vi "Results_file_Plotter.vi"() -> ()   [LabVIEW 2010]
uses:
  Anemometry/Anemometry Sub Vis/Data_plotting_vis/Plot_Slice.ctl
  Anemometry/Anemometry Sub Vis/Data_plotting_vis/Plotter_Mode.ctl
  Anemometry/Anemometry Sub Vis/Data_plotting_vis/Data_File_Type.ctl
  Anemometry/Anemometry Sub Vis/File/Setup_Filetype.ctl
  Anemometry/Anemometry Sub Vis/Controls/Global_mode.ctl
  Anemometry/Anemometry Sub Vis/Data_plotting_vis/Results_plotter_Global.vi
  Anemometry/Anemometry Sub Vis/Globals/Trav_pos_global.vi
  Anemometry/Anemometry Sub Vis/Globals/Constants_global.vi
  Instance           1 28Saved   Results_file_Plotter .vi
panel:
  in  "Single Series":i32[](listbox)=[0]
  out "Uadvec":dbl
  in  "Bkgnd Value":dbl
  in  "Update":bool
  in  "Full_Res_Results_Folder":path
  out "Last used Template":path
  out "Cursor index":i32
  in  "Plot Resolution":bool
  out "Choosen Path":path
  out "XY Plot":cluster{dbl[], dbl[]}[](graph)
  in  "VI Refnum Calculation":refnum<vi>
  in  "Save Plot as jpg":bool
  out "Edit Raw Data Header Info":bool
  out "Raw DF in Orig Pos?":bool
  out "Edit Raw DF?":bool
  out "Filetype":string[](array[string])
  out "Mode":T1
  out "Plotted rows only?":bool
  in  "type specifier VI Refnum (for type only) 2":refnum<vi>
  out "Warning!":string
  in  "Edit Template File":bool
  in  "type specifier VI Refnum (for type only)":refnum<vi>
  in  "color and symbol":bool
  out "No Of Rows":i32
  in  "Filter Bins 2":i32[](listbox)=[0]
  in  "Filter 6":u16(ring)
  in  "Filter 5":u16(ring)
  in  "Filter 4":u16(ring) items=["Show All (1216)", "10 (200)", "11 (4)", "13 (4)", "16 (4)", "17 (4)", "20 (12)", "23 (4)", "25 (4)", "28 (4)", "29 (4)", "30 (4)", "31 (4)", "35 (4)", "37 (4)", "38 (4)", "40 (8)", "44 (4)", "45 (8)", "47 (4)", "49 (4)", "50 (192)", "51 (4)", "53 (8)", "54 (4)", "56 (4)", "60 (12)", "63 (4)", "65 (4)", "67 (4)", "71 (8)", "72 (4)", "75 (4)", "78 (4)", "79 (4)", "81 (4)", "82 (4)", "85 (4)", "87 (4)", "90 (12)", "94 (4)", "97 (12)", "99 (4)", "100 (188)", "101 (8)", "103 (4)", "104 (4)", "106 (8)", "110 (4)", "111 (4)", "112 (4)", "115 (4)", "116 (4)", "119 (4)", "121 (8)", "125 (4)", "126 (4)", "128 (8)", "134 (12)", "137 (4)", "139 (4)", "141 (4)", "143 (4)", "144 (4)", "146 (8)", "148 (8)", "149 (4)", "150 (188)", "151 (4)", "153 (8)", "155 (4)", "156 (8)", "160 (4)", "162 (4)", "163 (4)", "164 (4)", "165 (4)", "171 (8)", "172 (4)", "173 (4)", "178 (8)", "181 (4)", "182 (4)", "185 (8)", "191 (8)", "193 (8)", "200 (16)"]
  in  "Filter 3":u16(ring) items=["Show All (1216)", "92 (1216)", "NOT 92 (0)"]
  in  "Filter Array":u16[](array[ring])=[0, 0, 0, 0, 0, 0] items=["Don't Filter", "Filename", "Case", "Roof Height", "Tank Height", "Release Angle", "X", "Y", "Z", "Y (FFID2)", "Z (FFID2)", "Mean Concentration (C)", "Variance in Concentration (C)", "Mean Concentration (C0)", "Variance in Concentration (C0)", "Standard Error in Mean C", "Background Mean Concentration", "Variance in Background Concentration", "CU/Q", "CU/Q err", "x/H", "y/H", "z/H", "Qtrace", "Uref", "Flow Measurement Time", "Seconds since 1st Jan", "Atmos Pressure Used for Corrections", "Current File Number", "Correlation coefficient", "Calib File", "Correlation", "Emission Rate", "Raw Data Filename"]
  in  "Filter Bins 1":i32[](listbox)=[0]
  in  "Tab Control":T2(tab)=enum."Save "
  in  "Reload Files":bool
  in  "Template":path
  in  "Empty":bool
  in  "Result files to read":path[](array[path])
  in  "Add results file":bool
  in  "File Tyoes to Read":T3
  in  "Vector Plot?":bool
  in  "Ordinate Name":string
  out "2nd Add label":string
  out "First Add label":string
  in  "Additional X Values":dbl[](array[numeric]) format="%.2f"
  in  "Additional Y Values":dbl[](array[numeric]) format="%.2f"
  in  "Show Results Space Analysis":bool
  in  "Show Plot Space Analysis":bool
  in  "Multi Ordinate":i32[](listbox)
  in  "Multi Ordinate?":bool
  in  "Ordinate":u16(ring) items=["Filename", "Case", "Roof Height", "Tank Height", "Release Angle", "X", "Y", "Z", "Y (FFID2)", "Z (FFID2)", "Mean Concentration (C)", "Variance in Concentration (C)", "Mean Concentration (C0)", "Variance in Concentration (C0)", "Standard Error in Mean C", "Background Mean Concentration", "Variance in Background Concentration", "CU/Q", "CU/Q err", "x/H", "y/H", "z/H", "Qtrace", "Uref", "Flow Measurement Time", "Seconds since 1st Jan", "Atmos Pressure Used for Corrections", "Current File Number", "Correlation coefficient", "Calib File", "Correlation", "Emission Rate", "Raw Data Filename"]
  in  "Intensity Plot?":bool
  in  "Absisca":u16(ring) items=["Filename", "Case", "Roof Height", "Tank Height", "Release Angle", "X", "Y", "Z", "Y (FFID2)", "Z (FFID2)", "Mean Concentration (C)", "Variance in Concentration (C)", "Mean Concentration (C0)", "Variance in Concentration (C0)", "Standard Error in Mean C", "Background Mean Concentration", "Variance in Background Concentration", "CU/Q", "CU/Q err", "x/H", "y/H", "z/H", "Qtrace", "Uref", "Flow Measurement Time", "Seconds since 1st Jan", "Atmos Pressure Used for Corrections", "Current File Number", "Correlation coefficient", "Calib File", "Correlation", "Emission Rate", "Raw Data Filename"]
  in  "Job Directory":path
  in  "Save Averaged rows":bool
  in  "Create picture Vi Name":string="Intensity plot jpg.vi"
  in  "Save Surface Fit":bool
  in  "Output Filename":path
  in  "Save Data in Rows":bool
  in  "Save Plot data":bool
  in  "Process Point":bool
  in  "Kill Point":bool
  out "Table":string[][](table)
  in  "Post Process Plotted Data":bool
  in  "Calculate Routine":string="Intensity plot jpg.vi"
  in  "Calculate new metadata":bool
  in  "Add /Edit metadata":bool
  in  "Delete Plotted data from file":bool
  in  "Save Setup":bool
  in  "Load Setup":bool
  in  "Point Size":i32(slide) scale=0.0..10.0
  in  "No of Contours":i32=20
  out "Accept Array":bool[][](array[boolean])
  out "Previous slice mode":T4
  out "Slice mode Change?":bool
  in  "Slice mode":T4
  in  "Z Ch Name":u16(ring) items=["Filename", "Case", "Roof Height", "Tank Height", "Release Angle", "X", "Y", "Z", "Y (FFID2)", "Z (FFID2)", "Mean Concentration (C)", "Variance in Concentration (C)", "Mean Concentration (C0)", "Variance in Concentration (C0)", "Standard Error in Mean C", "Background Mean Concentration", "Variance in Background Concentration", "CU/Q", "CU/Q err", "x/H", "y/H", "z/H", "Qtrace", "Uref", "Flow Measurement Time", "Seconds since 1st Jan", "Atmos Pressure Used for Corrections", "Current File Number", "Correlation coefficient", "Calib File", "Correlation", "Emission Rate", "Raw Data Filename"]
  in  "Y Ch Name":u16(ring) items=["Filename", "Case", "Roof Height", "Tank Height", "Release Angle", "X", "Y", "Z", "Y (FFID2)", "Z (FFID2)", "Mean Concentration (C)", "Variance in Concentration (C)", "Mean Concentration (C0)", "Variance in Concentration (C0)", "Standard Error in Mean C", "Background Mean Concentration", "Variance in Background Concentration", "CU/Q", "CU/Q err", "x/H", "y/H", "z/H", "Qtrace", "Uref", "Flow Measurement Time", "Seconds since 1st Jan", "Atmos Pressure Used for Corrections", "Current File Number", "Correlation coefficient", "Calib File", "Correlation", "Emission Rate", "Raw Data Filename"]
  in  "X Ch Name":u16(ring) items=["Filename", "Case", "Roof Height", "Tank Height", "Release Angle", "X", "Y", "Z", "Y (FFID2)", "Z (FFID2)", "Mean Concentration (C)", "Variance in Concentration (C)", "Mean Concentration (C0)", "Variance in Concentration (C0)", "Standard Error in Mean C", "Background Mean Concentration", "Variance in Background Concentration", "CU/Q", "CU/Q err", "x/H", "y/H", "z/H", "Qtrace", "Uref", "Flow Measurement Time", "Seconds since 1st Jan", "Atmos Pressure Used for Corrections", "Current File Number", "Correlation coefficient", "Calib File", "Correlation", "Emission Rate", "Raw Data Filename"]
  out "Filter 2 Strings":string[](array[string])
  out "Filter 1 Strings":string[](array[string])
  out "Ordinate Strings":string[](array[string])
  out "Non-Blank Rows":bool[](array[boolean])
  out "File Index":i32
  in  "Resolution":dbl=1.0 min=0.0 format="%.4f"
  out "Intensity Graph":dbl[][](graph)
  out "Tolerances":dbl[](array[numeric]) format="%.2f"
  in  "Results files choosen":path[](array[path])
  in  "Header":string
  out "Current":string="Graph Scales"
  in  "Transpose":bool
  out "Plotted Series":bool[][](array[boolean])
  in  "Results file":path
  in  "stop":bool
  out "Surface Area":dbl format="%.2f"
  out "Surface Integral":dbl format="%.4f"
  out "Surface Average":dbl format="%#.5f"
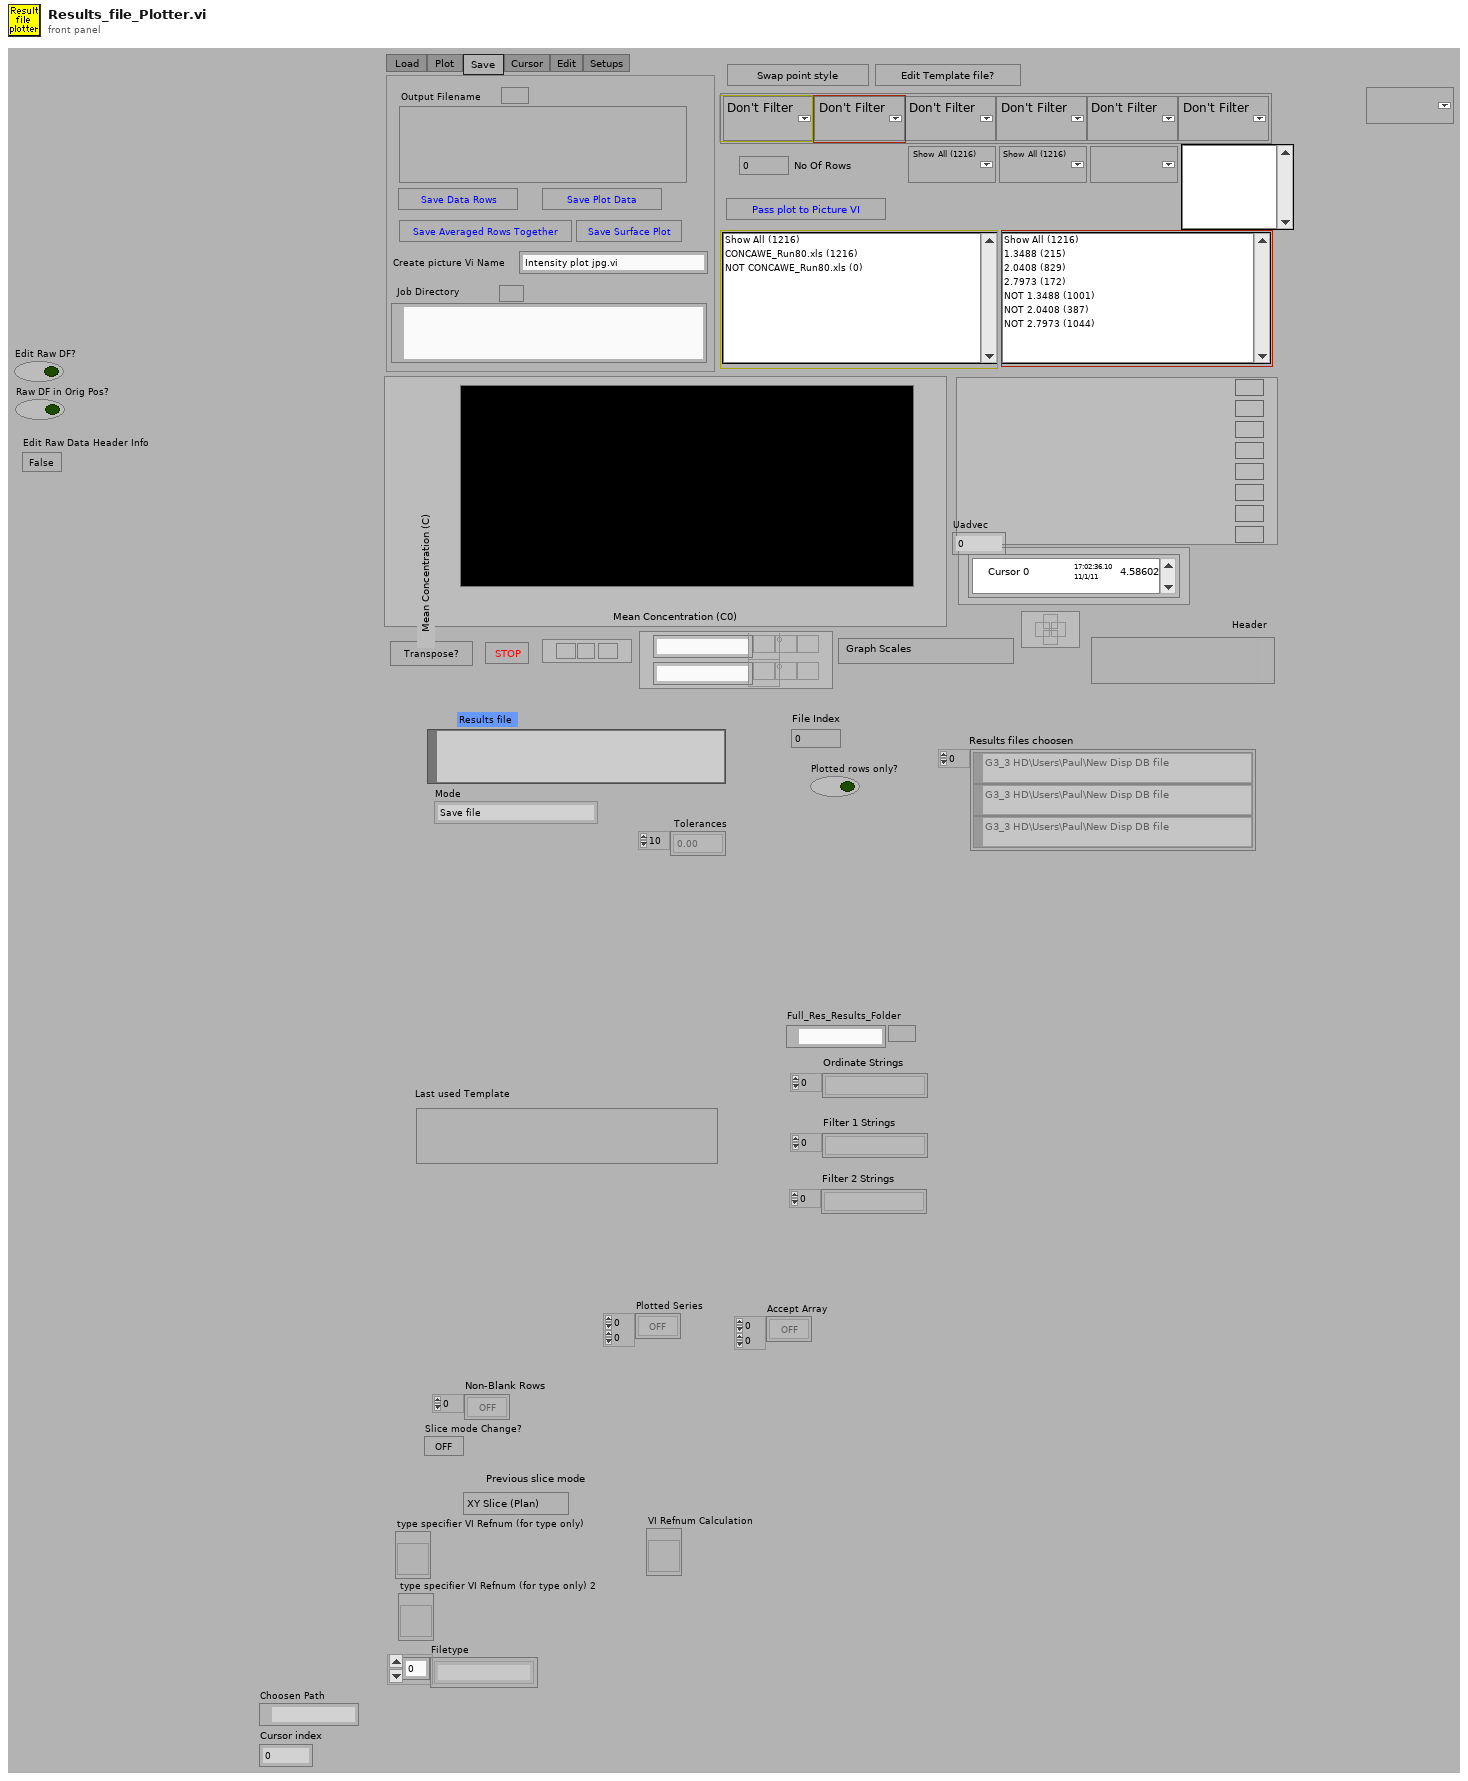
[diagram p1: front panel]
types:
  T1 = typedef "Plotter_Mode.ctl" = enum16{"Save file", "Delete unwanted rows", "Edit Values with constants", "Edit values per row", "Edit Raw Data file header", "Post Process Plotted Rows"}
  T2 = enum32{"Load ", "Plot ", "Save ", "Cursor", "Edit", "Setups"}
  T3 = typedef "Data_File_Type.ctl" = enum16{"Read All File Types", "Results Files Only", "Raw Data Files Only", "Calibration Files Only", "Gas Desk Files Only", "Old Results Files Only", "Tabulated Data Files Only"}
  T4 = typedef "Plot_Slice.ctl" = enum16{"XY Slice (Plan)", "YX Slice (Plan)", "YZ Slice (Cross)", "ZY Slice (Cross)", "XZ Slice (Side)", "ZX Slice (Side)"}
  T5 = typedef "Setup_Filetype.ctl" = enum16{"Measurement Setups", "Calibration Setups", "General", "Results File Plotter Setups", "Speed Calib Tweaks"}
  T6 = enum16{"Zero or one", "One", "Zero or more", "One or more"}
  T7 = typedef "Global_mode.ctl" = enum16{"Read Global", "Load Global From File", "Write Global to File"}
  T8 = enum16{"Edit Existing Template File", "Create New Template File"}
  T9 = enum16{"Show only data summary", "Show data summary", "No data summary"}
  T10 = typedef "All_Setup.ctl" = cluster{"Result files to read":path[], "Template":path, "Transpose":bool, "Additional X Values":dbl[], "Additional Y Values":dbl[], "Ordinate":u16, "Absisca":u16, "Filter Array":u16[], "color and symbol":bool, "Output Filename":path, "Jpg Vi Name":string, "Intensity Plot?":bool, "Multi Ordinate?":bool, "Filter Bins 1":i32[], "Filter Bins 2":i32[], "Multi Ordinate":i32[]}
  T11 = enum16{"Left Button", "Center Button", "Right Button", "Window Close"}
  T12 = enum32{"existing file", "new file", "new or existing file", "existing dir", "new dir", "new or existing dir", "existing file (use LLBs)", "new file (use LLBs)", "new or existing file (use LLBs)", "new or existing file or directory (use LLBs)"}
  T13 = cluster{"Plot Color":u32, "Plot Interpolation":u8, "Point Style":u8, "Line Style":u8, "Fill/Pt. Color":u32, "Line Width":u8, "Bar Plot Style":u8, "Fill To":i16}[]
  T14 = typedef "Group_Binning.ctl" = cluster{"Index":i32, "Tolerance":dbl, "Precision":string}
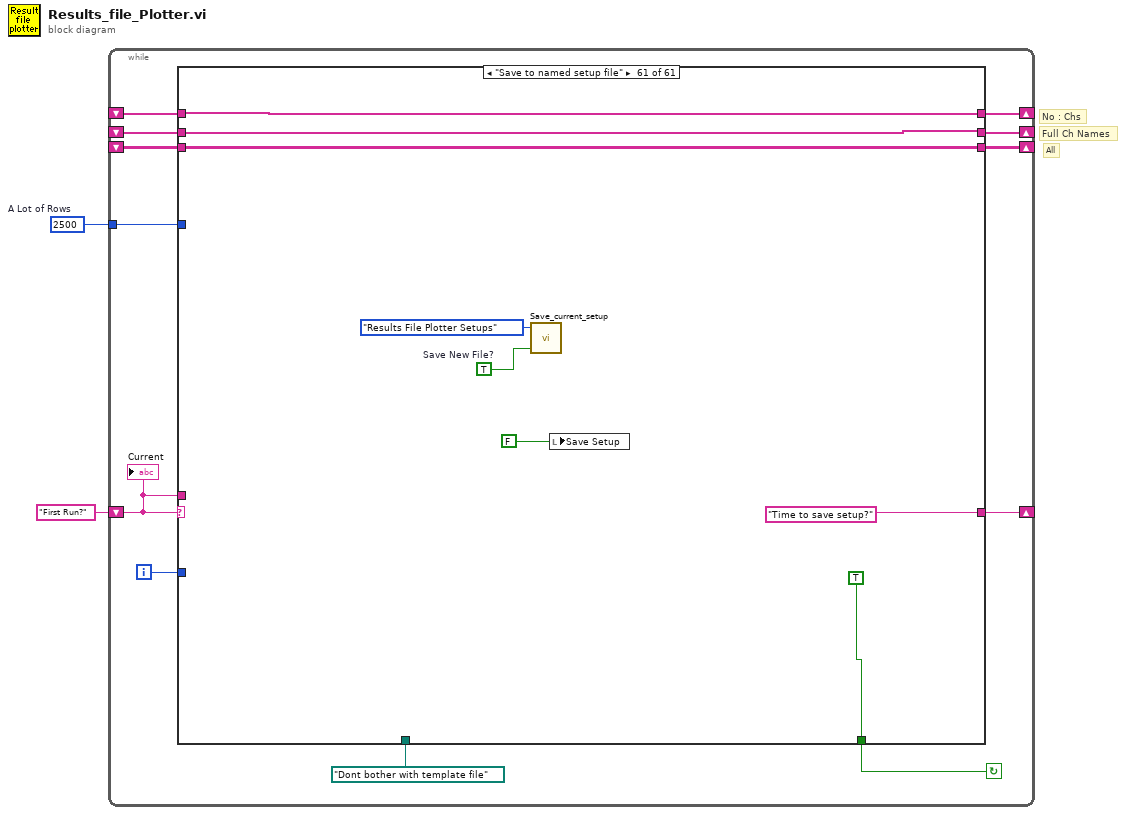
[diagram p0: block diagram]
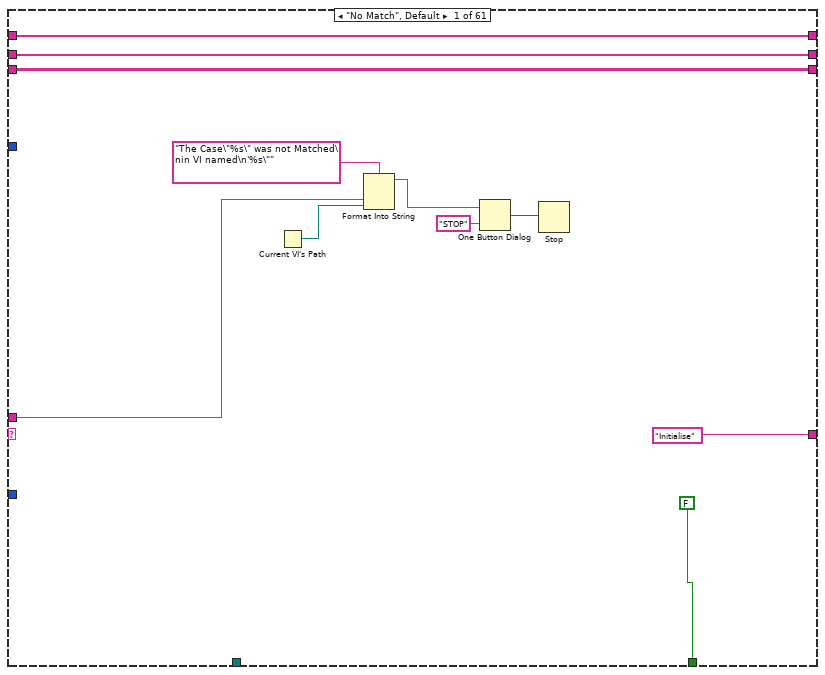
[diagram p2: hidden frame]
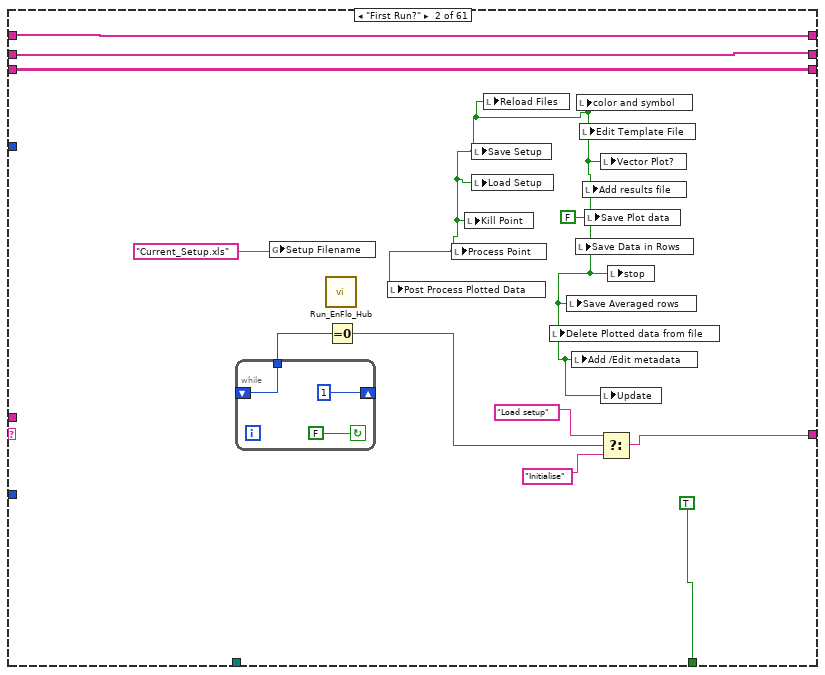
[diagram p3: hidden frame]
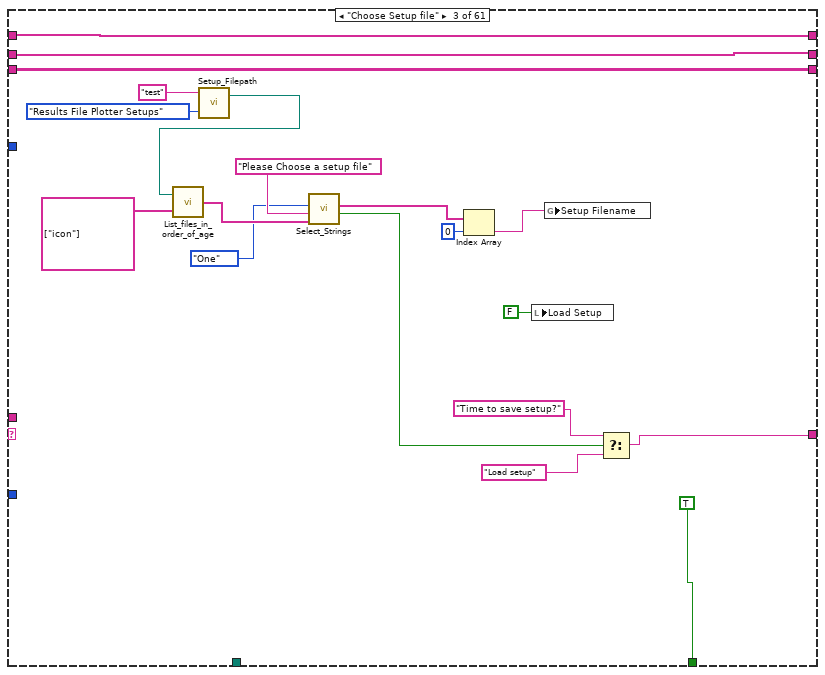
[diagram p4: hidden frame]
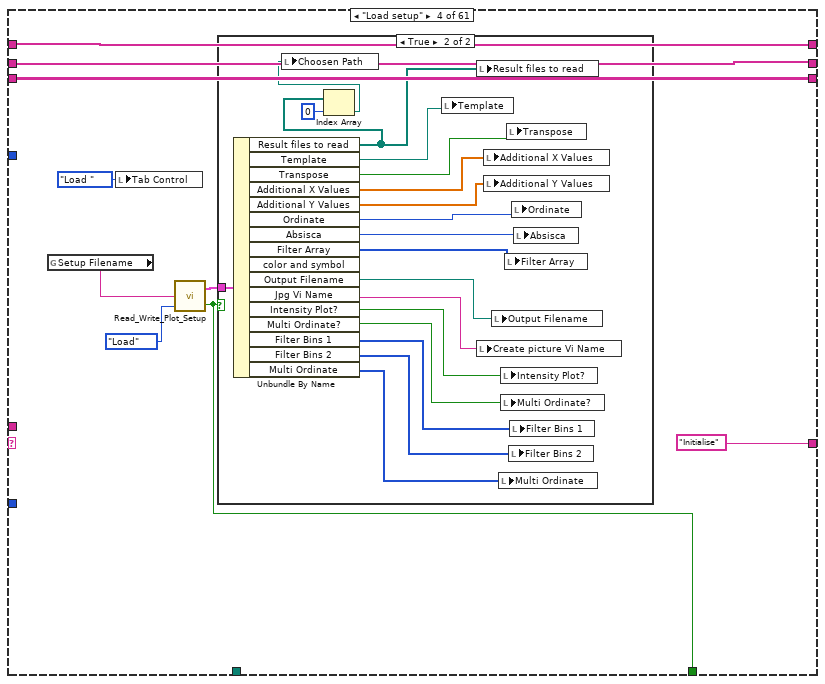
[diagram p5: hidden frame]
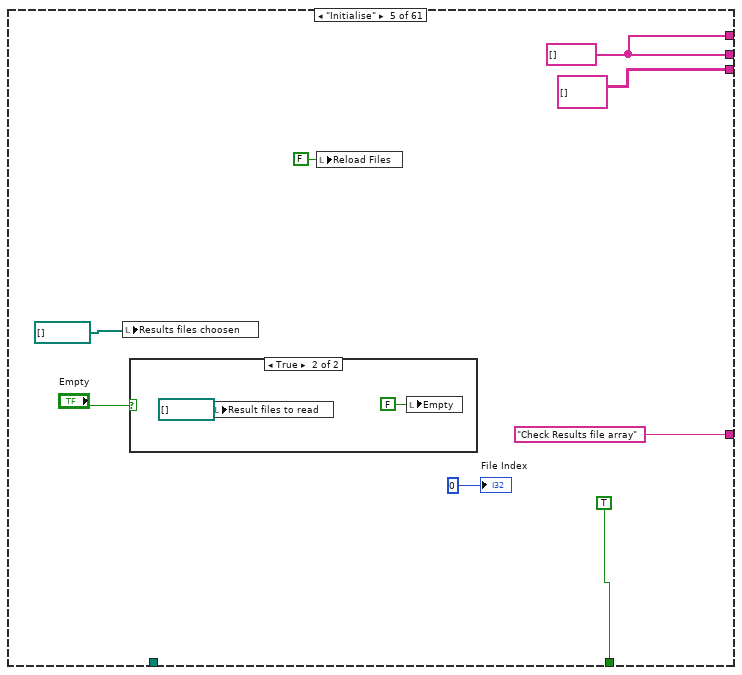
[diagram p7: hidden frame]
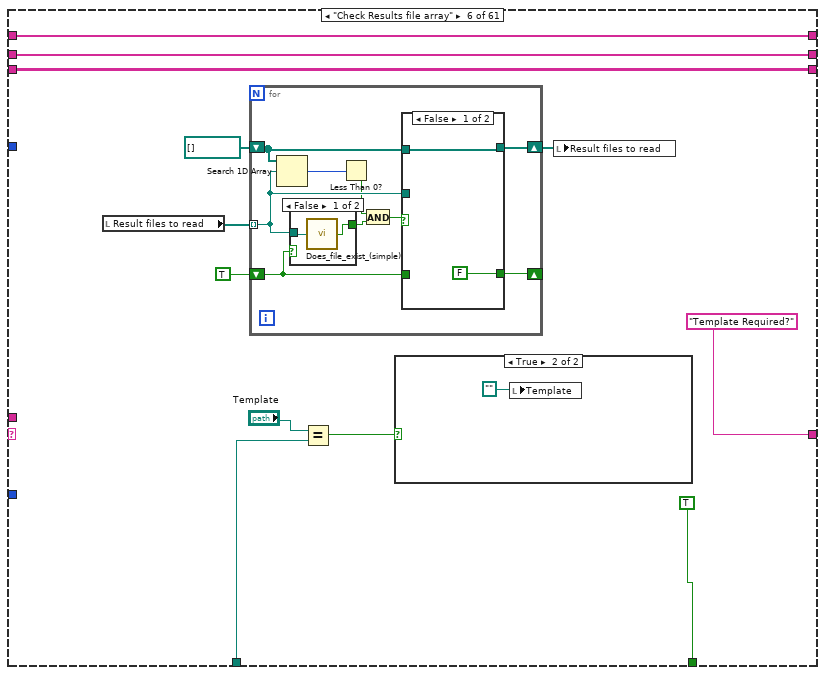
[diagram p9: hidden frame]
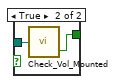
[diagram p11: hidden frame]
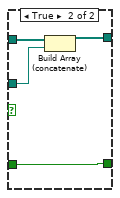
[diagram p12: hidden frame]
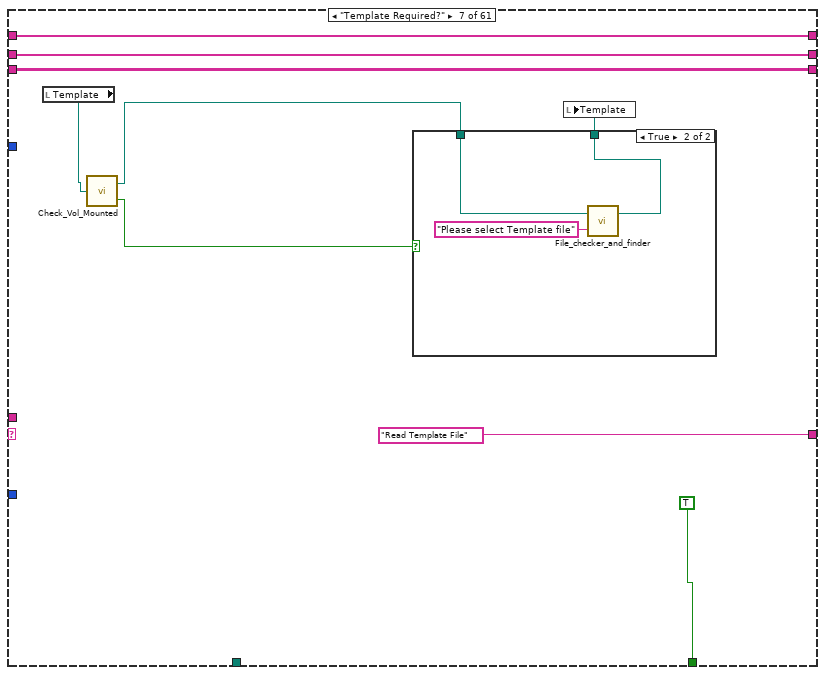
[diagram p13: hidden frame]
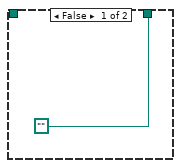
[diagram p14: hidden frame]
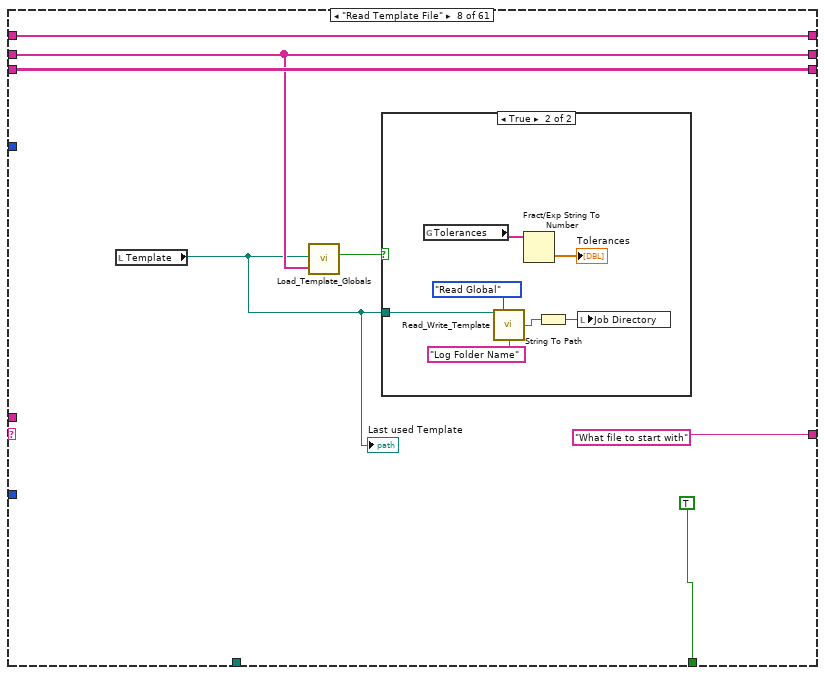
[diagram p15: hidden frame]
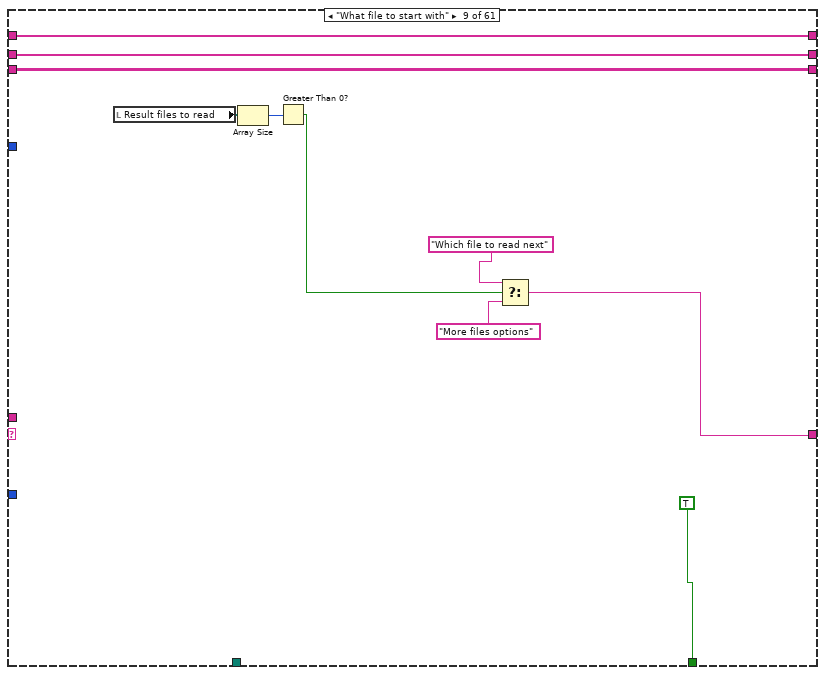
[diagram p17: hidden frame]
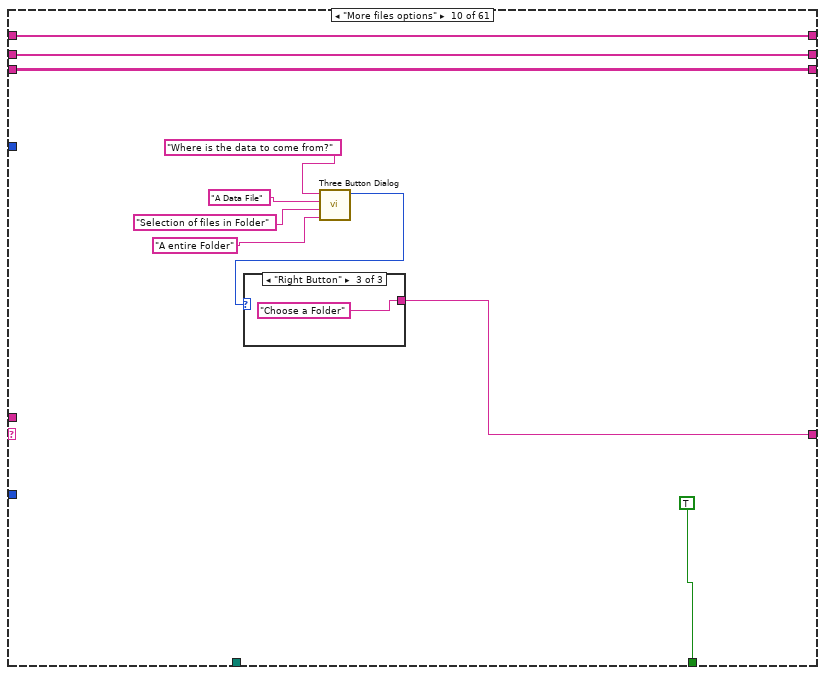
[diagram p18: hidden frame]
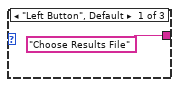
[diagram p19: hidden frame]
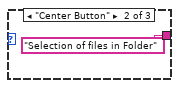
[diagram p20: hidden frame]
diagram:
  w1 = 2500  # A Lot of Rows
  # "No : Chs"
  # "Full Ch Names"
  # "All"
  n1 = while {
    shift-left: _ -> [w7]
    shift-right: [w8] -> _
    shift-left: "First Run?" -> [w11]
    shift-right: [w4] -> _
    shift-left: _ -> [w9]
    shift-right: [w14] -> _
    shift-left: _ -> [w12]
    shift-right: [w5] -> _
    tunnel: w1 -> [w3]
    i -> [w6]
    stop <- w13 continue-if-true
    n2 = case shown="\"Save to named setup file\"" w11 {
      tunnel: w9 -> [w25 w35 w57 w65 _ w106 w134 w143 w164 w174 w186 w200 w231 w258 w281 w403 w425 w451 w476 w502 w556 w570 w607 w909 w978 w1033 w1058 w1077 w1163 w1211 w1241 w1530 w1546 w1567 w1596 w1660 w1693 w1765 w1788 w1803 w1867 w1919 w1945 w2154 w2166 w2192 w2318 w2462 w2496 w2511 w2536 w2563 w2606 w2624 w2667 w2770 w2803 w3167 w3182 w3218 w3226]
      tunnel: [w25 w35 w57 w65 w91 w106 w134 w143 w164 w174 w186 w200 w231 w258 w279 w403 w425 w451 w476 w502 w556 w570 w607 w909 w978 w1033 w1058 w1077 w1163 w1211 w1239 w1530 w1546 w1567 w1596 w1660 w1693 w1765 w1788 w1803 w1867 w1919 w1943 w2154 w2166 w2190 w2311 w2462 w2496 w2511 w2536 w2563 w2606 w2624 w2667 w2770 w2803 w3167 w3182 w3218 w3226] -> w14
      tunnel: ["Initialise" w28 w52 "Initialise" ("t") "Check Results file array" ("t") "Template Required?" "Read Template File" "What file to start with" w155 w170 "Which file to read next" "Which file to read next" "Which file to read next" w254 w276 w394 "What is present?" "Ordinate Selector Type" w473 "Which rows are Non-Blank?" w549 "Create Selectors" w596 "Re Plot Data?" w973 "Prepare Filter2 strings" "Plot Data" w1074 "Add Axis names" "Analyse Plot Space" w1242 "What to do next?" "What to do next?" ("t") w1553 w1589 w1638 w1691 w1759 w1784 w1802 w1866 "Initialise" w1946 w2145 "Create Selectors" w2193 w2319 w2460 w2494 w2501 w2520 "Save XY plot as jpg" "Create Selectors" w2621 w2670 w2754 w2809 "Save Setup" ("t") "Initialise" ("t") w3187 "Time to save setup?"] -> w4
      tunnel: [FALSE TRUE TRUE w61 TRUE TRUE TRUE TRUE TRUE TRUE TRUE TRUE TRUE w249 w283 TRUE TRUE TRUE TRUE TRUE TRUE TRUE TRUE TRUE TRUE TRUE TRUE w1075 TRUE TRUE w1243 TRUE TRUE ("OK?") TRUE TRUE ("OK?") TRUE ("OK?") w1689 TRUE TRUE w1801 w1865 TRUE w1947 TRUE ("OK?") TRUE ("OK?") w2194 w2320 TRUE TRUE TRUE TRUE TRUE TRUE TRUE TRUE TRUE TRUE TRUE TRUE w3196 TRUE ("OK?")] -> w13
      tunnel: w12 -> [w24 w34 w56 w64 _ w105 w133 w145 w163 w173 w185 w199 w230 w257 w282 w399 w424 w452 w477 w503 w555 w568 w602 w911 w967 w1035 w1060 w1076 w1165 w1213 w1240 w1529 w1545 w1566 w1607 w1659 w1692 w1764 w1787 w1800 w1864 w1918 w1944 w2153 w2163 w2191 w2317 w2463 w2495 w2510 w2540 w2566 w2605 w2623 w2666 w2769 w2802 w3166 w3181 w3217 w3225]
      tunnel: w11 -> [w16 _ _ _ _ _ _ _ _ _ _ _ _ _ _ _ _ _ _ _ _ _ _ _ _ _ _ _ _ _ _ _ _ _ _ _ _ _ _ _ _ _ _ _ _ _ _ _ _ _ _ _ _ _ _ _ _ _ _ _ _]
      tunnel: path "Dont bother with template file" ("Template File") -> [_ _ _ _ _ w99 _ _ _ _ _ _ _ _ _ _ _ _ _ _ _ _ _ _ _ _ _ _ _ _ _ _ _ _ _ _ _ _ _ _ _ _ _ _ _ _ _ _ _ _ _ _ _ _ _ _ _ w3164 w3176 _ _]
      tunnel: [w15 w33 w55 w66 w91 w104 w132 w144 w161 w171 w183 w197 w228 w256 w278 w387 w423 w453 w475 w501 w547 w569 w600 w908 w969 w1025 w1053 w1073 w1157 w1206 w1235 w1526 w1547 w1565 w1597 w1661 w1694 w1763 w1786 w1799 w1863 w1917 w1937 w2155 w2171 w2181 w2314 w2472 w2497 w2512 w2537 w2564 w2607 w2625 w2671 w2771 w2810 w3168 w3183 w3219 w3227] -> w8
      tunnel: w7 -> [w15 w33 w55 w66 _ w104 w132 w144 w161 w171 w183 w197 w228 w256 w277 w387 w423 w453 w475 w501 w547 w569 w600 w908 w969 w1025 w1053 w1073 w1157 w1206 w1234 w1526 w1547 w1565 w1597 w1661 w1694 w1763 w1786 w1799 w1863 w1917 w1936 w2155 w2171 w2185 w2313 w2472 w2497 w2512 w2537 w2564 w2607 w2625 w2671 w2771 w2810 w3168 w3183 w3219 w3227]
      tunnel: w6 -> [_ _ _ _ _ _ _ _ _ _ _ _ _ _ _ _ _ _ _ _ _ _ _ _ _ _ _ _ _ _ _ _ _ _ _ _ w1690 _ _ _ _ _ _ _ _ _ _ _ _ _ _ _ _ _ _ _ _ _ _ _ _]
      tunnel: [w24 w34 w56 w64 string[][] [] w105 w133 w145 w163 w173 w185 w199 w230 w257 w280 w399 w424 w452 w477 w503 w555 w568 w602 w911 w967 w1035 w1060 w1076 w1165 w1213 w1238 w1529 w1545 w1566 w1607 w1659 w1692 w1764 w1787 w1800 w1864 w1918 w1942 w2153 w2163 w2189 w2310 w2463 w2495 w2510 w2540 w2566 w2605 w2623 w2666 w2769 w2802 w3166 w3181 w3217 w3225] -> w5
      tunnel: w3 -> [_ _ _ _ _ _ _ _ _ _ _ _ _ _ _ _ _ _ _ _ _ _ _ _ _ _ _ _ _ _ _ _ _ _ _ _ _ _ w1782 _ w1862 _ _ _ _ _ _ _ _ _ _ _ _ w2620 w2664 _ w2800 _ _ _ _]
      frame "No Match", Default {
        n3 = Current VI's Path() -> (path=w17:path)
        n4 = Format Into String(format string="The Case\"%s\" was not Matched\nin VI named\n'%s\"" ("Format String"), w16, w17) -> (resulting string=w20:string)  [unwired: 2 in, 1 out]
        n5 = One Button Dialog(message=w20, button name ("OK")="STOP") -> (true=w18:bool)
        n6 = Stop(stop? (T)=w18) -> ()
      }
      frame "First Run?" {
        w26 = FALSE ("Save Plot data")
        n7 = while {
          shift-right: [1] -> _
          shift-left: _ -> [w38]
          tunnel: [w38] -> w30
          stop <- FALSE continue-if-true
        }
        n8 = global write "Results_plotter_Global.vi" "Setup Filename"("Current_Setup.xls" ("Setup filename")) -> ()
        n9 = call "Run_EnFlo_Hub.vi"() -> ()  [unwired: 8 out]
        n10 = Equal To 0?(x=w30) -> (x = 0?=w29:bool)
        n11 = local write "Post Process Plotted Data"(w26) -> ()
        n12 = local write "Process Point"(w26) -> ()
        n13 = local write "Kill Point"(w26) -> ()
        n14 = local write "Save Setup"(w26) -> ()
        n15 = local write "Load Setup"(w26) -> ()
        n16 = local write "Reload Files"(w26) -> ()
        n17 = local write "Delete Plotted data from file"(w26) -> ()
        n18 = local write "Save Averaged rows"(w26) -> ()
        n19 = local write "Add /Edit metadata"(w26) -> ()
        n20 = local write "Save Data in Rows"(w26) -> ()
        n21 = local write "color and symbol"(w26) -> ()
        n22 = local write "Edit Template File"(w26) -> ()
        n23 = local write "Add results file"(w26) -> ()
        n24 = local write "Save Plot data"(w26) -> ()
        n25 = local write "Vector Plot?"(w26) -> ()
        n26 = local write "Update"(w26) -> ()
        n27 = Select(t="Load setup", s=w29, f="Initialise") -> (s? t:f=w28:string)
        n28 = local write "stop"(w26) -> ()
      }
      frame "Choose Setup file" {
        n29 = call "Setup_Filepath.vi"("Setup File Type"=Setup_Filetype."Results File Plotter Setups", "Filename in"="test") -> ("Directory"=w40:path)  [unwired: 1 out]
        n30 = call "List_files_in_order_of_age.vi"("Files to Hide"=string[] ["icon"], "Folder"=w40) -> ("file names"=w51:string[])
        n31 = call "Select_Strings.vi"("Available Ch names"=w51, "Message"="Please Choose a setup file", "Selector mode"=T6."One") -> ("Cancel"=w45:bool, "Selected Channel Names"=w48:string[])  [unwired: 1 in, 3 out]
        n32 = Index Array(array=w48, index=0) -> (element=w46:string)
        n33 = local write "Load Setup"(FALSE ("Save Setup")) -> ()
        n34 = global write "Results_plotter_Global.vi" "Setup Filename"(w46) -> ()
        n35 = Select(t="Time to save setup?", s=w45, f="Load setup") -> (s? t:f=w52:string)
      }
      frame "Load setup" {
        n36 = global read "Results_plotter_Global.vi" "Setup Filename"() -> (w60:string)
        n37 = local write "Tab Control"(T2."Load " ("Tab Control")) -> ()
        n38 = call "Read_Write_Plot_Setup.vi"("Mode"=enum16{"Load", "Save"}."Load", "Setup filename"=w60) -> ("OK?"=w61:bool, "Cluster 2"=w62:T10)  [unwired: 1 in]
        n39 = case shown="True" w61 {
          tunnel: w62 -> [_ w85]
          frame False {
          }
          frame True {
            n40 = Unbundle By Name(w85) -> ("Result files to read"=w70:path[], "Template"=w68:path, "Transpose"=w75:bool, "Additional X Values"=w76:dbl[], "Additional Y Values"=w77:dbl[], "Ordinate"=w78:u16, "Absisca"=w79:u16, "Filter Array"=w80:u16[], "Output Filename"=w81:path, "Jpg Vi Name"=w82:string, "Intensity Plot?"=w83:bool, "Multi Ordinate?"=w84:bool, "Filter Bins 1"=w74:i32[], "Filter Bins 2"=w73:i32[], "Multi Ordinate"=w72:i32[])  [unwired: 1 out]
            n41 = Index Array(array=w70, index=0) -> (element=w69:path)
            n42 = local write "Choosen Path"(w69) -> ()
            n43 = local write "Template"(w68) -> ()
            n44 = local write "Result files to read"(w70) -> ()
            n45 = local write "Create picture Vi Name"(w82) -> ()
            n46 = local write "Additional X Values"(w76) -> ()
            n47 = local write "Additional Y Values"(w77) -> ()
            n48 = local write "Output Filename"(w81) -> ()
            n49 = local write "Multi Ordinate"(w72) -> ()
            n50 = local write "Intensity Plot?"(w83) -> ()
            n51 = local write "Multi Ordinate?"(w84) -> ()
            n52 = local write "Filter Array"(w80) -> ()
            n53 = local write "Transpose"(w75) -> ()
            n54 = local write "Filter Bins 2"(w73) -> ()
            n55 = local write "Filter Bins 1"(w74) -> ()
            n56 = local write "Ordinate"(w78) -> ()
            n57 = local write "Absisca"(w79) -> ()
          }
        }
      }
      frame "Initialise" {
        w91 = string[] [] ("Channel names")
        n58 = local write "Results files choosen"(path[] [] ("Results file choosen")) -> ()
        n59 = case shown="True" "Empty" {
          frame False {
          }
          frame True {
            n60 = local write "Result files to read"(path[] [] ("Result files to read")) -> ()
            n61 = local write "Empty"(FALSE ("Empty")) -> ()
          }
        }
        n62 = local write "Reload Files"(FALSE ("Reload Files")) -> ()
        "File Index" <- 0
      }
      frame "Check Results file array" {
        n63 = local read "Result files to read"() -> (w103:path[])
        n64 = for {
          shift-right: [w117] -> w101
          shift-left: path[] [] -> [w116]
          tunnel: w103 -> [w115] mode=indexing
          shift-right: [w110] -> _
          shift-left: TRUE -> [w109]
          n65 = Search 1D Array(1D array=w116, element=w115) -> (index of element=w114:i32)  [unwired: 1 out]
          n66 = case shown="False" w109 {
            tunnel: w115 -> [w119 w121]
            tunnel: [w118 w120] -> w112
            frame False {
              n67 = call "Does_file_exist_(simple).vi"("Pathname"=w119) -> ("exists?"=w118:bool)
            }
            frame True {
              n68 = call "Check_Vol_Mounted.vi"("Filename"=w121) -> ("exists?"=w120:bool)  [unwired: 1 out]
            }
          }
          n69 = Less Than 0?(x=w114) -> (x < 0?=w111:bool)
          n70 = And(x=w111, y=w112) -> (x .and. y?=w113:bool)
          n71 = case shown="False" w113 {
            tunnel: w116 -> [w123 w127]
            tunnel: w115 -> [_ w126]
            tunnel: [w123 w125] -> w117
            tunnel: [FALSE w124] -> w110
            tunnel: w109 -> [_ w124]
            frame False {
            }
            frame True {
              n72 = Build Array (concatenate)(w127, w126) -> (w125:path[])
            }
          }
        }
        n73 = Equal?(x="Template", y=w99) -> (x = y?=w98:bool)
        n74 = case shown="True" w98 {
          frame False {
          }
          frame True {
            n75 = local write "Template"(path "") -> ()
          }
        }
        n76 = local write "Result files to read"(w101) -> ()
      }
      frame "Template Required?" {
        n77 = local read "Template"() -> (w131:path)
        n78 = call "Check_Vol_Mounted.vi"("Filename"=w131) -> ("Filename Out"=w130:path, "exists?"=w129:bool)
        n79 = case shown="True" w129 {
          tunnel: w130 -> [_ w139]
          tunnel: [path "" w138] -> w128
          frame False {
          }
          frame True {
            n80 = call "File_checker_and_finder.vi"("Promp if not found"="Please select Template file", "Filename In"=w139) -> ("Filename Out"=w138:path)  [unwired: 1 out]
          }
        }
        n81 = local write "Template"(w128) -> ()
      }
      frame "Read Template File" {
        n82 = local read "Template"() -> (w141:path)
        "Last used Template" <- w141
        n83 = call "Load_Template_Globals.vi"("Channel Names"=w143, "Template-read"=w141) -> ("Valid Template File?"=w142:bool)
        n84 = case shown="True" w142 {
          tunnel: w141 -> [_ w149]
          frame False {
          }
          frame True {
            n85 = global read "Results_plotter_Global.vi" "Tolerances"() -> (w153:string[])
            n86 = call "Read_Write_Template.vi"("Template File"=w149, "Mode"=Global_mode."Read Global", "Data type"="Log Folder Name" ("Variable name")) -> ("Single Value Out"=w151:string)  [unwired: 5 in, 7 out]
            n87 = Fract/Exp String To Number(string=w153) -> (number=→"Tolerances":dbl[])  [unwired: 4 out]
            n88 = String To Path(string=w151) -> (path=w148:path)
            n89 = local write "Job Directory"(w148) -> ()
          }
        }
      }
      frame "What file to start with" {
        n90 = local read "Result files to read"() -> (w160:path[])
        n91 = Array Size(array=w160) -> (size(s)=w159:i32)
        n92 = Greater Than 0?(x=w159) -> (x > 0?=w156:bool)
        n93 = Select(t="Which file to read next", s=w156, f="More files options") -> (s? t:f=w155:string)
      }
      frame "More files options" {
        n94 = call <vilib>:"Three Button Dialog.vi"("Right Button Text (\"Cancel\")"="A entire Folder" ("F button name (\"Cancel\")"), "Center Button Text (\"No\")"="Selection of files in Folder" ("T button name (\"OK\")"), "Left Button Text (\"Yes\")"="A Data File" ("T button name (\"OK\")"), "message"="Where is the data to come from?") -> ("Which Button?"=w169:T11)  [unwired: 1 in, 6 out]
        n95 = case shown="\"Right Button\"" w169 {
          tunnel: ["Choose Results File" "Selection of files in Folder" "Choose a Folder"] -> w170
          frame "Left Button", Default {
          }
          frame "Center Button" {
          }
          frame "Right Button" {
          }
        }
      }
      frame "Choose Results File" {
        (unwired) T12."existing file" ("select mode (2)")
        n96 = local read "Choosen Path"() -> (w178:path)
        n97 = File Dialog(7:"Please Choose a Results File" ("Promp if not found"), 11:w178) -> (1:w180:bool, 3:w179:path)  [unwired: 1 in, 6 out]
        "Choosen Path" <- w179
        n98 = case shown="False" w180 {
          tunnel: w179 -> [w187 _]
          frame False {
            n99 = local read "Result files to read"() -> (w188:path[])
            n100 = Build Array (concatenate)(w188, w187) -> (w189:path[])
            n101 = local write "Result files to read"(w189) -> ()
          }
          frame True {
          }
        }
      }
      frame "Choose a Folder" {
        n102 = local read "Choosen Path"() -> (w191:path)
        n103 = File Dialog(7:"Please Choose the folder that contains the Results files to be plotted" ("prompt"), 11:w191) -> (3:w190:path)  [unwired: 1 in, 7 out]
        n104 = local write "Choosen Path"(w190) -> ()
        n105 = call "Get_folder_and_filenames.vi"("file path (dialog if empty)"=w190) -> ("Files"=w192:path[])  [unwired: 1 out]
        n106 = for {
          shift-right: [w211] -> w193
          shift-left: "Result files to read" -> [w210]
          tunnel: w192 -> [w208] mode=indexing
          n107 = Search 1D Array(1D array=w210, element=w208) -> (index of element=w209:i32)  [unwired: 1 out]
          n108 = Strip Path(path=w208) -> (name=w207:string)  [unwired: 1 out]
          n109 = Less Than 0?(x=w209) -> (x < 0?=w206:bool)
          n110 = call "Add_filename_suffix.vi"("Filename"=w207) -> ("Original Suffix"=w204:string)  [unwired: 1 in, 3 out]
          n111 = call "Match_Pat_Case_In.vi"("String to match"=".jpg" ("x"), "String"=w204) -> ("offset past match"=w202:i32)  [unwired: 1 in, 3 out]
          n112 = Less Than 0?(x=w202) -> (x < 0?=w201:bool)
          n113 = And(x=w206, y=w201) -> (x .and. y?=w205:bool)
          n114 = case shown="True" w205 {
            tunnel: w210 -> [w212 w215]
            tunnel: w208 -> [_ w214]
            tunnel: [w212 w213] -> w211
            frame False {
            }
            frame True {
              n115 = Build Array (concatenate)(w215, w214) -> (w213:path[])
            }
          }
        }
        n116 = local write "Result files to read"(w193) -> ()
      }
      frame "Selection of files in Folder" {
        n117 = local read "Choosen Path"() -> (w217:path)
        n118 = local read "Result files to read"() -> (w220:path[])
        n119 = File Dialog(7:"Please Choose the folder that contains the Results files to be plotted" ("prompt"), 11:w217) -> (3:w216:path)  [unwired: 1 in, 7 out]
        n120 = local write "Choosen Path"(w216) -> ()
        n121 = call "Get_folder_and_filenames.vi"("file path (dialog if empty)"=w216) -> ("Files"=w222:path[])  [unwired: 1 out]
        n122 = for {
          tunnel: w222 -> [w245] mode=indexing
          tunnel: [w244] -> w225 mode=indexing
          n123 = Strip Path(path=w245) -> (name=w244:string)  [unwired: 1 out]
        }
        n124 = call "Select_Strings.vi"("Available Ch names"=w225, "Message"="Please select the desired data files", "Selector mode"=T6."Zero or more") -> ("Ch Indicies Choosen"=w223:i32[])  [unwired: 1 in, 4 out]
        n125 = for {
          tunnel: w223 -> [w243] mode=indexing
          tunnel: w222 -> [w242]
          tunnel: [w241] -> w218 mode=indexing
          n126 = Index Array(array=w242, index=w243) -> (element=w241:path)
        }
        n127 = for {
          shift-right: [w236] -> w219
          shift-left: w220 -> [w235]
          tunnel: w218 -> [w234] mode=indexing
          n128 = Search 1D Array(1D array=w235, element=w234) -> (index of element=w233:i32)  [unwired: 1 out]
          n129 = Less Than 0?(x=w233) -> (x < 0?=w232:bool)
          n130 = case shown="True" w232 {
            tunnel: w235 -> [w237 w240]
            tunnel: w234 -> [_ w239]
            tunnel: [w237 w238] -> w236
            frame False {
            }
            frame True {
              n131 = Build Array (concatenate)(w240, w239) -> (w238:path[])
            }
          }
        }
        n132 = local write "Result files to read"(w219) -> ()
      }
      frame "Which file to read next" {
        n133 = local read "Result files to read"() -> (w255:path[])
        n134 = local read "File Index"() -> (w252:i32)
        n135 = Array Size(array=w255) -> (size(s)=w253:i32)
        n136 = Equal?(x=w253, y=w252) -> (x = y?=w251:bool)
        n137 = case shown="True" w251 {
          tunnel: w255 -> [w261 _]
          tunnel: [w262 "Load Selectors"] -> w254
          tunnel: w252 -> [w260 w274]
          tunnel: [w259 w274] -> w247
          frame False {
            n138 = Index Array(array=w261, index=w260) -> (element=w263:path)
            n139 = Search 1D Array(1D array="Results files choosen", element=w263) -> (index of element=w265:i32)  [unwired: 1 out]
            n140 = local write "Results file"(w263) -> ()
            n141 = call "Add_filename_suffix.vi"() -> ()  [unwired: 2 in, 4 out]
            n142 = case shown="-1" w265 {
              tunnel: "Results files choosen" -> [_ w273]
              tunnel: w263 -> [w269 w272]
              tunnel: ["Which file to read next" "Load Data"] -> w262
              frame 0, Default {
                n143 = Format Into String(format string="The filename\n \"%s\"\n has already been choosen" ("Format String"), w269) -> (resulting string=w267:string)  [unwired: 2 in, 1 out]
                n144 = One Button Dialog(message=w267) -> ()  [unwired: 2 out]
              }
              frame -1 {
                n145 = Build Array (concatenate)(w273, w272) -> (w271:path[])
                n146 = local write "Results files choosen"(w271) -> ()
              }
            }
            n147 = Increment(x=w260) -> (x+1=w259:i32)
          }
          frame True {
          }
        }
        n148 = Decrement(x=w247) -> (x-1=w246:i32)
        n149 = Build Array(w246) -> (w248:i32[])
        n150 = local read "stop"() -> (w250:bool)
        n151 = local write "File Index"(w247) -> ()
        n152 = property on="Result files to read" class="Arr (strict)"("Index Values"=w248) -> ()  [unwired: 2 in, 2 out]
        n153 = Not(x=w250) -> (.not. x?=w249:bool)
      }
      frame "Load Data" {
        n154 = stacked-sequence {
          seq-local: [w288 _] -> [_ w348]
          seq-local: [w287 _] -> [_ w353]
          seq-local: [w286 _] -> [_ w352]
          seq-local: [w284 _] -> [_ w351]
          tunnel: [TRUE _] -> w283
          tunnel: w282 -> [w302 w354]
          tunnel: w281 -> [w301 _]
          tunnel: [w300 _] -> w280
          tunnel: [w299 _] -> w279
          tunnel: [w298 _] -> w278
          tunnel: w277 -> [w297 _]
          tunnel: ["Which file to read next" _] -> w276
          frame #0 {
            w291 = TRUE  # Add Extra Channels?
            n155 = local read "Template"() -> (w295:path)
            n156 = call "Read_Data_file.vi"("Results file"="Results file", "Add Extra Channels?"=w291, "Template File"=w295, "Desired File Types"="File Tyoes to Read") -> ("Row numbers"=w286:i32[], "Template File Out"=w292:path, "Filetype"=w287:string, "Results file Out"=w288:path, "Ch names Out"=w293:string[], "Channel Values Out"=w289:string[][])  [unwired: 1 in, 9 out]
            n157 = local write "Template"(w292) -> ()
            n158 = Array Size(array=w293) -> (size(s)=w294:i32)
            n159 = Greater Than 0?(x=w294) -> (x > 0?=w284:bool)
            n160 = case shown="True" w284 {
              tunnel: w302 -> [w305 w318]
              tunnel: w301 -> [w306 w310]
              tunnel: w289 -> [_ w308]
              tunnel: [w305 w311] -> w300
              tunnel: [w306 w316] -> w299
              tunnel: [w304 w315] -> w298
              tunnel: w297 -> [w304 _]
              tunnel: w293 -> [_ w309]
              frame False {
              }
              frame True {
                n161 = for {
                  tunnel: w308 -> [w320] mode=indexing
                  tunnel: [w319] -> w307 mode=indexing
                  n162 = for {
                    tunnel: w320 -> [w322] mode=indexing
                    tunnel: [w321] -> w319 mode=indexing
                    n163 = call "Fast_string_Replace.vi"("Replace match with:"="[", "Input String"=w322, "regular expression"="(") -> ("Output String"=w323:string)  [unwired: 2 out]
                    n164 = call "Fast_string_Replace.vi"("Replace match with:"="]", "Input String"=w323, "regular expression"=")") -> ("Output String"=w321:string)  [unwired: 2 out]
                  }
                }
                n165 = call "Merge_channel_names.vi"("Preferred Channel array"=w310, "Channel array"=w309) -> ("Merged Channels"=w316:string[], "Preferred Channels Changed?"=w313:bool, "Channel Array Changed?"=w314:bool)
                n166 = for {
                  tunnel: w316 -> [w345] mode=indexing
                  tunnel: [w342] -> w315 mode=indexing
                  n167 = call "Fast_string_Replace.vi"("Replace match with:"=" ", "Input String"=w345, "regular expression"=":") -> ("Output String"=w341:string)  [unwired: 2 out]
                  n168 = call "Fast_string_Replace.vi"("Replace match with:"=" ", "Input String"=w341, "regular expression"="  ") -> ("Output String"=w340:string)  [unwired: 2 out]
                  n169 = call <vilib>:"Trim Whitespace.vi"("string"=w340) -> ("trimmed string"=w342:string)  [unwired: 1 in]
                }
                n170 = case shown="True" w313 {
                  tunnel: w318 -> [w333 w335]
                  tunnel: w310 -> [_ w337]
                  tunnel: [w333 w334] -> w312
                  tunnel: w316 -> [_ w336]
                  frame False {
                  }
                  frame True {
                    n171 = call "Merge_2D_values.vi"("Values In"=w335, "Present Channels"=w337, "Desired Channels"=w336) -> ("Values Out"=w334:string[][])
                  }
                }
                n172 = case shown="True" w314 {
                  tunnel: [w328 w332] -> w317
                  tunnel: w309 -> [_ w331]
                  tunnel: w307 -> [w328 w330]
                  tunnel: w316 -> [_ w329]
                  frame False {
                  }
                  frame True {
                    n173 = call "Merge_2D_values.vi"("Values In"=w330, "Present Channels"=w331, "Desired Channels"=w329) -> ("Values Out"=w332:string[][])
                  }
                }
                n174 = Build Array (concatenate)(w312, w317) -> (w311:string[][])
              }
            }
          }
          frame #1 {
            n175 = local read "Result files to read"() -> (w347:path[])
            n176 = local read "File Index"() -> (w350:i32)
            n177 = Decrement(x=w350) -> (x-1=w349:i32)
            n178 = case shown="True" w351 {
              tunnel: w354 -> [_ w367]
              tunnel: w353 -> [_ w365]
              tunnel: w352 -> [_ w363]
              tunnel: w349 -> [w355 w361]
              tunnel: w348 -> [_ w360]
              tunnel: w347 -> [w357 w362]
              tunnel: [w356 w359] -> w346
              frame False {
                n179 = Delete From Array(array=w357, length=1, index=w355) -> (array with subset deleted=w356:path[])  [unwired: 1 out]
                n180 = local write "File Index"(w355) -> ()
              }
              frame True {
                n181 = Array Size(array=w367) -> (size(s)=w369:i32[])
                n182 = Index Array(array=w369, index=0 ("Index")) -> (element=w366:i32)
                n183 = for {
                  tunnel: w361 -> [w386]
                  tunnel: [w385] -> w371 mode=indexing
                  tunnel: w366 -> [w382]
                  tunnel: w363 -> [w381] mode=indexing
                  i -> [w383]
                  n184 = Add(x=w383, y=w382) -> (x+y=w384:i32)
                  n185 = Build Array(w386, w381, w384) -> (w385:i32[])
                }
                n186 = case shown="0" w361 {
                  tunnel: w371 -> [w374 w379]
                  tunnel: [w374 w378] -> w370
                  tunnel: w365 -> [w373 w377]
                  tunnel: [w372 w375] -> w364
                  frame 0 {
                    n187 = Build Array(w373) -> (w372:string[])
                  }
                  frame 1, Default {
                    n188 = global read "Results_plotter_Global.vi" "Row Reference"() -> (w380:i32[][])
                    n189 = local read "Filetype"() -> (w376:string[])
                    n190 = Build Array (concatenate)(w376, w377) -> (w375:string[])
                    n191 = Build Array (concatenate)(w380, w379) -> (w378:i32[][])
                  }
                }
                "Filetype" <- w364
                n192 = Replace Array Subset(array=w362, new element=w360, index=w361) -> (w359:path[])
                n193 = global write "Results_plotter_Global.vi" "Row Reference"(w370) -> ()
              }
            }
            n194 = local write "Result files to read"(w346) -> ()
          }
        }
      }
      frame "Load Selectors" {
        n195 = while {
          shift-right: [w407] -> w392
          shift-left: _ -> [w409]
          tunnel: [w409] -> w391
          tunnel: w387 -> [w407]
          stop <- FALSE continue-if-true
        }
        n196 = Array Size(array=w399) -> (size(s)=w398:i32[])
        n197 = local read "Tolerances"() -> (w395:dbl[])
        n198 = Index Array(array=w398, index=0 ("Index")) -> (element=→"No Of Rows":i32)
        n199 = property on="X Ch Name" class="Ring (strict)"("Strings []"=w387) -> ()  [unwired: 2 in, 2 out]
        n200 = property on="Ordinate" class="Ring (strict)"("Strings []"=w387) -> ()  [unwired: 2 in, 2 out]
        n201 = property on="X Axis" class="Ring (strict)"("Strings []"=w387) -> ()  [unwired: 2 in, 2 out]
        n202 = property on="Y Ch Name" class="Ring (strict)"("Strings []"=w387) -> ()  [unwired: 2 in, 2 out]
        n203 = Equal?(x=w392, y=w391) -> (x = y?=w390:bool)
        n204 = Array Size(array=w387) -> (size(s)=w401:i32)
        n205 = Array Size(array=w395) -> (size(s)=w400:i32)
        n206 = property on="Multi Ordinate" class="LstBox (strict)"("Item Names"=w387) -> ()  [unwired: 2 in, 2 out]
        n207 = property on="Z Ch Name" class="Ring (strict)"("Strings []"=w387) -> ()  [unwired: 2 in, 2 out]
        n208 = Not Equal?(x=w401, y=w400) -> (x != y?=w402:bool)
        n209 = case shown="True" w402 {
          tunnel: w401 -> [_ w416]
          tunnel: w400 -> [_ w415]
          tunnel: w395 -> [_ w412]
          frame False {
          }
          frame True {
            n210 = Subtract(x=w416, y=w415) -> (x-y=w414:i32)
            n211 = Initialize Array(1.0 ("Element Data"), w414) -> (w411:dbl[])
            n212 = Build Array (concatenate)(w412, w411) -> (w410:dbl[])
            n213 = local write "Tolerances"(w410) -> ()
          }
        }
        n214 = Build Array (concatenate)("Don't Filter" ("Input Element"), w387) -> (w404:string[])
        n215 = global write "Results_plotter_Global.vi" "First Loop"(TRUE) -> ()
        n216 = property on="Filter on column 1:" class="Ring (strict)"("Strings []"=w404) -> ()  [unwired: 2 in, 2 out]
        n217 = Select(t="What is present?", s=w390, f="Set Axis Channels") -> (s? t:f=w394:string)
      }
      frame "Set Axis Channels" {
        n218 = Array Size(array=w423) -> (size(s)=w422:i32)
        n219 = Build Array("X" ("regular expression"), "Y" ("regular expression"), "Z" ("regular expression")) -> (w417:string[])
        n220 = Decrement(x=w422) -> (x-1=w421:i32)
        n221 = for {
          tunnel: w423 -> [w435]
          tunnel: w421 -> [w434]
          tunnel: w417 -> [w433] mode=indexing
          i -> [w429]
          n222 = while {
            tunnel: w435 -> [w449] mode=indexing
            tunnel: w434 -> [w448]
            tunnel: w433 -> [w446]
            tunnel: [w439] -> w432
            tunnel: [w444] -> w431
            i -> [w444]
            stop <- w447 continue-if-true
            n223 = call "Match_Pat_Case_In.vi"("String to match"=w446, "String"=w449) -> ("offset past match"=w443:i32)  [unwired: 1 in, 3 out]
            n224 = Less?(x=w444, y=w448) -> (x < y?=w445:bool)
            n225 = In Range and Coerce(upper limit=4, x=w443, lower limit=0) -> (In Range?=w440:bool)  [unwired: 1 out]
            n226 = Not(x=w440) -> (.not. x?=w439:bool)
            n227 = And(x=w439, y=w445) -> (x .and. y?=w447:bool)
          }
          n228 = Select(t=0, s=w432, f=w431) -> (s? t:f=w428:i32)
          n229 = case shown="1" w429 {
            tunnel: w428 -> [w436 w437 w438]
            frame 0, Default {
              n230 = local write "X Ch Name"(w436) -> ()
            }
            frame 1 {
              n231 = local write "Y Ch Name"(w437) -> ()
            }
            frame 2 {
              n232 = local write "Z Ch Name"(w438) -> ()
            }
          }
        }
      }
      frame "What is present?" {
        n233 = case shown="True" "Show Results Space Analysis" {
          tunnel: w453 -> [_ w457]
          tunnel: w452 -> [_ w456]
          frame False {
          }
          frame True {
            n234 = stacked-sequence {
              tunnel: w457 -> [w461]
              tunnel: w456 -> [w460]
              frame #0 {
                w458 = FALSE  # Summarise All
                n235 = call "Summarise.vi"("Channel Names"=w461, "Data"=w460, "Summarise All"=w458) -> ("Summary"=w459:string[][])  [unwired: 2 in]
                n236 = call "Results_Space_Analysis.vi"("Table"=w459) -> ()
              }
            }
          }
        }
      }
      frame "Ordinate Selector Type" {
        n237 = while {
          tunnel: [w480] -> w471
          shift-left: _ -> [w480]
          shift-right: ["Slice mode"] -> w472
          stop <- FALSE continue-if-true
          "Previous slice mode" <- w480
        }
        n238 = property on="Multi Ordinate" class="LstBox (strict)"("Visible"="Multi Ordinate?") -> ()  [unwired: 2 in, 2 out]
        n239 = global read "Results_plotter_Global.vi" "First Loop"() -> (w467:bool)
        n240 = Not(x="Multi Ordinate?") -> (.not. x?=w466:bool)
        n241 = local read "Intensity Plot?"() -> (w470:bool)
        n242 = property on="Ordinate Name" class="Str"("Visible"="Multi Ordinate?") -> ()  [unwired: 2 in, 2 out]
        n243 = property on="Ordinate" class="Ring (strict)"("Visible"=w466) -> ()  [unwired: 2 in, 2 out]
        n244 = Not Equal?(x=w472, y=w471) -> (x != y?=w463:bool)
        n245 = Or(x=w463, y="Update") -> (x .or. y?=w464:bool)
        n246 = case shown="False" "Multi Ordinate?" {
          frame False {
            n247 = Build Array("Ordinate") -> (w482:u16[])
            n248 = local write "Multi Ordinate"(w482) -> ()
          }
          frame True {
          }
        }
        n249 = Compound Arithmetic op=AND(invert w467, w464, w470) -> (w469:bool)
        "Slice mode Change?" <- w469
        n250 = property on="First Add label" class="Str"("Visible"=w466) -> ()  [unwired: 2 in, 2 out]
        n251 = property on="Additional Y Values" class="Arr (strict)"("Visible"=w466) -> ()  [unwired: 2 in, 2 out]
        n252 = property on="2nd Add label" class="Str"("Visible"=w466) -> ()  [unwired: 2 in, 2 out]
        n253 = Select(t="Change Slice mode", s=w469, f="Which rows are Non-Blank?") -> (s? t:f=w473:string)
        n254 = property on="Additional X Values" class="Arr (strict)"("Visible"=w466) -> ()  [unwired: 2 in, 2 out]
      }
      frame "Change Slice mode" {
        n255 = local read "Previous slice mode"() -> (w486:T4)
        n256 = local read "Slice mode"() -> (w500:T4)
        n257 = case shown="\"XY Slice (Plan)\"" w500 {
          tunnel: [w512 w517 w524 w529 w536 w542] -> w499
          tunnel: "Y Ch Name" -> [w510 w517 w524 w530 w535 w540]
          tunnel: "X Ch Name" -> [w512 w516 w523 w528 w536 w541]
          tunnel: [w511 w518 w523 w528 w535 w540] -> w490
          tunnel: "Z Ch Name" -> [w511 w518 w522 w529 w534 w542]
          tunnel: [w510 w516 w522 w530 w534 w541] -> w488
          tunnel: w486 -> [w509 w514 w520 w526 w533 w538]
          tunnel: [w507 w513 w519 w525 w532 w537] -> w485
          frame "XY Slice (Plan)" {
            n258 = Equal?(x=Plot_Slice."YX Slice (Plan)" ("Previous slice mode"), y=w509) -> (x = y?=w507:bool)
          }
          frame "YX Slice (Plan)" {
            n259 = Equal?(x=Plot_Slice."XY Slice (Plan)" ("Previous slice mode"), y=w514) -> (x = y?=w513:bool)
          }
          frame "YZ Slice (Cross)" {
            n260 = Equal?(x=Plot_Slice."ZY Slice (Cross)" ("Previous slice mode"), y=w520) -> (x = y?=w519:bool)
          }
          frame "ZY Slice (Cross)" {
            n261 = Equal?(x=Plot_Slice."YZ Slice (Cross)" ("Previous slice mode"), y=w526) -> (x = y?=w525:bool)
          }
          frame "XZ Slice (Side)" {
            n262 = Equal?(x=Plot_Slice."ZX Slice (Side)" ("Previous slice mode"), y=w533) -> (x = y?=w532:bool)
          }
          frame "ZX Slice (Side)" {
            n263 = Equal?(x=Plot_Slice."XZ Slice (Side)" ("Previous slice mode"), y=w538) -> (x = y?=w537:bool)
          }
        }
        n264 = case shown="True" w485 {
          frame False {
          }
          frame True {
            n265 = local read "Transpose"() -> (w506:bool)
            n266 = Not(x=w506) -> (.not. x?=w505:bool)
            n267 = local write "Transpose"(w505) -> ()
          }
        }
        n268 = local write "Update"(FALSE ("Update")) -> ()
        n269 = Increment(x=w490) -> (x+1=w493:u16)
        n270 = Increment(x=w488) -> (x+1=w492:u16)
        n271 = local read "Filter Array"() -> (w497:u16[])
        n272 = Array Subset(array=w497, index=2 ("Array Index")) -> (w495:u16[])  [unwired: 1 in]
        n273 = Build Array (concatenate)(w493, w492, w495) -> (w494:u16[])
        n274 = local write "Filter Array"(w494) -> ()
        n275 = local write "Absisca"(w499) -> ()
      }
      frame "Which rows are Non-Blank?" {
        n276 = while {
          tunnel: [w559] -> w553
          tunnel: [w560] -> w554
          shift-left: _ -> [w561]
          shift-right: [w562] -> w546
          shift-left: _ -> [w564]
          shift-right: [w563] -> _
          stop <- FALSE continue-if-true
          n277 = local read "Multi Ordinate"() -> (w562:i32[])
          n278 = local read "Absisca"() -> (w563:u16)
          n279 = Equal?(x=w563, y=w564) -> (x = y?=w560:bool)
          n280 = Equal?(x=w562, y=w561) -> (x = y?=w559:bool)
        }
        n281 = global read "Results_plotter_Global.vi" "First Loop"() -> (w548:bool)
        n282 = Compound Arithmetic op=AND(invert w548, w554, w553) -> (w552:bool)
        n283 = Array Size(array=w546) -> (size(s)=w545:i32)
        n284 = Greater?(x=w545, y=1) -> (0:w543:bool)
        n285 = global write "Results_plotter_Global.vi" "Multi Ordinate?"(w543) -> ()
        n286 = Select(t="Create Selectors", s=w552, f="Evaluate Blank Rows") -> (s? t:f=w549:string)
      }
      frame "Evaluate Blank Rows" {
        n287 = local read "Multi Ordinate"() -> (w566:i32[])
        n288 = local read "Absisca"() -> (w567:u16)
        n289 = for {
          tunnel: w568 -> [w574] mode=indexing
          tunnel: w567 -> [w577]
          tunnel: w566 -> [w576]
          tunnel: [w573] -> w565 mode=indexing
          n290 = Index Array(array=w574, index=w577) -> (element=w578:string)
          n291 = call "Convert_to_number.vi"("string"=w578) -> ("Number"=w579:dbl)  [unwired: 1 out]
          n292 = Not A Number/Path/Refnum?(number/path/refnum=w579) -> (NaN/Path/Refnum?=w575:bool)
          n293 = case shown="False" w575 {
            tunnel: w576 -> [w583 _]
            tunnel: w574 -> [w582 _]
            tunnel: [w580 FALSE] -> w573
            frame False {
              n294 = for {
                tunnel: w583 -> [w589] mode=indexing
                tunnel: w582 -> [w587]
                tunnel: [w584] -> w581 mode=indexing
                n295 = Index Array(array=w587, index=w589) -> (element=w588:string)
                n296 = call "Convert_to_number.vi"("string"=w588) -> ("Number"=w586:dbl)  [unwired: 1 out]
                n297 = Not A Number/Path/Refnum?(number/path/refnum=w586) -> (NaN/Path/Refnum?=w585:bool)
                n298 = Not(x=w585) -> (.not. x?=w584:bool)
              }
              n299 = Or Array Elements(Boolean array=w581) -> (logical OR=w580:bool)
            }
            frame True {
            }
          }
        }
        "Non-Blank Rows" <- w565
      }
      frame "Create Selectors" {
        n300 = local read "Non-Blank Rows"() -> (w594:bool[])
        n301 = local read "Tolerances"() -> (w592:dbl[])
        n302 = global read "Results_plotter_Global.vi" "Precision"() -> (w591:string[])
        n303 = Array Size(array=w602) -> (size(s)=w601:i32[])
        n304 = Index Array(array=w601, index=0 ("Index")) -> (element=w604:i32)
        n305 = for {
          tunnel: w602 -> [w620]
          tunnel: "Filter Array" -> [w612] mode=indexing
          shift-right: [w619] -> w593
          shift-left: _ -> [w617]
          tunnel: w604 -> [w618]
          tunnel: [w615] -> w599 mode=indexing
          tunnel: w594 -> [w614]
          tunnel: w592 -> [w613]
          tunnel: w591 -> [w610]
          i -> [w616]
          n306 = Decrement(x=w612) -> (x-1=w609:u16)
          n307 = Index Array(array=w610, index=w609) -> (element=w608:string)
          n308 = Index Array(array=w613, index=w609) -> (element=w611:dbl)
          n309 = case shown="5" w616 {
            tunnel: w620 -> [w633 w669 w710 w751 w792 w835 w876]
            tunnel: w612 -> [w632 w668 w709 w750 w791 w834 w875]
            tunnel: w611 -> [w631 w667 w708 w749 w790 w833 w874]
            tunnel: [w630 w666 w707 w748 w789 w832 w873] -> w619
            tunnel: w618 -> [w628 w665 w706 w747 w788 w831 w872]
            tunnel: w617 -> [_ w664 w705 w746 w787 w830 w871]
            tunnel: w616 -> [w627 w663 w702 w743 w784 w829 w868]
            tunnel: [w623 w658 w701 w742 w783 w824 w867] -> w615
            tunnel: w614 -> [w622 w657 w700 w741 w782 w823 w866]
            tunnel: w608 -> [w621 w656 w699 w740 w781 w822 w865]
            frame 0, Default {
              n310 = case shown="1, Default" w632 {
                tunnel: w633 -> [w639 w649]
                tunnel: w632 -> [w640 w648]
                tunnel: w631 -> [_ w655]
                tunnel: [w635 w652] -> w630
                tunnel: "Filter Bins 1" -> [_ w653]
                tunnel: [string[] [] ("Write Attribute") w654] -> w629
                tunnel: w628 -> [w637 _]
                tunnel: w627 -> [w643 w651]
                tunnel: [i32[] [0] ("Filter Bins Out") w650] -> w625
                tunnel: [TRUE ("Unchanged?") w647] -> w623
                tunnel: w622 -> [_ w646]
                tunnel: w621 -> [_ w645]
                frame 0 {
                  n311 = call "Create_filter_points.vi"("Channel to Filter On"=w640, "Index"=w643, "Ch Values In"=w639) -> ()  [unwired: 4 in, 4 out]
                  n312 = Initialize Array(TRUE, w637) -> (w636:bool[])
                  n313 = Build Array(w636) -> (w635:bool[][])
                }
                frame 1, Default {
                  n314 = call "Create_filter_points.vi"("Non-Blank Rows"=w646, "Precision"=w645, "Channel to Filter On"=w648, "Tolerance"=w655, "Index"=w651, "Filter Bins 1"=w653, "Ch Values In"=w649) -> ("Unchanged?"=w647:bool, "Accept array"=w652:bool[][], "Filter Bins Out"=w650:i32[], "Bin Names"=w654:string[])
                }
              }
              n315 = Equal?(x="Filter Bins 1", y=w625) -> (x = y?=w624:bool)
              n316 = case shown="False" w624 {
                tunnel: w625 -> [w634 _]
                frame False {
                  n317 = local write "Filter Bins 1"(w634) -> ()
                }
                frame True {
                }
              }
              n318 = property on="Filter bins 1" class="LstBox (strict)"("Item Names"=w629) -> ()  [unwired: 2 in, 2 out]
            }
            frame 1 {
              n319 = case shown="1, Default" w668 {
                tunnel: w669 -> [_ w681]
                tunnel: w668 -> [w672 w680]
                tunnel: w667 -> [_ w688]
                tunnel: [w676 w684] -> w666
                tunnel: "Filter Bins 2" -> [_ w686]
                tunnel: [string[] [] ("Write Attribute") w690] -> w662
                tunnel: w665 -> [_ _]
                tunnel: w664 -> [w676 w689]
                tunnel: w663 -> [w675 w687]
                tunnel: [i32[] [0] ("Filter Bins Out") w682] -> w661
                tunnel: [TRUE ("Unchanged?") w679] -> w658
                tunnel: w657 -> [_ w678]
                tunnel: w656 -> [_ w677]
                frame 0 {
                  n320 = call "Create_filter_points.vi"("Channel to Filter On"=w672, "Index"=w675) -> ()  [unwired: 5 in, 4 out]
                }
                frame 1, Default {
                  n321 = call "Create_filter_points.vi"("Non-Blank Rows"=w678, "Precision"=w677, "Channel to Filter On"=w680, "Tolerance"=w688, "Index"=w687, "Filter Bins 1"=w686, "Ch Values In"=w681) -> ("Unchanged?"=w679:bool, "Accept array"=w685:bool[][], "Filter Bins Out"=w682:i32[], "Bin Names"=w690:string[])
                  n322 = for {
                    tunnel: w689 -> [w695]
                    tunnel: w685 -> [w694] mode=indexing
                    shift-right: [w691] -> w684
                    shift-left: bool[][] [] -> [w693]
                    n323 = for {
                      tunnel: w694 -> [w698]
                      tunnel: w695 -> [w697] mode=indexing
                      tunnel: [w696] -> _ mode=indexing
                      tunnel: [w696] -> w692 mode=indexing
                      n324 = And(x=w698, y=w697) -> (x .and. y?=w696:bool[])
                    }
                    n325 = Build Array (concatenate)(w693, w692) -> (w691:bool[][])
                  }
                }
              }
              n326 = Equal?(x="Filter Bins 2", y=w661) -> (x = y?=w659:bool)
              n327 = case shown="False" w659 {
                tunnel: w661 -> [w670 _]
                frame False {
                  n328 = local write "Filter Bins 2"(w670) -> ()
                }
                frame True {
                }
              }
              n329 = property on="Filter Bins 2" class="LstBox (strict)"("Item Names"=w662) -> ()  [unwired: 2 in, 2 out]
            }
            frame 2 {
              n330 = case shown="0" w709 {
                tunnel: w710 -> [_ w720]
                tunnel: w709 -> [w713 w721]
                tunnel: w708 -> [_ w732]
                tunnel: [w716 w733] -> w707
                tunnel: "Filter 3" -> [_ w724]
                tunnel: [string[] [] ("Write Attribute") w735] -> w703
                tunnel: w706 -> [_ _]
                tunnel: w705 -> [w716 w734]
                tunnel: w702 -> [w715 w727]
                tunnel: [TRUE ("Unchanged?") w719] -> w701
                tunnel: w700 -> [_ w718]
                tunnel: w699 -> [_ w717]
                frame 0 {
                  n331 = call "Create_filter_points.vi"("Channel to Filter On"=w713, "Index"=w715) -> ()  [unwired: 5 in, 4 out]
                  n332 = local write "Filter 3"(0) -> ()
                }
                frame 1, Default {
                  n333 = Build Array(w724) -> (w731:u16[])
                  n334 = call "Create_filter_points.vi"("Non-Blank Rows"=w718, "Precision"=w717, "Channel to Filter On"=w721, "Tolerance"=w732, "Index"=w727, "Filter Bins 1"=w731, "Ch Values In"=w720) -> ("Unchanged?"=w719:bool, "Accept array"=w729:bool[][], "Filter Bins Out"=w725:i32[], "Bin Names"=w735:string[])
                  n335 = Index Array(array=w725, index=0 ("Index")) -> (element=w722:i32)
                  n336 = Index Array(array=w729, index (row)=0 ("Index")) -> (element=w728:bool[])  [unwired: 1 in]
                  n337 = Equal?(x=w724, y=w722) -> (x = y?=w723:bool)
                  n338 = case shown="True" w723 {
                    tunnel: w722 -> [w736 _]
                    frame False {
                      n339 = local write "Filter 3"(w736) -> ()
                    }
                    frame True {
                    }
                  }
                  n340 = for {
                    tunnel: w728 -> [w739]
                    tunnel: w734 -> [w738] mode=indexing
                    tunnel: [w737] -> w733 mode=indexing
                    n341 = And(x=w739, y=w738) -> (x .and. y?=w737:bool[])
                  }
                }
              }
              n342 = property on="Filter 3" class="Ring (strict)"("Strings []"=w703) -> ()  [unwired: 2 in, 2 out]
            }
            frame 3 {
              n343 = case shown="1, Default" w750 {
                tunnel: w751 -> [_ w762]
                tunnel: w750 -> [w754 w761]
                tunnel: w749 -> [_ w773]
                tunnel: [w757 w774] -> w748
                tunnel: "Filter 4" -> [_ w765]
                tunnel: [string[] [] ("Write Attribute") w776] -> w744
                tunnel: w747 -> [_ _]
                tunnel: w746 -> [w757 w775]
                tunnel: w743 -> [w756 w768]
                tunnel: [TRUE ("Unchanged?") w760] -> w742
                tunnel: w741 -> [_ w759]
                tunnel: w740 -> [_ w758]
                frame 0 {
                  n344 = call "Create_filter_points.vi"("Channel to Filter On"=w754, "Index"=w756) -> ()  [unwired: 5 in, 4 out]
                  n345 = local write "Filter 4"(0) -> ()
                }
                frame 1, Default {
                  n346 = Build Array(w765) -> (w772:u16[])
                  n347 = call "Create_filter_points.vi"("Non-Blank Rows"=w759, "Precision"=w758, "Channel to Filter On"=w761, "Tolerance"=w773, "Index"=w768, "Filter Bins 1"=w772, "Ch Values In"=w762) -> ("Unchanged?"=w760:bool, "Accept array"=w770:bool[][], "Filter Bins Out"=w766:i32[], "Bin Names"=w776:string[])
                  n348 = Index Array(array=w766, index=0 ("Index")) -> (element=w764:i32)
                  n349 = Equal?(x=w765, y=w764) -> (x = y?=w763:bool)
                  n350 = Index Array(array=w770, index (row)=0 ("Index")) -> (element=w769:bool[])  [unwired: 1 in]
                  n351 = case shown="False" w763 {
                    tunnel: w764 -> [w777 _]
                    frame False {
                      n352 = local write "Filter 4"(w777) -> ()
                    }
                    frame True {
                    }
                  }
                  n353 = for {
                    tunnel: w769 -> [w780]
                    tunnel: w775 -> [w779] mode=indexing
                    tunnel: [w778] -> w774 mode=indexing
                    n354 = And(x=w780, y=w779) -> (x .and. y?=w778:bool[])
                  }
                }
              }
              n355 = property on="Filter 4" class="Ring (strict)"("Strings []"=w744) -> ()  [unwired: 2 in, 2 out]
            }
            frame 4 {
              n356 = case shown="1, Default" w791 {
                tunnel: w792 -> [_ w803]
                tunnel: w791 -> [w795 w802]
                tunnel: w790 -> [_ w814]
                tunnel: [w798 w815] -> w789
                tunnel: "Filter 5" -> [_ w805]
                tunnel: [string[] [] ("Write Attribute") w817] -> w785
                tunnel: w788 -> [_ _]
                tunnel: w787 -> [w798 w816]
                tunnel: w784 -> [w797 w809]
                tunnel: [TRUE ("Unchanged?") w801] -> w783
                tunnel: w782 -> [_ w800]
                tunnel: w781 -> [_ w799]
                frame 0 {
                  n357 = call "Create_filter_points.vi"("Channel to Filter On"=w795, "Index"=w797) -> ()  [unwired: 5 in, 4 out]
                  n358 = local write "Filter 5"(0) -> ()
                }
                frame 1, Default {
                  n359 = Build Array(w805) -> (w813:u16[])
                  n360 = call "Create_filter_points.vi"("Non-Blank Rows"=w800, "Precision"=w799, "Channel to Filter On"=w802, "Tolerance"=w814, "Index"=w809, "Filter Bins 1"=w813, "Ch Values In"=w803) -> ("Unchanged?"=w801:bool, "Accept array"=w811:bool[][], "Filter Bins Out"=w807:i32[], "Bin Names"=w817:string[])
                  n361 = Index Array(array=w807, index=0 ("Index")) -> (element=w806:i32)
                  n362 = Equal?(x=w805, y=w806) -> (x = y?=w804:bool)
                  n363 = Index Array(array=w811, index (row)=0 ("Index")) -> (element=w810:bool[])  [unwired: 1 in]
                  n364 = case shown="False" w804 {
                    tunnel: w806 -> [w818 _]
                    frame False {
                      n365 = local write "Filter 5"(w818) -> ()
                    }
                    frame True {
                    }
                  }
                  n366 = for {
                    tunnel: w810 -> [w821]
                    tunnel: w816 -> [w820] mode=indexing
                    tunnel: [w819] -> w815 mode=indexing
                    n367 = And(x=w821, y=w820) -> (x .and. y?=w819:bool[])
                  }
                }
              }
              n368 = property on="Filter 5" class="Ring (strict)"("Strings []"=w785) -> ()  [unwired: 2 in, 2 out]
            }
            frame 5 {
              n369 = case shown="1, Default" w834 {
                tunnel: w835 -> [_ w852]
                tunnel: w834 -> [w838 w851]
                tunnel: w833 -> [_ w856]
                tunnel: [w842 w843] -> w832
                tunnel: "Single Series" -> [_ w854]
                tunnel: [string[] [] ("Write Attribute") w858] -> w828
                tunnel: w831 -> [_ _]
                tunnel: w830 -> [w842 w857]
                tunnel: w829 -> [w841 w855]
                tunnel: [i32[] [0] ("Filter Bins Out") w853] -> w827
                tunnel: [TRUE ("Unchanged?") w850] -> w824
                tunnel: w823 -> [_ w849]
                tunnel: w822 -> [_ w848]
                frame 0 {
                  n370 = call "Create_filter_points.vi"("Channel to Filter On"=w838, "Index"=w841) -> ()  [unwired: 5 in, 4 out]
                }
                frame 1, Default {
                  n371 = call "Create_filter_points.vi"("Non-Blank Rows"=w849, "Precision"=w848, "Channel to Filter On"=w851, "Tolerance"=w856, "Index"=w855, "Filter Bins 1"=w854, "Ch Values In"=w852) -> ("Unchanged?"=w850:bool, "Accept array"=w845:bool[][], "Filter Bins Out"=w853:i32[], "Bin Names"=w858:string[])
                  n372 = Index Array(array=w845, index (row)=0 ("Index")) -> (element=w846:bool[])  [unwired: 1 in]
                  n373 = for {
                    shift-right: [w859] -> w844
                    shift-left: w846 -> [w861]
                    tunnel: w845 -> [w860] mode=indexing
                    n374 = Or(x=w860, y=w861) -> (x .or. y?=w859:bool[])
                  }
                  n375 = for {
                    tunnel: w844 -> [w864]
                    tunnel: w857 -> [w863] mode=indexing
                    tunnel: [w862] -> w843 mode=indexing
                    n376 = And(x=w864, y=w863) -> (x .and. y?=w862:bool[])
                  }
                }
              }
              n377 = Equal?(x="Single Series", y=w827) -> (x = y?=w825:bool)
              n378 = case shown="False" w825 {
                tunnel: w827 -> [w836 _]
                frame False {
                  n379 = local write "Single Series"(w836) -> ()
                }
                frame True {
                }
              }
              n380 = property on="Single Series" class="LstBox (strict)"("Item Names"=w828) -> ()  [unwired: 2 in, 2 out]
            }
            frame 6 {
              n381 = case shown="1, Default" w875 {
                tunnel: w876 -> [_ w887]
                tunnel: w875 -> [w879 w886]
                tunnel: w874 -> [_ w894]
                tunnel: [w882 w899] -> w873
                tunnel: "Filter 6" -> [_ w889]
                tunnel: [string[] [] ("Write Attribute") w901] -> w869
                tunnel: w872 -> [_ _]
                tunnel: w871 -> [w882 w900]
                tunnel: w868 -> [w881 w893]
                tunnel: [TRUE ("Unchanged?") w885] -> w867
                tunnel: w866 -> [_ w884]
                tunnel: w865 -> [_ w883]
                frame 0 {
                  n382 = call "Create_filter_points.vi"("Channel to Filter On"=w879, "Index"=w881) -> ()  [unwired: 5 in, 4 out]
                  n383 = local write "Filter 6"(0) -> ()
                }
                frame 1, Default {
                  n384 = Build Array(w889) -> (w895:u16[])
                  n385 = call "Create_filter_points.vi"("Non-Blank Rows"=w884, "Precision"=w883, "Channel to Filter On"=w886, "Tolerance"=w894, "Index"=w893, "Filter Bins 1"=w895, "Ch Values In"=w887) -> ("Unchanged?"=w885:bool, "Accept array"=w897:bool[][], "Filter Bins Out"=w891:i32[], "Bin Names"=w901:string[])
                  n386 = Index Array(array=w891, index=0 ("Index")) -> (element=w890:i32)
                  n387 = Equal?(x=w889, y=w890) -> (x = y?=w888:bool)
                  n388 = Index Array(array=w897, index (row)=0 ("Index")) -> (element=w896:bool[])  [unwired: 1 in]
                  n389 = case shown="False" w888 {
                    tunnel: w890 -> [w902 _]
                    frame False {
                      n390 = local write "Filter 6"(w902) -> ()
                    }
                    frame True {
                    }
                  }
                  n391 = for {
                    tunnel: w896 -> [w905]
                    tunnel: w900 -> [w904] mode=indexing
                    tunnel: [w903] -> w899 mode=indexing
                    n392 = And(x=w905, y=w904) -> (x .and. y?=w903:bool[])
                  }
                }
              }
              n393 = property on="Filter 6" class="Ring (strict)"("Strings []"=w869) -> ()  [unwired: 2 in, 2 out]
            }
          }
        }
        "Accept Array" <- w593
        n394 = And Array Elements(Boolean array=w599) -> (logical AND=w598:bool)
        n395 = Select(t="Select all for Filter 2", s=w598, f="Create Selectors") -> (s? t:f=w596:string)
      }
      frame "Select all for Filter 2" {
        n396 = local read "Slice mode Change?"() -> (w907:bool)
        n397 = case shown="True" w907 {
          frame False {
          }
          frame True {
            n398 = property on="Filter Bins 2" class="LstBox (strict)"() -> ("Item Names"=w921:string[])  [unwired: 2 in, 2 out]
            n399 = Array Size(array=w921) -> (size(s)=w920:i32)
            n400 = Build Array("Blanks", "Numeric", "Non Numeric", "Non Blanks", "Show All" ("Input Element")) -> (w914:string[])
            n401 = local read "Filter Bins 1"() -> (w923:i32[])
            n402 = while {
              tunnel: w921 -> [w936] mode=indexing
              tunnel: w920 -> [w939]
              shift-right: [w930] -> w912
              shift-left: i32[] [] -> [w931]
              tunnel: w914 -> [w933]
              i -> [w932]
              stop <- w937 stop-if-true
              n403 = String Subset(string=w936, length (rest)=4 ("length (rest)")) -> (substring=w941:string)  [unwired: 1 out]
              n404 = Match Pattern(string=w936, regular expression=" (") -> (before substring=w934:string)  [unwired: 4 out]
              n405 = Search 1D Array(1D array=w933, element=w934) -> (index of element=w929:i32)  [unwired: 1 out]
              n406 = Equal?(x="NOT ", y=w941) -> (x = y?=w928:bool)
              n407 = Equal?(x=w939, y=w932) -> (x = y?=w938:bool)
              n408 = Less Than 0?(x=w929) -> (x < 0?=w927:bool)
              n409 = Or(x=w928, y=w938) -> (x .or. y?=w937:bool)
              n410 = Compound Arithmetic op=AND(w927, invert w928) -> (w926:bool)
              n411 = case shown="False" w926 {
                tunnel: w932 -> [_ w946]
                tunnel: w931 -> [w943 w945]
                tunnel: [w943 w944] -> w930
                frame False {
                }
                frame True {
                  n412 = Build Array (concatenate)(w945, w946) -> (w944:i32[])
                }
              }
            }
            n413 = Array Size(array=w923) -> (size(s)=w925:i32)
            n414 = case shown="1" w925 {
              tunnel: [w947 w950] -> w924
              tunnel: w923 -> [_ w949]
              tunnel: i32[] [1] ("Filter Bins 1") -> [w947 w948]
              frame 0, Default {
              }
              frame 1 {
                n415 = Index Array(array=w949, index=0 ("Index")) -> (element=w952:i32)
                n416 = Greater Than 0?(x=w952) -> (x > 0?=w951:bool)
                n417 = Select(t=w949, s=w951, f=w948) -> (s? t:f=w950:i32[])
              }
            }
            n418 = local write "Filter Bins 1"(w924) -> ()
            n419 = local write "Filter Bins 2"(w912) -> ()
          }
        }
      }
      frame "Re Plot Data?" {
        n420 = while {
          tunnel: [w1000] -> w962
          shift-left: _ -> [w1002]
          shift-right: [w1001] -> _
          tunnel: [w1005] -> w968
          shift-left: _ -> [w1003]
          shift-right: [w1004] -> _
          tunnel: [w1009] -> w970
          shift-left: _ -> [w1008]
          shift-right: [w1007] -> w954
          tunnel: [w1010] -> w971
          shift-left: _ -> [w1012]
          shift-right: [w1011] -> _
          tunnel: [w1014] -> w972
          shift-left: _ -> [w1013]
          shift-right: [w1006] -> _
          tunnel: [w1015] -> w975
          tunnel: [w1016] -> w976
          shift-left: _ -> [w1017]
          shift-right: [w1018] -> _
          shift-left: _ -> [w1020]
          shift-right: [w1019] -> _
          tunnel: [w1021] -> w955
          shift-left: _ -> [w1022]
          shift-right: [w1023] -> _
          tunnel: [w998] -> w965
          shift-right: [w995] -> _
          shift-left: _ -> [w994]
          tunnel: [w997] -> w964
          shift-right: [w993] -> _
          shift-left: _ -> [w996]
          tunnel: [w990] -> w963
          shift-right: [w991] -> _
          shift-left: _ -> [w992]
          shift-right: [w988] -> _
          shift-left: _ -> [w989]
          tunnel: [w987] -> w957
          stop <- FALSE continue-if-true
          n421 = local read "Ordinate Name"() -> (w988:string)
          n422 = local read "Additional X Values"() -> (w995:dbl[])
          n423 = local read "Additional Y Values"() -> (w993:dbl[])
          n424 = local read "Intensity Plot?"() -> (w1007:bool)
          n425 = local read "color and symbol"() -> (w991:bool)
          n426 = local read "Accept Array"() -> (w1023:bool[][])
          n427 = local read "No of Contours"() -> (w1004:i32)
          n428 = local read "Point Size"() -> (w1001:i32)
          n429 = local read "Multi Ordinate"() -> (w1018:i32[])
          n430 = local read "Transpose"() -> (w1006:bool)
          n431 = local read "Resolution"() -> (w1011:dbl)
          n432 = local read "Absisca"() -> (w1019:u16)
          n433 = Equal?(x=w988, y=w989) -> (x = y?=w987:bool)
          n434 = Equal?(x=w1006, y=w1013) -> (x = y?=w1014:bool)
          n435 = Equal?(x=w991, y=w992) -> (x = y?=w990:bool)
          n436 = Equal?(x=w1004, y=w1003) -> (x = y?=w1005:bool)
          n437 = Equal?(x=w1001, y=w1002) -> (x = y?=w1000:bool)
          n438 = Equal?(x=w1011, y=w1012) -> (x = y?=w1010:bool)
          n439 = Equal?(x=w995, y=w994) -> (x = y?=w998:bool)
          n440 = Equal?(x=w993, y=w996) -> (x = y?=w997:bool)
          n441 = Equal?(x=w1019, y=w1020) -> (x = y?=w1016:bool)
          n442 = Equal?(x=w1023, y=w1022) -> (x = y?=w1021:bool)
          n443 = Equal?(x=w1007, y=w1008) -> (x = y?=w1009:bool)
          n444 = Equal?(x=w1018, y=w1017) -> (x = y?=w1015:bool)
        }
        n445 = global read "Results_plotter_Global.vi" "First Loop"() -> (w966:bool)
        n446 = while {
          shift-right: [w986] -> _
          shift-left: _ -> [w985]
          shift-right: [w983] -> _
          shift-left: _ -> [w984]
          tunnel: [w982] -> w961
          tunnel: [w981] -> w960
          stop <- FALSE continue-if-true
          n447 = local read "Filter Bins 1"() -> (w983:i32[])
          n448 = local read "Filter Bins 2"() -> (w986:i32[])
          n449 = Equal?(x=w983, y=w984) -> (x = y?=w981:bool)
          n450 = Equal?(x=w986, y=w985) -> (x = y?=w982:bool)
        }
        n451 = Not(x=w954) -> (.not. x?=w958:bool)
        n452 = property on="XY Plot" class="XYGraph (strict)"("Visible"=w958) -> ()  [unwired: 2 in, 2 out]
        n453 = property on="Intensity Graph" class="IntGraph (strict)"("Visible"=w954) -> ()  [unwired: 2 in, 2 out]
        n454 = property on="Resolution" class="DigNum (strict)"("Visible"=w954) -> ()  [unwired: 2 in, 2 out]
        n455 = property on="Bkgnd Value" class="DigNum (strict)"("Visible"=w954) -> ()  [unwired: 2 in, 2 out]
        n456 = Compound Arithmetic op=AND(w961, w960) -> (w959:bool)
        n457 = Compound Arithmetic op=AND(w957, w959, w962, w963, w968, w971, w972, w976, w975, w955, w970, w965, w964, invert w966) -> (w974:bool)
        n458 = Select(t="What to do next?", s=w974, f="Prepare for Plotting") -> (s? t:f=w973:string)
      }
      frame "Prepare for Plotting" {
        n459 = local read "Filter Array"() -> (w1032:u16[])
        n460 = local read "Multi Ordinate"() -> (w1026:i32[])
        n461 = Index Array(array=w1032, index=0 ("Index")) -> (element=w1029:u16)
        n462 = Equal To 0?(x=w1029) -> (x = 0?=w1030:bool)
        n463 = for {
          tunnel: w1026 -> [w1038] mode=indexing
          tunnel: [w1037] -> w1024 mode=indexing
          tunnel: w1025 -> [w1036]
          n464 = Index Array(array=w1036, index=w1038) -> (element=w1037:string)
        }
        "Ordinate Strings" <- w1024
        n465 = case shown="False" w1030 {
          tunnel: w1029 -> [w1044 _]
          tunnel: w1025 -> [w1042 _]
          tunnel: [w1039 string[] []] -> w1028
          frame False {
            n466 = Decrement(x=w1044) -> (x-1=w1043:u16)
            n467 = local read "Filter Bins 1"() -> (w1046:i32[])
            n468 = property on="Filter bins 1" class="LstBox (strict)"() -> ("Item Names"=w1045:string[])  [unwired: 2 in, 2 out]
            n469 = Index Array(array=w1042, index=w1043) -> (element=w1040:string)
            n470 = for {
              tunnel: w1046 -> [w1049] mode=indexing
              tunnel: w1045 -> [w1048]
              tunnel: [w1047] -> w1041 mode=indexing
              n471 = Index Array(array=w1048, index=w1049) -> (element=w1047:string)
            }
            n472 = Build Array (concatenate)(w1040, w1041) -> (w1039:string[])
          }
          frame True {
          }
        }
        "Filter 1 Strings" <- w1028
      }
      frame "Prepare Filter2 strings" {
        n473 = local read "Filter Array"() -> (w1057:u16[])
        n474 = Index Array(array=w1057, index=1 ("Index")) -> (element=w1054:u16)
        n475 = Equal To 0?(x=w1054) -> (x = 0?=w1055:bool)
        n476 = case shown="False" w1055 {
          tunnel: w1054 -> [w1066 _]
          tunnel: w1053 -> [w1064 _]
          tunnel: [w1061 string[] []] -> w1051
          frame False {
            n477 = Decrement(x=w1066) -> (x-1=w1065:u16)
            n478 = local read "Filter Bins 2"() -> (w1068:i32[])
            n479 = property on="Filter Bins 2" class="LstBox (strict)"() -> ("Item Names"=w1067:string[])  [unwired: 2 in, 2 out]
            n480 = Index Array(array=w1064, index=w1065) -> (element=w1062:string)
            n481 = for {
              tunnel: w1068 -> [w1071] mode=indexing
              tunnel: w1067 -> [w1070]
              tunnel: [w1069] -> w1063 mode=indexing
              n482 = Index Array(array=w1070, index=w1071) -> (element=w1069:string)
            }
            n483 = Build Array (concatenate)(w1062, w1063) -> (w1061:string[])
          }
          frame True {
          }
        }
        "Filter 2 Strings" <- w1051
      }
      frame "Plot Data" {
        n484 = stacked-sequence {
          seq-local: [w1079 _ _] -> [_ w1112 _]
          seq-local: [w1078 _ _] -> [_ w1111 _]
          tunnel: w1076 -> [_ w1121 _]
          tunnel: [_ TRUE _] -> w1075
          tunnel: [_ _ w1141] -> w1074
          tunnel: w1073 -> [w1080 _ _]
          frame #0 {
            n485 = local read "Ordinate Strings"() -> (w1079:string[])
            n486 = for {
              tunnel: w1079 -> [w1082] mode=indexing
              tunnel: w1080 -> [w1085]
              tunnel: [w1083] -> w1078 mode=indexing
              n487 = String Length(string=w1082) -> (length=w1081:i32)
              n488 = for {
                tunnel: w1082 -> [w1089]
                tunnel: w1085 -> [w1086] mode=indexing
                shift-right: [w1093] -> w1083
                shift-left: -1 -> [w1091]
                tunnel: w1081 -> [w1087]
                i -> [w1092]
                n489 = String Subset(string=w1086, length (rest)=w1087) -> (substring=w1088:string)  [unwired: 1 out]
                n490 = Equal?(x=w1088, y=w1089) -> (x = y?=w1090:bool)
                n491 = case shown="True" w1090 {
                  tunnel: [w1105 w1108] -> w1093
                  tunnel: w1092 -> [w1104 _]
                  tunnel: w1091 -> [w1103 w1108]
                  tunnel: w1087 -> [w1102 _]
                  tunnel: w1086 -> [w1101 _]
                  frame True {
                    n492 = String Subset(string=w1101, offset (0)=w1102) -> (substring=w1095:string)  [unwired: 1 out]
                    n493 = call <vilib>:"Trim Whitespace.vi"("string"=w1095) -> ("trimmed string"=w1094:string)  [unwired: 1 in]
                    n494 = Equal?(x=w1094, y="Err") -> (x = y?=w1097:bool)
                    n495 = Equal?(x=w1094, y="err") -> (x = y?=w1098:bool)
                    n496 = Or(x=w1097, y=w1098) -> (x .or. y?=w1096:bool)
                    n497 = case shown="True" w1096 {
                      tunnel: [w1106 w1107] -> w1105
                      tunnel: w1104 -> [w1106 _]
                      tunnel: w1103 -> [_ w1107]
                      frame True {
                      }
                      frame False {
                      }
                    }
                  }
                  frame False {
                  }
                }
              }
            }
          }
          frame #1 {
            n498 = local read "Accept Array"() -> (w1123:bool[][])
            n499 = local read "Filter 1 Strings"() -> (w1125:string[])
            n500 = local read "Filter 2 Strings"() -> (w1124:string[])
            n501 = local read "Multi Ordinate?"() -> (w1117:bool)
            n502 = Select(t=5, s=w1117, f=2 ("y")) -> (s? t:f=w1115:i32)
            n503 = global write "Results_plotter_Global.vi" "Ordinate"("Multi Ordinate") -> ()
            n504 = global write "Results_plotter_Global.vi" "Absisca"("Absisca") -> ()
            n505 = global write "Results_plotter_Global.vi" "Transpose"("Transpose") -> ()
            n506 = while {
              shift-right: [w1128] -> w1120
              shift-left: _ -> [w1129]
              tunnel: "color and symbol" -> [w1130]
              tunnel: w1115 -> [w1126]
              stop <- FALSE continue-if-true
              n507 = case shown="True" w1130 {
                tunnel: w1129 -> [w1137 w1139]
                tunnel: [w1136 w1139] -> w1128
                tunnel: w1126 -> [w1131 _]
                frame True {
                  n508 = Add(x=w1137, y=1) -> (x+y=w1134:i32)
                  n509 = local write "color and symbol"(FALSE ("color and symbol")) -> ()
                  n510 = Greater?(x=w1134, y=w1131) -> (0:w1135:bool)
                  n511 = Select(t=0, s=w1135, f=w1134) -> (s? t:f=w1136:i32)
                }
                frame False {
                }
              }
            }
            n512 = call "Plot_XY_data.vi"("Channel Values"=w1121, "Ordinate Strings"=w1112, "Swap color and symbol"=w1120, "Error Bar Chs"=w1111, "Accept Array"=w1123, "Filter 1 Strings"=w1125, "Filter 2 Strings"=w1124, "Ordinate"="Multi Ordinate", "Absisca"="Absisca", "Transpose"="Transpose") -> ("Accept Array Out"=→"Plotted Series":bool[][])  [unwired: 5 out]
          }
          frame #2 {
            n513 = Select(t="Intensity plot", s="Intensity Plot?", f="Add Legend and scales") -> (s? t:f=w1141:string)
            n514 = property on="Surface Area" class="DigNum (strict)"("Visible"="Intensity Plot?") -> ()  [unwired: 2 in, 2 out]
            n515 = property on="Surface Integral" class="DigNum (strict)"("Visible"="Intensity Plot?") -> ()  [unwired: 2 in, 2 out]
            n516 = property on="Surface Average" class="DigNum (strict)"("Visible"="Intensity Plot?") -> ()  [unwired: 2 in, 2 out]
            n517 = property on="X Ch Name" class="Ring (strict)"("Visible"="Intensity Plot?") -> ()  [unwired: 2 in, 2 out]
            n518 = property on="Y Ch Name" class="Ring (strict)"("Visible"="Intensity Plot?") -> ()  [unwired: 2 in, 2 out]
            n519 = property on="Z Ch Name" class="Ring (strict)"("Visible"="Intensity Plot?") -> ()  [unwired: 2 in, 2 out]
            n520 = property on="Point Size" class="Slide (strict)"("Visible"="Intensity Plot?") -> ()  [unwired: 2 in, 2 out]
            n521 = property on="No of Contours" class="DigNum (strict)"("Visible"="Intensity Plot?") -> ()  [unwired: 2 in, 2 out]
            n522 = property on="Slice mode" class="Enum (strict)"("Visible"="Intensity Plot?") -> ()  [unwired: 2 in, 2 out]
            n523 = property on="Plot Resolution" class="Bool (strict)"("Visible"="Intensity Plot?") -> ()  [unwired: 2 in, 2 out]
            n524 = property on="Update" class="Bool (strict)"("Visible"="Intensity Plot?") -> ()  [unwired: 2 in, 2 out]
          }
        }
      }
      frame "Add Legend and scales" {
        n525 = local read "Transpose"() -> (w1147:bool)
        n526 = global read "Results_plotter_Global.vi" "Plot Index values"() -> (w1150:dbl[][])
        n527 = global read "Results_plotter_Global.vi" "XY Graph Cluster"() -> (→"XY Plot":cluster{dbl[], dbl[]}[])
        n528 = Select(t=1 ("index (row)"), s=w1147, f=0 ("index (row)")) -> (s? t:f=w1144:i32)
        n529 = Index Array(array=w1150, index (row)=w1144) -> (element=w1149:dbl[])  [unwired: 1 in]
        n530 = Array Max & Min(array=w1149) -> (max value=w1148:dbl)  [unwired: 3 out]
        n531 = global read "Results_plotter_Global.vi" "Point info"() -> (w1155:T13)
        n532 = global read "Results_plotter_Global.vi" "Legend"() -> (w1156:string[])
        n533 = Greater?(x=w1148, y=2680560000.0) -> (0:w1152:bool)
        n534 = case shown="False" w1152 {
          tunnel: [w1167 u8 7 ("X Scale.Format & Precision:Precision")] -> w1151
          tunnel: w1148 -> [w1173 _]
          frame False {
            n535 = Absolute Value(x=w1173) -> (abs(x)=w1166:dbl)
            n536 = In Range and Coerce(upper limit=100000.0 ("y"), x=w1166, lower limit=0.0001) -> (In Range?=w1170:bool)  [unwired: 1 out]
            n537 = Select(t=u8 0 ("f"), s=w1170, f=u8 1) -> (s? t:f=w1167:u8)
          }
          frame True {
          }
        }
        n538 = local write "Warning!"("") -> ()
        n539 = for {
          tunnel: w1156 -> [w1190] mode=indexing
          tunnel: w1155 -> [w1187] mode=indexing
          tunnel: [w1188] -> w1160
          i -> [w1188]
          n540 = call "Abbreviate_string.vi"("Input String"=w1190, "Max String Length"=50) -> ("Output String"=w1181:string)
          n541 = Unbundle By Name(w1187) -> ("Point Style"=w1186:u8, "Fill/Pt. Color"=w1185:u32)
          n542 = String Length(string=w1181) -> (length=w1184:i32)
          n543 = Subtract(x=w1184, y=2) -> (x-y=w1182:i32)
          n544 = String Subset(string=w1181, length (rest)=w1182) -> (substring=w1180:string)  [unwired: 1 out]
          n545 = property on="XY Plot" class="XYGraph (strict)"("Active Plot"=w1188, "Plot.Plot Name"=w1180, "Plot.Point Style"=w1186, "Plot.Fill/Point Color"=w1185, "Plot.Plot Color"=w1185) -> ()  [unwired: 2 in, 2 out]
        }
        n546 = Increment(x=w1160) -> (x+1=w1159:i32)
        n547 = property on="XY Plot" class="XYGraph (strict)"("X Scale.Format & Precision:Format"=w1151) -> ()  [unwired: 2 in, 2 out]
        n548 = for {
          N: 10 -> [_]
          tunnel: w1159 -> [w1178]
          i -> [w1179]
          w1175 = u32 0
          n549 = Add(x=w1178, y=w1179) -> (x+y=w1177:i32)
          n550 = property on="XY Plot" class="XYGraph (strict)"("Active Plot"=w1177, "Plot.Plot Name"="" ("Write Attribute"), "Plot.Plot Color"=w1175, "Plot.Fill/Point Color"=w1175) -> ()  [unwired: 2 in, 2 out]
        }
      }
      frame "Add Axis names" {
        n551 = local read "Multi Ordinate"() -> (w1205:i32[])
        n552 = for {
          tunnel: w1205 -> [w1222] mode=indexing
          shift-right: [w1219] -> w1198
          shift-left: "" -> [w1218]
          tunnel: w1206 -> [w1221]
          tunnel: [w1214] -> w1197
          i -> [w1214]
          n553 = Index Array(array=w1221, index=w1222) -> (element=w1220:string)
          n554 = String Length(string=w1218) -> (length=w1217:i32)
          n555 = Less?(x=w1217, y=30) -> (x < y?=w1215:bool)
          n556 = case shown="True" w1215 {
            tunnel: w1220 -> [_ w1227]
            tunnel: [w1223 w1226] -> w1219
            tunnel: w1218 -> [w1223 w1224]
            frame False {
            }
            frame True {
              n557 = Concatenate Strings(w1224, w1227, "   ") -> (w1226:string)
            }
          }
        }
        n558 = Greater Than 0?(x=w1197) -> (x > 0?=w1195:bool)
        n559 = local read "Transpose"() -> (w1208:bool)
        n560 = local read "Absisca"() -> (w1209:u16)
        n561 = Index Array(array=w1206, index=w1209) -> (element=w1207:string)
        n562 = String Length(string=w1198) -> (length=w1201:i32)
        n563 = Empty String/Path?(string/path="Ordinate Name") -> (empty?=w1196:bool)
        n564 = Subtract(x=w1201, y=3) -> (x-y=w1199:i32)
        n565 = Compound Arithmetic op=AND(invert w1196, w1195) -> (w1194:bool)
        n566 = String Subset(string=w1198, length (rest)=w1199) -> (substring=w1193:string)  [unwired: 1 out]
        n567 = Select(t="Ordinate Name", s=w1194, f=w1193) -> (s? t:f=w1191:string)
        n568 = case shown="False" w1208 {
          tunnel: [w1228 w1231] -> w1204
          tunnel: w1191 -> [w1229 w1231]
          tunnel: [w1229 w1230] -> w1203
          tunnel: w1207 -> [w1228 w1230]
          frame False {
          }
          frame True {
          }
        }
        n569 = global write "Results_plotter_Global.vi" "X Axis Name"(w1204) -> ()
        n570 = global write "Results_plotter_Global.vi" "Y Axis Name"(w1203) -> ()
        n571 = global write "Results_plotter_Global.vi" "Value plotted Name"(w1191) -> ()
        n572 = property on="XY Plot" class="XYGraph (strict)"("X Scale.Name Label.Text"=w1204, "Y Scale.Name Label.Text"=w1203) -> ()  [unwired: 2 in, 2 out]
      }
      frame "Intensity plot" {
        # "Max"
        # "Min"
        n573 = global read "Results_plotter_Global.vi" "XY Graph Cluster"() -> (w1232:cluster{dbl[], dbl[]}[])
        n574 = local read "Tolerances"() -> (w1237:dbl[])
        n575 = local read "Absisca"() -> (w1236:u16)
        n576 = local read "Transpose"() -> (w1233:bool)
        n577 = stacked-sequence {
          seq-local: [w1250 _ _ _ _ _ _ _ _ _ _ _ _] -> [_ _ _ w1315 w1322 _ w1347 _ _ _ _ _ _]
          seq-local: [_ w1266 _ _ _ _ _ _ _ _ _ _ _] -> [_ _ _ _ w1321 _ w1346 _ _ _ _ _ _]
          seq-local: [_ _ w1298 _ _ _ _ _ _ _ _ _ _] -> [_ _ _ _ _ _ w1355 _ _ _ _ _ _]
          seq-local: [_ _ _ _ _ _ w1357 _ _ _ _ _ _] -> [_ _ _ _ _ _ _ _ w1381 _ _ _ _]
          seq-local: [_ _ _ _ _ _ w1356 _ _ _ _ _ _] -> [_ _ _ _ _ _ _ _ w1382 _ _ _ _]
          seq-local: [_ w1262 _ _ _ _ _ _ _ _ _ _ _] -> [_ _ _ _ _ _ _ _ _ w1446 _ _ _]
          seq-local: [_ _ _ w1313 _ _ _ _ _ _ _ _ _] -> [_ _ _ _ w1320 _ w1351 _ _ _ _ _ _]
          seq-local: [_ _ _ _ _ _ _ _ _ _ _ w1472 _] -> [_ _ _ _ _ _ _ _ _ _ _ _ w1522]
          seq-local: [_ _ _ _ _ _ _ _ _ _ _ w1471 _] -> [_ _ _ _ _ _ _ _ _ _ _ _ w1523]
          seq-local: [_ _ _ w1312 _ _ _ _ _ _ _ _ _] -> [_ _ _ _ _ w1335 _ _ _ _ _ _ _]
          seq-local: [_ _ _ _ _ _ _ _ _ _ _ w1469 _] -> [_ _ _ _ _ _ _ _ _ _ _ _ w1515]
          tunnel: [_ _ _ TRUE _ _ _ _ _ _ _ _ _] -> w1243
          tunnel: [_ _ _ _ _ _ _ _ _ _ _ _ "Analyse Plot Space"] -> w1242
          tunnel: w1240 -> [w1247 _ _ _ _ _ _ _ _ _ _ _ _]
          tunnel: w1241 -> [w1248 _ w1299 _ _ _ _ _ _ w1427 _ _ _]
          tunnel: [w1248 _ _ _ _ _ _ _ _ _ _ _ _] -> w1239
          tunnel: [w1247 _ _ _ _ _ _ _ _ _ _ _ _] -> w1238
          tunnel: w1237 -> [w1252 _ _ _ _ _ _ _ _ _ _ _ _]
          tunnel: w1232 -> [w1251 _ _ w1317 _ _ _ _ _ _ _ _ _]
          tunnel: w1236 -> [w1249 _ _ _ _ _ _ _ _ w1443 _ _ _]
          tunnel: w1233 -> [w1246 _ _ w1314 _ _ w1359 _ _ w1441 _ _ _]
          tunnel: [_ w1267 _ _ _ _ _ _ _ _ _ _ _] -> w1235
          tunnel: w1234 -> [_ w1267 _ _ _ _ _ _ _ w1428 _ _ _]
          frame #0 {
            n578 = Not(x=w1246) -> (.not. x?=w1245:bool)
            n579 = for {
              tunnel: w1251 -> [w1261] mode=indexing
              tunnel: w1245 -> [w1258]
              shift-right: [w1256] -> w1253
              shift-left: dbl[] [] -> [w1257]
              n580 = Unbundle(w1261) -> (w1260:dbl[], w1259:dbl[])
              n581 = Select(t=w1260, s=w1258, f=w1259) -> (s? t:f=w1255:dbl[])
              n582 = Build Array (concatenate)(w1257, w1255) -> (w1256:dbl[])
            }
            n583 = Index Array(array=w1252, index=w1249) -> (element=w1244:dbl)
            n584 = call "Numeric_bins.vi"("Values"=w1253, "Tolerance"=w1244) -> ("Bin Centres"=w1250:dbl[])  [unwired: 2 out]
          }
          frame #1 {
            n585 = local read "Filter Bins 2"() -> (w1268:i32[])
            n586 = local read "Filter Bins 1"() -> (w1270:i32[])
            n587 = Array Size(array=w1268) -> (size(s)=w1272:i32)
            n588 = Array Size(array=w1270) -> (size(s)=w1273:i32)
            n589 = Greater?(x=w1273, y=w1272) -> (0:w1271:bool)
            n590 = case shown="True" w1271 {
              tunnel: w1270 -> [_ w1295]
              tunnel: [w1291 w1295] -> w1269
              tunnel: [w1292 w1294] -> w1264
              tunnel: w1268 -> [w1291 _]
              tunnel: [1 0] -> w1262
              frame False {
                n591 = property on="Filter Bins 2" class="LstBox (strict)"() -> ("Item Names"=w1292:string[])  [unwired: 2 in, 2 out]
              }
              frame True {
                n592 = property on="Filter Bins 1" class="LstBox (strict)"() -> ("Item Names"=w1294:string[])  [unwired: 2 in, 2 out]
              }
            }
            n593 = Array Size(array=w1264) -> (size(s)=w1263:i32)
            n594 = for {
              tunnel: w1269 -> [w1278] mode=indexing
              tunnel: w1264 -> [w1284]
              shift-right: [w1281] -> w1266
              shift-left: dbl[] [] -> [w1282]
              tunnel: w1263 -> [w1277]
              n595 = Index Array(array=w1284, index=w1278) -> (element=w1280:string)
              n596 = Less?(x=w1278, y=w1277) -> (x < y?=w1276:bool)
              n597 = Match Pattern(string=w1280, regular expression=" (0)") -> (offset past match=w1279:i32)  [unwired: 4 out]
              n598 = Less Than 0?(x=w1279) -> (x < 0?=w1275:bool)
              n599 = And(x=w1275, y=w1276) -> (x .and. y?=w1274:bool)
              n600 = case shown="True" w1274 {
                tunnel: w1282 -> [w1285 w1289]
                tunnel: [w1285 w1288] -> w1281
                tunnel: w1280 -> [_ w1287]
                frame False {
                }
                frame True {
                  n601 = Fract/Exp String To Number(string=w1287) -> (number=w1286:dbl)  [unwired: 4 out]
                  n602 = Build Array (concatenate)(w1289, w1286) -> (w1288:dbl[])
                }
              }
            }
          }
          frame #2 {
            n603 = local read "Template"() -> (w1297:path)
            n604 = call "Valid_Path.vi"("Filename"=w1297) -> ("Valid Path?"=w1296:bool)
            n605 = case shown="True" w1296 {
              tunnel: w1297 -> [_ w1309]
              tunnel: w1299 -> [_ w1308]
              tunnel: [nan w1305] -> w1298
              frame False {
              }
              frame True {
                n606 = local read "Multi Ordinate"() -> (w1304:i32[])
                n607 = call "Read_Write_Template.vi"("Template File"=w1309, "Mode"=Global_mode."Read Global", "Channel names In"=w1308, "Data type"="Minimum Value") -> ("1D Info Out"=w1307:string[])  [unwired: 4 in, 7 out]
                n608 = Index Array(array=w1304, index=0 ("Index")) -> (element=w1303:i32)
                n609 = Index Array(array=w1307, index=w1303) -> (element=w1306:string)
                n610 = Fract/Exp String To Number(string=w1306, default (0 dbl)=nan) -> (number=w1305:dbl)  [unwired: 3 out]
              }
            }
          }
          frame #3 {
            n611 = call "Grid_Data.vi"("Transpose"=w1314, "XY Graph"=w1317, "Bin Centres"=w1315) -> ("No of Duplicates"=w1312:i32, "Grided data"=w1313:dbl[][])
          }
          frame #4 {
            n612 = for {
              tunnel: w1322 -> [w1327]
              tunnel: w1321 -> [w1326] mode=indexing
              tunnel: w1320 -> [w1325] mode=indexing
              shift-right: [w1323] -> w1318
              shift-left: dbl[][] [] -> [w1324]
              n613 = for {
                tunnel: w1327 -> [w1333] mode=indexing
                tunnel: w1326 -> [w1328]
                tunnel: w1325 -> [w1332] mode=indexing
                shift-right: [w1329] -> w1323
                shift-left: w1324 -> [w1331]
                n614 = Build Array(w1333, w1328, w1332) -> (w1330:dbl[])
                n615 = Build Array (concatenate)(w1331, w1330) -> (w1329:dbl[][])
              }
            }
            n616 = global write "Results_plotter_Global.vi" "Intensity Plot data in rows"(w1318) -> ()
          }
          frame #5 {
            n617 = case shown="1, Default" w1335 {
              tunnel: w1335 -> [_ w1339]
              tunnel: ["" w1337] -> w1334
              frame 0 {
              }
              frame 1, Default {
                n618 = Format Into String(format string="The Intensity Plot has %d duplicate points which have been averged together.", w1339) -> (resulting string=w1337:string)  [unwired: 2 in, 1 out]
              }
            }
            "Warning!" <- w1334
          }
          frame #6 {
            n619 = call "Insert_extra_rows_and_col.vi"("Row Values In"=w1346, "Additional Row Values"="Additional X Values", "Column Values In"=w1347, "Data In"=w1351, "Additional Column Values"="Additional Y Values") -> ("Row Values Out"=w1348:dbl[], "Column Values Out"=w1349:dbl[], "Data Out"=w1350:dbl[][])  [unwired: 2 out]
            n620 = Select(t="Resolution", s="Plot Resolution", f=0.0) -> (s? t:f=w1341:dbl)
            n621 = call "2D_interpolation.vi"("X Axis Current"=w1349, "Min Z Value In"=w1355, "Y axis Current"=w1348, "Bkgnd Value"="Bkgnd Value", "Plot In"=w1350, "Increment Value"=w1341, "Transpose"=w1359, "Point Size"="Point Size") -> ("min Z value"=w1357:dbl, "max Z value"=w1356:dbl, "Increment Value Out"=w1345:dbl, "Plot Out"=→"Intensity Graph":dbl[][])  [unwired: 4 out]
            n622 = local write "Resolution"(w1345) -> ()
          }
          frame #7 {
            n623 = global read "Results_plotter_Global.vi" "X Scale"() -> (w1367:cluster{"Xo":dbl, "delta X":dbl})
            n624 = global read "Results_plotter_Global.vi" "Y Scale"() -> (w1363:cluster{"Xo":dbl, "delta X":dbl})
            n625 = global read "Results_plotter_Global.vi" "Y Max"() -> (w1364:dbl)
            n626 = global read "Results_plotter_Global.vi" "X Max"() -> (w1365:dbl)
            n627 = Unbundle By Name(w1363) -> ("Xo"=w1362:dbl)
            n628 = Unbundle By Name(w1367) -> ("Xo"=w1366:dbl)
            n629 = Subtract(x=w1364, y=w1362) -> (x-y=w1368:dbl)
            n630 = Subtract(x=w1365, y=w1366) -> (x-y=w1377:dbl)
            n631 = Greater?(x=w1377, y=5.0) -> (0:w1375:bool)
            n632 = Greater?(x=w1368, y=5.0) -> (0:w1370:bool)
            n633 = Select(t=u8 0 ("Write Attribute"), s=w1375, f=u8 3) -> (s? t:f=w1361:u8)
            n634 = Select(t=u8 0 ("Write Attribute"), s=w1370, f=u8 3) -> (s? t:f=w1360:u8)
            n635 = property on="Intensity Graph" class="IntGraph (strict)"("X Scale.Offset and Multiplier"=w1367, "X Scale.Range:Maximum"=w1365, "Y Scale.Offset and Multiplier"=w1363, "Y Scale.Range:Maximum"=w1364, "X Scale.Format & Precision:Precision"=w1361, "Y Scale.Format & Precision:Precision"=w1360) -> ()  [unwired: 2 in, 2 out]
          }
          frame #8 {
            n636 = Greater Than 0?(x=w1382) -> (x > 0?=w1379:bool)
            n637 = Less Than 0?(x=w1381) -> (x < 0?=w1380:bool)
            n638 = And(x=w1379, y=w1380) -> (x .and. y?=w1378:bool)
            n639 = case shown="True" w1378 {
              tunnel: w1382 -> [w1411 w1425]
              tunnel: [w1419 w1423] -> w1384
              tunnel: w1381 -> [w1407 w1420]
              frame True {
                (unwired) u32 3743
                (unwired) u32 16721152
                n640 = Absolute Value(x=w1407) -> (abs(x)=w1406:dbl)
                n641 = Absolute Value(x=w1411) -> (abs(x)=w1413:dbl)
                n642 = Absolute Value(x=w1407) -> (abs(x)=w1414:dbl)
                n643 = Max & Min(x=w1413, y=w1414) -> (max(x,y)=w1409:dbl)  [unwired: 1 out]
                n644 = Divide(x=w1406, y=w1409) -> (x/y=w1400:dbl)
                n645 = Subtract(x=1.0, y=w1400) -> (x-y=w1399:dbl)
                n646 = Multiply(x=w1399, y=u32 255) -> (x*y=w1405:dbl)
                n647 = To Unsigned Long Integer(number=w1405) -> (unsigned 32bit integer=w1389:u32)
                n648 = Multiply(x=w1389, y=u32 256) -> (x*y=w1391:u32)
                n649 = Multiply(x=w1389, y=u32 65536) -> (x*y=w1388:u32)
                n650 = Compound Arithmetic op=ADD(w1388, w1391, u32 255) -> (w1387:u32)
                n651 = Bundle("min Z value"=w1407, w1387) -> (w1416:cluster{"min Z value":dbl, u32})  [unwired: 1 out]
                n652 = Divide(x=w1411, y=w1409) -> (x/y=w1404:dbl)
                n653 = Bundle("max Z value"=0.0, u32 16777215) -> (w1415:cluster{"max Z value":dbl, u32})  [unwired: 1 out]
                n654 = Subtract(x=1.0, y=w1404) -> (x-y=w1402:dbl)
                n655 = Multiply(x=w1402, y=u32 255) -> (x*y=w1398:dbl)
                n656 = To Unsigned Long Integer(number=w1398) -> (unsigned 32bit integer=w1385:u32)
                n657 = Multiply(x=w1385, y=u32 256) -> (x*y=w1395:u32)
                n658 = Compound Arithmetic op=ADD(w1385, w1395, u32 16711680) -> (w1386:u32)
                n659 = Bundle("max Z value"=w1411, w1386) -> (w1418:cluster{"max Z value":dbl, u32})  [unwired: 1 out]
                n660 = Build Array(w1418, w1416) -> (w1417:cluster{"min Z value":dbl, u32}[])
                n661 = Build Array (concatenate)(w1417, w1415) -> (w1419:cluster{"max Z value":dbl, u32}[])
              }
              frame False {
                n662 = Bundle("max Z value"=w1425, u32 16721152) -> (w1422:cluster{"max Z value":dbl, u32})  [unwired: 1 out]
                n663 = Bundle("min Z value"=w1420, u32 3743) -> (w1421:cluster{"min Z value":dbl, u32})  [unwired: 1 out]
                n664 = Build Array(w1422, w1421) -> (w1423:cluster{"min Z value":dbl, u32}[])
              }
            }
            n665 = property on="Intensity Graph" class="IntGraph (strict)"("Ignore Array"=FALSE ("Write Attribute"), "Z Scale.Marker Values[]"=w1384) -> ()  [unwired: 2 in, 2 out]
          }
          frame #9 {
            n666 = local read "Filter Array"() -> (w1445:u16[])
            n667 = Index Array(array=w1445, index=w1446) -> (element=w1444:u16)
            n668 = Decrement(x=w1444) -> (x-1=w1442:u16)
            n669 = local read "Multi Ordinate"() -> (w1432:i32[])
            n670 = Index Array(array=w1428, index=w1442) -> (element=w1436:string)
            n671 = Index Array(array=w1428, index=w1443) -> (element=w1435:string)
            n672 = case shown="False" w1441 {
              tunnel: [w1448 w1450] -> w1434
              tunnel: w1436 -> [w1448 w1449]
              tunnel: w1435 -> [w1447 w1450]
              tunnel: [w1447 w1449] -> w1433
              frame False {
              }
              frame True {
              }
            }
            n673 = Index Array(array=w1432, index=0) -> (element=w1430:i32)
            n674 = Index Array(array=w1427, index=w1430) -> (element=w1429:string)
            n675 = global write "Results_plotter_Global.vi" "Value plotted Name"(w1429) -> ()
            n676 = property on="Intensity Graph" class="IntGraph (strict)"("X Scale.Name Label.Text"=w1433, "Y Scale.Name Label.Text"=w1434) -> ()  [unwired: 2 in, 2 out]
            n677 = global write "Results_plotter_Global.vi" "Y Axis Name"(w1433) -> ()
            n678 = global write "Results_plotter_Global.vi" "X Axis Name"(w1434) -> ()
            n679 = Format Into String(format string="Add %s values", w1436) -> (resulting string=→"First Add label":string)  [unwired: 2 in, 1 out]
            n680 = Format Into String(format string="Add %s values", w1435) -> (resulting string=→"2nd Add label":string)  [unwired: 2 in, 1 out]
          }
          frame #10 {
            n681 = property on="Intensity Graph" class="IntGraph (strict)"() -> ("Color Table"=w1452:u32[])  [unwired: 2 in, 2 out]
            n682 = Increment(x="No of Contours") -> (x+1=w1453:i32)
            n683 = Divide(x=255, y=w1453) -> (x/y=w1457:dbl)
            n684 = To Long Integer(number=w1457) -> (32bit integer=w1456:i32)
            n685 = for {
              tunnel: w1456 -> [w1465]
              tunnel: [w1462] -> w1451 mode=indexing
              tunnel: w1452 -> [w1461] mode=indexing
              tunnel: u32 0 -> [w1460]
              i -> [w1466]
              n686 = Increment(x=w1466) -> (x+1=w1463:i32)
              n687 = Quotient & Remainder(x=w1463, y=w1465) -> (x-y*floor(x/y)=w1464:i32)  [unwired: 1 out]
              n688 = case shown="0" w1464 {
                tunnel: [w1467 w1468] -> w1462
                tunnel: w1461 -> [_ w1468]
                tunnel: w1460 -> [w1467 _]
                frame 0 {
                }
                frame 1, Default {
                }
              }
            }
            n689 = property on="Intensity Graph" class="IntGraph (strict)"("Ignore Array"=TRUE ("Write Attribute"), "Color Table"=w1451) -> ()  [unwired: 2 in, 2 out]
          }
          frame #11 {
            n690 = global read "Results_plotter_Global.vi" "Raw Interpolation"() -> (w1470:dbl[][])
            n691 = Add Array Elements(numeric array=w1470) -> (sum=w1469:dbl)
            n692 = Array Size(array=w1470) -> (size(s)=w1480:i32[])
            n693 = Decrement(x=w1480) -> (x-1=w1478:i32[])
            n694 = Index Array(array=w1478, index=0) -> (element=w1479:i32)
            n695 = Index Array(array=w1478, index=1) -> (element=w1475:i32)
            n696 = for {
              N: w1479 -> [_]
              tunnel: w1470 -> [w1488]
              tunnel: w1475 -> [w1487]
              shift-right: [w1483] -> w1472
              shift-left: 0.0 -> [w1484]
              shift-right: [w1482] -> w1471
              shift-left: 0 -> [w1481]
              i -> [w1486]
              n697 = Increment(x=w1486) -> (x+1=w1485:i32)
              n698 = for {
                N: w1487 -> [_]
                tunnel: w1488 -> [w1497]
                tunnel: w1486 -> [w1502]
                tunnel: w1485 -> [w1500]
                shift-right: [w1493] -> w1483
                shift-left: w1484 -> [w1492]
                shift-right: [w1489] -> w1482
                shift-left: w1481 -> [w1490]
                i -> [w1501]
                n699 = Increment(x=w1501) -> (x+1=w1499:i32)
                n700 = Index Array(array=w1497, index (row)=w1502, index (col)=w1499) -> (element=w1498:dbl)
                n701 = Index Array(array=w1497, index (row)=w1500, index (col)=w1499) -> (element=w1495:dbl)
                n702 = Index Array(array=w1497, index (row)=w1502, index (col)=w1501) -> (element=w1503:dbl)
                n703 = Index Array(array=w1497, index (row)=w1500, index (col)=w1501) -> (element=w1496:dbl)
                n704 = Compound Arithmetic op=ADD(w1503, w1498, w1496, w1495) -> (w1491:dbl)
                n705 = Not A Number/Path/Refnum?(number/path/refnum=w1491) -> (NaN/Path/Refnum?=w1494:bool)
                n706 = case shown="False" w1494 {
                  tunnel: [w1507 w1511] -> w1493
                  tunnel: w1492 -> [w1509 w1511]
                  tunnel: w1491 -> [w1508 _]
                  tunnel: [w1506 w1510] -> w1489
                  tunnel: w1490 -> [w1505 w1510]
                  frame False {
                    n707 = Add(x=w1508, y=w1509) -> (x+y=w1507:dbl)
                    n708 = Add(x=1, y=w1505) -> (x+y=w1506:i32)
                  }
                  frame True {
                  }
                }
              }
            }
          }
          frame #12 {
            n709 = local read "Resolution"() -> (w1524:dbl)
            n710 = Divide(x=w1522, y=4.0) -> (x/y=w1520:dbl)
            n711 = Multiply(x=w1524, y=w1524) -> (x*y=w1516:dbl)
            n712 = Multiply(x=w1516, y=w1515) -> ()  [unwired: 1 out]
            n713 = Multiply(x=w1516, y=w1523) -> (x*y=w1517:dbl)
            "Surface Area" <- w1517
            n714 = Multiply(x=w1516, y=w1520) -> (x*y=w1513:dbl)
            "Surface Integral" <- w1513
            n715 = global write "Results_plotter_Global.vi" "Surface Area"(w1517) -> ()
            n716 = global write "Results_plotter_Global.vi" "Surface Integral"(w1513) -> ()
            n717 = Divide(x=16666667, y=w1513) -> (x/y=→"Uadvec":dbl)
            n718 = Divide(x=w1513, y=w1517) -> (x/y=→"Surface Average":dbl)
          }
        }
      }
      frame "Analyse Plot Space" {
        n719 = case shown="True" "Show Plot Space Analysis" {
          tunnel: w1529 -> [_ w1539]
          tunnel: w1526 -> [_ w1538]
          frame False {
          }
          frame True {
            w1535 = TRUE  # Summarise All
            n720 = global read "Results_plotter_Global.vi" "Plot Index values"() -> (w1533:dbl[][])
            n721 = Index Array(array=w1533, index (row)=2) -> (element=w1532:dbl[])  [unwired: 1 in]
            n722 = To Long Integer(number=w1532) -> (32bit integer=w1531:i32[])
            n723 = for {
              tunnel: w1531 -> [w1542] mode=indexing
              tunnel: w1539 -> [w1541]
              tunnel: [w1540] -> w1536 mode=indexing
              n724 = Index Array(array=w1541, index (row)=w1542) -> (element=w1540:string[])  [unwired: 1 in]
            }
            n725 = call "Summarise.vi"("Channel Names"=w1538, "Data"=w1536, "Summarise All"=w1535) -> ("Summary"=w1537:string[][])  [unwired: 2 in]
            n726 = call "Plot_Space_Analysis.vi"("Table"=w1537) -> ()
          }
        }
      }
      frame "Vector Plot" {
        n727 = flat-sequence {
          tunnel: w1547 -> [w1549]
          tunnel: w1545 -> [w1548]
          frame #0 {
            n728 = local read "Template"() -> (w1550:path)
            n729 = call "Vector_Plotting.vi"("Template Filename"=w1550, "Data"=w1548, "Channel Names"=w1549) -> ()  [unwired: 1 out]
          }
          frame #1 {
            n730 = local write "Vector Plot?"(FALSE ("Vector Plot?")) -> ()
          }
        }
      }
      frame "What to do next?" {
        n731 = local read "Warning!"() -> (w1560:string)
        n732 = Empty String/Path?(string/path=w1560) -> (empty?=w1559:bool)
        n733 = Not(x=w1559) -> (.not. x?=w1558:bool)
        n734 = property on="Warning!" class="Str" props=["Visible", "Blinking", "Caption"]("Visible"=w1558, "Blinking"=w1558) -> ()  [unwired: 2 in, 3 out]
        n735 = case shown="False" "Add results file" {
          tunnel: [w1582 "More files options"] -> w1563
          tunnel: "Add results file" -> [_ _]
          tunnel: "Edit Template File" -> [w1573 _]
          frame False {
            n736 = Select(t="Edit template file", s=w1573, f="What to do next 2nd?") -> (s? t:f=w1571:string)
            n737 = Or(x="Save Plot data", y="Save Surface Fit") -> (x .or. y?=w1575:bool)
            n738 = Select(t="Save Plot Data", s=w1575, f=w1571) -> (s? t:f=w1578:string)
            n739 = Select(t="Create Plot summary", s="Save Plot as jpg", f=w1578) -> (s? t:f=w1569:string)
            n740 = Select(t="Save Data in Rows", s="Save Data in Rows", f=w1569) -> (s? t:f=w1582:string)
          }
          frame True {
            n741 = local write "Add results file"(FALSE) -> ()
          }
        }
        n742 = Select(t="End", s="stop", f=w1563) -> (s? t:f=w1554:string)
        n743 = Select(t="Vector Plot", s="Vector Plot?", f=w1554) -> (s? t:f=w1553:string)
      }
      frame "What to do next 2nd?" {
        n744 = local read "Empty"() -> (w1605:bool)
        n745 = local read "Last used Template"() -> (w1593:path)
        n746 = local read "Template"() -> (w1585:path)
        n747 = Select(t="Empty Results file array", s=w1605, f="What to do next 3rd?") -> (s? t:f=w1588:string)
        n748 = global write "Results_plotter_Global.vi" "Template"(w1585) -> ()
        n749 = Not Equal?(x=w1593, y=w1585) -> (x != y?=w1592:bool)
        n750 = Select(t="What type of row averaging?", s="Save Averaged rows", f=w1588) -> (s? t:f=w1600:string)
        n751 = case shown="True" "Delete Plotted data from file" {
          tunnel: [w1633 "Full Res file manipulator" ("t")] -> w1598
          tunnel: w1600 -> [w1633 _]
          frame False {
          }
          frame True {
            n752 = local write "Plotted rows only?"(TRUE ("Save Plotted rows only?")) -> ()
            n753 = local write "Mode"(Plotter_Mode."Delete unwanted rows" ("Mode")) -> ()
          }
        }
        n754 = case shown="True" "Add /Edit metadata" {
          tunnel: [w1610 w1625] -> w1590
          tunnel: w1598 -> [w1611 w1626]
          tunnel: w1596 -> [_ w1624]
          tunnel: "Reload Files" -> [w1612 _]
          tunnel: [string[] [] ("New Chs Out") w1618] -> w1587
          tunnel: [string[][] [] w1617] -> w1586
          frame False {
            n755 = Select(t="Initialise", s=w1612, f=w1611) -> (s? t:f=w1610:string)
          }
          frame True {
            n756 = local read "Result files to read"() -> (w1619:path[])
            n757 = call "Edit_Channel_Panel.vi"("All Channel names"=w1624, "Result files to read"=w1619) -> ("New Values Out"=w1632:string[], "New Chs Out"=w1618:string[], "Cancel Out"=w1621:bool, "Edit Raw Data Header Info Out"=w1615:bool, "Plotted rows only?"=w1631:bool, "Edit Raw data files?"=→"Edit Raw DF?":bool, "Raw data files in Orig Positions?"=→"Raw DF in Orig Pos?":bool, "Mode"=w1629:T1)  [unwired: 6 out]
            "Edit Raw Data Header Info" <- w1615
            n758 = Array Size(array=w1618) -> (size(s)=w1628:i32)
            n759 = Build Array(w1632) -> (w1617:string[][])
            n760 = local write "Add /Edit metadata"(FALSE ("Add /Edit metadata")) -> ()
            n761 = Greater Than 0?(x=w1628) -> (x > 0?=w1616:bool)
            n762 = local write "Plotted rows only?"(w1631) -> ()
            n763 = Or(x=w1615, y=w1616) -> (x .or. y?=w1614:bool)
            n764 = local write "Mode"(w1629) -> ()
            n765 = Compound Arithmetic op=AND(invert w1621, w1614) -> (w1620:bool)
            n766 = Select(t="Full Res file manipulator", s=w1620, f=w1626) -> (s? t:f=w1625:string)
          }
        }
        n767 = global write "Results_plotter_Global.vi" "New Chs In"(w1587) -> ()
        n768 = global write "Results_plotter_Global.vi" "New Values In"(w1586) -> ()
        n769 = Select(t="Initialise", s=w1592, f=w1590) -> (s? t:f=w1589:string)
      }
      frame "What to do next 3rd?" {
        n770 = local read "Show Results Space Analysis"() -> (w1648:bool)
        n771 = local read "Show Plot Space Analysis"() -> (w1647:bool)
        n772 = while {
          shift-right: [w1671] -> _
          shift-left: _ -> [w1670]
          shift-left: _ -> [w1669]
          shift-left: _ -> [w1668]
          tunnel: w1648 -> [w1671]
          shift-right: [w1676] -> _
          shift-left: _ -> [w1675]
          shift-left: _ -> [w1674]
          shift-left: _ -> [w1673]
          tunnel: w1647 -> [w1676]
          tunnel: [w1672] -> w1646
          tunnel: [w1667] -> w1645
          stop <- TRUE stop-if-true
          n773 = Compound Arithmetic op=AND(w1671, w1670, w1669, w1668) -> (w1667:bool)
          n774 = Compound Arithmetic op=AND(w1676, w1675, w1674, w1673) -> (w1672:bool)
        }
        n775 = Select(t="Run Calculation Routine", s="Calculate new metadata", f="Time to save setup?") -> (s? t:f=w1654:string)
        n776 = case shown="True" w1646 {
          frame False {
          }
          frame True {
            n777 = Open VI Reference(vi path="Plot_Space_Analysis.vi" ("VI path")) -> (vi reference=w1688:refnum<vi>, error out=w1687:errorcluster)  [unwired: 1 in, 4 out]
            n778 = property class="VI"(reference=w1688, error in=w1687) -> (reference out=w1686:refnum<vi>, error out=w1685:errorcluster, "Front Panel Window:Open"=w1683:bool)
            n779 = local write "Show Plot Space Analysis"(w1683) -> ()
            n780 = Close Reference(reference=w1686, error in (no error)=w1685) -> ()  [unwired: 1 out]
          }
        }
        n781 = case shown="True" w1645 {
          frame False {
          }
          frame True {
            n782 = Open VI Reference(vi path="Results_Space_Analysis.vi" ("VI path")) -> (vi reference=w1682:refnum<vi>, error out=w1681:errorcluster)  [unwired: 1 in, 4 out]
            n783 = property class="VI"(reference=w1682, error in=w1681) -> (reference out=w1680:refnum<vi>, error out=w1679:errorcluster, "Front Panel Window:Open"=w1677:bool)
            n784 = local write "Show Results Space Analysis"(w1677) -> ()
            n785 = Close Reference(reference=w1680, error in (no error)=w1679) -> ()  [unwired: 1 out]
          }
        }
        n786 = Select(t="Save Setup", s="Save Setup", f=w1654) -> (s? t:f=w1651:string)
        n787 = Select(t="Choose Setup file", s="Load Setup", f=w1651) -> (s? t:f=w1644:string)
        n788 = Or(x="Kill Point", y="Process Point") -> (x .or. y?=w1641:bool)
        n789 = Select(t="Process cursor point", s=w1641, f=w1644) -> (s? t:f=w1637:string)
        n790 = case shown="True" "Post Process Plotted Data" {
          tunnel: [w1662 "Full Res file manipulator" ("t")] -> w1638
          tunnel: w1637 -> [w1662 _]
          frame False {
          }
          frame True {
            n791 = local write "Plotted rows only?"(TRUE ("Plotted rows only?")) -> ()
            n792 = local write "Mode"(Plotter_Mode."Post Process Plotted Rows" ("Mode")) -> ()
          }
        }
      }
      frame "Time to save setup?" {
        n793 = stacked-sequence {
          seq-local: [w1698 _] -> [_ w1739]
          seq-local: [w1697 _] -> [_ w1738]
          tunnel: [w1706 _] -> w1691
          tunnel: w1690 -> [w1696 _]
          tunnel: [w1695 _] -> w1689
          frame #0 {
            n794 = while {
              shift-right: [w1728] -> _
              shift-left: _ -> [w1726]
              shift-right: [w1715] -> _
              shift-left: _ -> [w1723]
              tunnel: [w1715] -> w1705
              tunnel: [w1714] -> w1704
              shift-right: [w1716] -> _
              shift-left: _ -> [w1722]
              tunnel: [w1720] -> w1699
              tunnel: [w1717] -> w1700
              tunnel: [w1716] -> w1701
              tunnel: [w1713] -> w1697
              tunnel: w1696 -> [w1708]
              tunnel: [w1707] -> w1695
              stop <- FALSE continue-if-true
              n795 = Get Date/Time In Seconds() -> (seconds since 1Jan1904=w1724:timestamp)
              n796 = To Double Precision Float(number=w1724) -> (double precision float=w1727:dbl)
              n797 = local read "Show Plot Space Analysis"() -> (w1716:bool)
              n798 = Subtract(x=w1727, y=w1726) -> (x-y=w1730:dbl)
              n799 = local read "Show Results Space Analysis"() -> (w1715:bool)
              n800 = Greater?(x=w1730, y=200.0) -> (0:w1711:bool)
              n801 = Greater?(x=w1708, y=300) -> (0:w1710:bool)
              n802 = And(x=w1711, y=w1710) -> (x .and. y?=w1709:bool)
              n803 = case shown="True" w1709 {
                tunnel: [w1733 w1737] -> w1728
                tunnel: w1727 -> [_ w1737]
                tunnel: w1726 -> [w1733 _]
                tunnel: ["Check modification dates?" "Save Setup"] -> w1719
                tunnel: [TRUE w1734] -> w1707
                frame False {
                }
                frame True {
                  n804 = global read "Trav_pos_global.vi" "Estimated Completion time"() -> (w1736:string)
                  n805 = Empty String/Path?(string/path=w1736) -> (empty?=w1734:bool)
                }
              }
              n806 = Not Equal?(x=w1716, y=w1722) -> (x != y?=w1717:bool)
              n807 = Not Equal?(x=w1715, y=w1723) -> (x != y?=w1714:bool)
              n808 = Compound Arithmetic op=AND(invert w1715, w1714) -> (w1713:bool)
              n809 = And(x=w1716, y=w1717) -> (x .and. y?=w1721:bool)
              n810 = Select(t="Analyse Plot Space", s=w1721, f=w1719) -> (s? t:f=w1720:string)
            }
            n811 = Compound Arithmetic op=AND(invert w1701, w1700) -> (w1698:bool)
            n812 = And(x=w1705, y=w1704) -> (x .and. y?=w1703:bool)
            n813 = Select(t="What is present?", s=w1703, f=w1699) -> (s? t:f=w1706:string)
          }
          frame #1 {
            n814 = case shown="True" w1738 {
              frame False {
              }
              frame True {
                n815 = Open VI Reference(vi path="Results_Space_Analysis.vi" ("VI path")) -> (vi reference=w1745:refnum<vi>, error out=w1744:errorcluster)  [unwired: 1 in, 4 out]
                n816 = property class="VI"(reference=w1745, error in=w1744, "Front Panel Window:Open"=FALSE) -> (reference out=w1743:refnum<vi>, error out=w1742:errorcluster)
                n817 = Close Reference(reference=w1743, error in (no error)=w1742) -> ()  [unwired: 1 out]
              }
            }
            n818 = case shown="True" w1739 {
              frame False {
              }
              frame True {
                n819 = Open VI Reference(vi path="Plot_Space_Analysis.vi" ("VI path")) -> (vi reference=w1751:refnum<vi>, error out=w1750:errorcluster)  [unwired: 1 in, 4 out]
                n820 = property class="VI"(reference=w1751, error in=w1750, "Front Panel Window:Open"=FALSE) -> (reference out=w1749:refnum<vi>, error out=w1748:errorcluster)
                n821 = Close Reference(reference=w1749, error in (no error)=w1748) -> ()  [unwired: 1 out]
              }
            }
          }
        }
      }
      frame "Check modification dates?" {
        n822 = while {
          shift-right: [w1771] -> _
          shift-left: _ -> [w1769]
          tunnel: [w1768] -> w1760
          stop <- FALSE continue-if-true
          n823 = Get Date/Time In Seconds() -> (seconds since 1Jan1904=w1766:timestamp)
          n824 = To Double Precision Float(number=w1766) -> (double precision float=w1770:dbl)
          n825 = Subtract(x=w1770, y=w1769) -> (x-y=w1774:dbl)
          n826 = Greater?(x=w1774, y=200.0) -> (0:w1772:bool)
          n827 = case shown="True" w1772 {
            tunnel: [w1776 w1779] -> w1771
            tunnel: w1770 -> [_ w1779]
            tunnel: w1769 -> [w1776 _]
            tunnel: [FALSE w1777] -> w1768
            frame False {
            }
            frame True {
              n828 = global read "Results_plotter_Global.vi" "First Loop"() -> (w1778:bool)
              n829 = Not(x=w1778) -> (.not. x?=w1777:bool)
            }
          }
        }
        n830 = Equal?(x="Tab Control", y=enum32{"Load ", "Plot ", "Save ", "Cursor"}."Cursor" ("Tab Control")) -> (x = y?=w1756:bool)
        n831 = global write "Results_plotter_Global.vi" "First Loop"(FALSE) -> ()
        n832 = Select(t="Read Cursor", s=w1756, f="Ordinate Selector Type") -> (s? t:f=w1754:string)
        n833 = Select(t="Files Modified?", s=w1760, f=w1754) -> (s? t:f=w1759:string)
      }
      frame "Files Modified?" {
        n834 = local read "No Of Rows"() -> (w1783:i32)
        n835 = Less?(x=w1783, y=w1782) -> (x < y?=w1780:bool)
        n836 = case shown="False" w1780 {
          tunnel: [w1789 w1795] -> w1784
          tunnel: "Ordinate Selector Type" -> [w1789 w1790]
          frame False {
          }
          frame True {
            n837 = local read "Result files to read"() -> (w1794:path[])
            n838 = for {
              tunnel: w1794 -> [w1798] mode=indexing
              tunnel: [w1796] -> w1793 mode=indexing
              n839 = call "File_Modified_Since_Check.vi"("Pathname"=w1798, "Just Modified?"=TRUE) -> ("Modified?"=w1796:bool)
            }
            n840 = Or Array Elements(Boolean array=w1793) -> (logical OR=w1792:bool)
            n841 = Select(t="Initialise", s=w1792, f=w1790) -> (s? t:f=w1795:string)
          }
        }
      }
      frame "Read Cursor" {
        n842 = stacked-sequence {
          seq-local: [w1804 _] -> [_ w1839]
          tunnel: ["Ordinate Selector Type" _] -> w1802
          tunnel: [TRUE _] -> w1801
          tunnel: w1800 -> [_ w1838]
          tunnel: w1799 -> [_ w1837]
          frame #0 {
            n843 = property on="XY Plot" class="XYGraph (strict)"() -> ("Cursor.Cursor Position:Cursor X"=w1806:dbl, "Cursor.Cursor Position:Cursor Y"=w1805:dbl)  [unwired: 2 in, 2 out]
            n844 = local read "Transpose"() -> (w1819:bool)
            n845 = global read "Results_plotter_Global.vi" "Plot Index values"() -> (w1812:dbl[][])
            n846 = Index Array(array=w1812, index (row)=1) -> (element=w1810:dbl[])  [unwired: 1 in]
            n847 = Index Array(array=w1812, index (row)=2) -> (element=w1809:dbl[])  [unwired: 1 in]
            n848 = Index Array(array=w1812, index (row)=0) -> (element=w1811:dbl[])  [unwired: 1 in]
            n849 = case shown="True" w1819 {
              tunnel: [w1823 w1825] -> w1818
              tunnel: w1806 -> [w1823 w1824]
              tunnel: [w1822 w1824] -> w1817
              tunnel: w1805 -> [w1822 w1825]
              frame False {
              }
              frame True {
              }
            }
            n850 = for {
              tunnel: w1818 -> [w1834]
              tunnel: w1817 -> [w1833]
              tunnel: [w1828] -> w1816 mode=indexing
              tunnel: w1811 -> [w1827] mode=indexing
              tunnel: w1810 -> [w1826] mode=indexing
              n851 = Subtract(x=w1834, y=w1827) -> (x-y=w1832:dbl)
              n852 = Subtract(x=w1833, y=w1826) -> (x-y=w1831:dbl)
              n853 = Multiply(x=w1832, y=w1832) -> (x*y=w1829:dbl)
              n854 = Multiply(x=w1831, y=w1831) -> (x*y=w1830:dbl)
              n855 = Add(x=w1829, y=w1830) -> (x+y=w1828:dbl)
            }
            n856 = Array Max & Min(array=w1816) -> (min index (indices)=w1808:i32)  [unwired: 3 out]
            n857 = Index Array(array=w1809, index=w1808) -> (element=w1807:dbl)
            n858 = To Long Integer(number=w1807) -> (32bit integer=w1804:i32)
            "Cursor index" <- w1804
          }
          frame #1 {
            n859 = Index Array(array=w1838, index (row)=w1839) -> (element=w1836:string[])  [unwired: 1 in]
            n860 = for {
              tunnel: w1837 -> [w1847] mode=indexing
              tunnel: w1836 -> [w1840] mode=indexing
              tunnel: [w1846] -> w1835 mode=indexing
              n861 = while {
                shift-right: [w1859] -> _
                shift-left: w1840 -> [w1860]
                tunnel: [w1856] -> w1844
                tunnel: [w1855] -> w1842 mode=indexing
                i -> [w1856]
                stop <- w1857 continue-if-true
                n862 = Match Pattern(string=w1860, regular expression=":") -> (before substring=w1855:string, after substring=w1859:string, offset past match=w1858:i32)  [unwired: 2 out]
                n863 = Greater Than 0?(x=w1858) -> (x > 0?=w1857:bool)
              }
              n864 = Greater?(x=w1844, y=2) -> (0:w1843:bool)
              n865 = Reverse 1D Array(array=w1842) -> (reversed array=w1841:string[])
              n866 = case shown="True" w1843 {
                tunnel: w1847 -> [w1850 w1854]
                tunnel: [w1848 w1853] -> w1846
                tunnel: w1841 -> [_ w1852]
                tunnel: w1840 -> [w1849 w1851]
                frame False {
                  n867 = Build Array(w1850, w1849) -> (w1848:string[])
                }
                frame True {
                  n868 = Build Array (concatenate)(w1854, w1852, w1851) -> (w1853:string[])
                }
              }
            }
            "Table" <- w1835
          }
        }
      }
      frame "Process Cursor Point" {
        n869 = stacked-sequence {
          tunnel: [w1883] -> w1866
          tunnel: [TRUE] -> w1865
          tunnel: w1864 -> [_]
          tunnel: w1863 -> [_]
          tunnel: w1862 -> [w1884]
          frame #0 {
            w1875 = FALSE  # Add Extra Channels?
            w1876 = FALSE  # Read Channel Names only
            n870 = local read "Kill Point"() -> (w1885:bool)
            n871 = local read "Cursor index"() -> (w1891:i32)
            n872 = global read "Results_plotter_Global.vi" "Row Reference"() -> (w1892:i32[][])
            n873 = Index Array(array=w1892, index (row)=w1891) -> (element=w1886:i32[])  [unwired: 1 in]
            n874 = local read "Result files to read"() -> (w1890:path[])
            n875 = Index Array(array=w1886, index=0) -> (element=w1889:i32)
            n876 = Index Array(array=w1886, index=1) -> (element=w1870:i32)
            n877 = Index Array(array=w1890, index=w1889) -> (element=w1874:path)
            n878 = global read "Constants_global.vi" "Run VI Folder"() -> (w1879:path)
            n879 = Strip Path(path=w1879) -> (stripped path=w1880:path)  [unwired: 1 out]
            n880 = Build Path(base path=w1880, name or relative path="Data_plotting_vis") -> (appended path=w1881:path)
            n881 = Build Path(base path=w1881, name or relative path="RD_Files.tpt") -> (appended path=w1877:path)
            n882 = call "Read_Data_file.vi"("Results file"=w1874, "Read Channel Names only"=w1876, "Add Extra Channels?"=w1875, "Template File"=w1877) -> ("Channel Values Out"=w1871:string[][])  [unwired: 1 in, 14 out]
            n883 = Index Array(array=w1871, index (col)=0 ("index (row)")) -> (element=w1873:string[])  [unwired: 1 in]
            n884 = Index Array(array=w1873, index=w1870) -> (element=w1869:string)
            n885 = call "String_to_Pathname.vi"("Input String"=w1869) -> ("path"=w1868:path)
            n886 = case shown="False" w1885 {
              tunnel: w1874 -> [_ w1904]
              tunnel: w1870 -> [_ w1900]
              tunnel: w1884 -> [_ w1907]
              tunnel: ["What to do next?" ("t") w1906] -> w1883
              tunnel: w1868 -> [w1894 w1898]
              frame False {
                n887 = call "Post_Process_Measurement.vi"("Raw data file"=w1894) -> ()  [unwired: 1 out]
                n888 = local write "Process Point"(FALSE ("Kill Point")) -> ()
              }
              frame True {
                n889 = Strip Path(path=w1904) -> (name=w1899:string)  [unwired: 1 out]
                n890 = Strip Path(path=w1898) -> (name=w1897:string)  [unwired: 1 out]
                n891 = local read "No Of Rows"() -> (w1909:i32)
                n892 = Format Into String(format string="Are you sure you want to remove the row in the results file \"%s\" generated from the raw data filename \"%s\"?", w1899, w1897) -> (resulting string=w1902:string)  [unwired: 2 in, 1 out]
                n893 = Less?(x=w1909, y=w1907) -> (x < y?=w1908:bool)
                n894 = Two Button Dialog(message=w1902) -> (T button?=w1901:bool)  [unwired: 2 out]
                n895 = case shown="False" w1908 {
                  tunnel: ["Create Selectors" "Initialise" ("t")] -> w1906
                  frame False {
                  }
                  frame True {
                  }
                }
                n896 = case shown="True" w1901 {
                  tunnel: w1904 -> [_ w1911]
                  tunnel: w1900 -> [_ w1910]
                  frame False {
                  }
                  frame True {
                    n897 = Build Array(w1910) -> (w1912:i32[])
                    n898 = call "Delete_unwanted_rows.vi"("Selected Rows"=w1912, "Filename"=w1911) -> ()  [unwired: 1 out]
                  }
                }
                n899 = local write "Kill Point"(FALSE ("Kill Point")) -> ()
              }
            }
          }
        }
      }
      frame "Edit template file" {
        n900 = stacked-sequence {
          frame #0 {
            n901 = local read "Template"() -> (w1921:path)
            n902 = call "Valid_Path.vi"("Filename"=w1921) -> ("Valid Path?"=w1920:bool)
            n903 = case shown="False" w1920 {
              tunnel: [T8."Edit Existing Template File" ("Mode") T8."Create New Template File" ("Mode")] -> w1924
              frame True {
              }
              frame False {
              }
            }
            n904 = local read "Results file"() -> (w1923:path)
            n905 = call "Edit_Template_File.vi"("Mode"=w1924, "Template Filename"=w1921, "Data Filename"=w1923) -> ("Template Filename Out"=w1922:path)  [unwired: 12 out]
            n906 = local write "Template"(w1922) -> ()
          }
          frame #1 {
            n907 = local read "Job Directory"() -> (w1927:path)
            n908 = Path To String(path=w1927) -> (string=w1930:string)
            n909 = call "Read_Write_Template.vi"("Mode"=Global_mode."Write Global to File", "Single Value In"=w1930, "Data type"="Log Folder Name" ("Variable name")) -> ()  [unwired: 5 in, 8 out]
            n910 = local write "Edit Template File"(FALSE ("Edit Template File")) -> ()
            n911 = Current VI's Path() -> (path=w1933:path)
            n912 = call "Open_Close_Front_Panel.ph.vi"("Front Panel Window:Open"=TRUE, "VI path"=w1933) -> ()  [unwired: 2 out]
          }
        }
      }
      frame "Save Plot Data" {
        n913 = global read "Results_plotter_Global.vi" "XY Graph Cluster"() -> (w1934:cluster{dbl[], dbl[]}[])
        n914 = local read "Tolerances"() -> (w1941:dbl[])
        n915 = local read "Absisca"() -> (w1940:u16)
        n916 = local read "Transpose"() -> (w1939:bool)
        n917 = local read "Multi Ordinate"() -> (w1938:i32[])
        n918 = global read "Results_plotter_Global.vi" "Precision"() -> (w1935:string[])
        n919 = stacked-sequence {
          seq-local: [w1952 _ _ _ _ _ _ _ _] -> [_ w1977 _ w2015 _ _ _ _ _]
          seq-local: [_ w1973 _ _ _ _ _ _ _] -> [_ _ _ _ _ _ _ w2137 _]
          seq-local: [_ _ _ _ _ w2067 _ _ _] -> [_ _ _ _ _ _ _ w2136 _]
          seq-local: [_ _ _ _ _ w2069 _ _ _] -> [_ _ _ _ _ _ w2105 _ _]
          seq-local: [_ _ _ w2013 _ _ _ _ _] -> [_ _ _ _ _ _ w2106 _ _]
          seq-local: [_ _ _ _ w2036 _ _ _ _] -> [_ _ _ _ _ w2062 _ _ _]
          seq-local: [w1949 _ _ _ _ _ _ _ _] -> [_ _ _ _ _ _ _ _ w2142]
          seq-local: [w1948 _ _ _ _ _ _ _ _] -> [_ w1965 _ _ _ _ _ _ _]
          seq-local: [_ _ w1994 _ _ _ _ _ _] -> [_ _ _ w2014 _ _ w2107 _ _]
          seq-local: [_ _ _ _ _ _ w2103 _ _] -> [_ _ _ _ _ _ _ w2134 _]
          tunnel: [_ _ _ _ _ _ _ _ TRUE] -> w1947
          tunnel: [_ _ _ _ _ _ _ _ w2140] -> w1946
          tunnel: w1944 -> [_ _ _ _ _ w2065 _ _ _]
          tunnel: w1945 -> [_ w1970 _ _ _ w2068 _ _ _]
          tunnel: [_ _ _ _ _ w2068 _ _ _] -> w1943
          tunnel: [_ _ _ _ _ w2065 _ _ _] -> w1942
          tunnel: w1941 -> [w1954 _ _ _ w2041 w2066 _ _ _]
          tunnel: w1934 -> [w1953 _ _ w2017 _ _ _ _ _]
          tunnel: w1940 -> [w1951 w1987 _ _ w2043 _ _ _ _]
          tunnel: w1939 -> [w1950 _ _ w2016 _ _ _ _ _]
          tunnel: w1938 -> [_ _ _ _ w2040 _ _ _ _]
          tunnel: [_ _ _ w2011 _ _ _ _ _] -> w1937
          tunnel: w1936 -> [_ _ w1997 w2011 _ _ _ _ _]
          tunnel: w1935 -> [_ _ _ w2010 _ w2061 _ _ _]
          frame #0 {
            n920 = local read "Save Surface Fit"() -> (w1949:bool)
            n921 = Not(x=w1950) -> (.not. x?=w1957:bool)
            n922 = for {
              tunnel: w1953 -> [w1964] mode=indexing
              tunnel: w1957 -> [w1961]
              shift-right: [w1959] -> w1955
              shift-left: dbl[] [] -> [w1960]
              n923 = Unbundle(w1964) -> (w1963:dbl[], w1962:dbl[])
              n924 = Select(t=w1963, s=w1961, f=w1962) -> (s? t:f=w1958:dbl[])
              n925 = Build Array (concatenate)(w1960, w1958) -> (w1959:dbl[])
            }
            n926 = Index Array(array=w1954, index=w1951) -> (element=w1948:dbl)
            n927 = call "Numeric_bins.vi"("Values"=w1955, "Tolerance"=w1948) -> ("Bin Centres"=w1952:dbl[])  [unwired: 2 out]
          }
          frame #1 {
            n928 = Index Array(array=w1970, index=w1987) -> (element=w1990:string)
            n929 = Match Pattern(string=w1990, regular expression=":") -> (before substring=w1989:string, after substring=w1988:string)  [unwired: 3 out]
            n930 = Concatenate Strings(w1989, " ", w1988, " =:" ("regular expression")) -> (w1972:string)
            n931 = Greater?(x=w1965, y=0.4) -> (0:w1985:bool)
            n932 = Greater?(x=w1965, y=0.09) -> (0:w1980:bool)
            n933 = call <vilib>:"Trim Whitespace.vi"("string"=w1972) -> ("trimmed string"=w1971:string)  [unwired: 1 in]
            n934 = Select(t=i16 0 ("precision (6)"), s=w1985, f=i16 2 ("precision (6)")) -> (s? t:f=w1981:i16)
            n935 = Select(t=w1981, s=w1980, f=i16 3) -> (s? t:f=w1978:i16)
            n936 = Number To Fractional String(number=w1977, precision (6)=w1978) -> (F-format string=w1976:string[])  [unwired: 2 out]
            n937 = for {
              tunnel: w1971 -> [w1993]
              tunnel: w1976 -> [w1991] mode=indexing
              tunnel: [w1992] -> w1975 mode=indexing
              n938 = Concatenate Strings(w1993, w1991) -> (w1992:string)
            }
            n939 = Build Array (concatenate)("Plot:Legend:" ("Input Element"), w1975, "End of:Plot Series:" ("Input Element")) -> (w1973:string[])
          }
          frame #2 {
            n940 = local read "Multi Ordinate?"() -> (w1996:bool)
            n941 = global read "Results_plotter_Global.vi" "Legend"() -> (w1995:string[])
            n942 = case shown="False" w1996 {
              tunnel: w1997 -> [w2001 _]
              tunnel: [w1998 w2009] -> w1994
              tunnel: w1995 -> [w2000 w2009]
              frame False {
                n943 = local read "Multi Ordinate"() -> (w2004:i32[])
                n944 = Index Array(array=w2004, index=0 ("Index")) -> (element=w2002:i32)
                n945 = Index Array(array=w2001, index=w2002) -> (element=w1999:string)
                n946 = for {
                  tunnel: w2000 -> [w2008] mode=indexing
                  tunnel: w1999 -> [w2007]
                  tunnel: [w2005] -> w1998 mode=indexing
                  n947 = Format Into String(format string="; %s", initial string=w2007, w2008) -> (resulting string=w2005:string)  [unwired: 1 in, 1 out]
                }
              }
              frame True {
              }
            }
          }
          frame #3 {
            n948 = call "Grid_Data.vi"("Transpose"=w2016, "XY Graph"=w2017, "Bin Centres"=w2015) -> ("Grided data"=w2012:dbl[][])  [unwired: 1 out]
            n949 = for {
              tunnel: w2014 -> [w2024] mode=indexing
              tunnel: [w2026] -> w2013 mode=indexing
              tunnel: w2012 -> [w2025] mode=indexing
              tunnel: w2011 -> [w2020]
              tunnel: w2010 -> [w2019]
              n950 = Match Pattern(string=w2024, regular expression=";") -> (before substring=w2021:string)  [unwired: 4 out]
              n951 = Search 1D Array(1D array=w2020, element=w2021) -> (index of element=w2022:i32)  [unwired: 1 out]
              n952 = Index Array(array=w2019, index=w2022) -> (element=w2018:string)
              n953 = for {
                tunnel: w2018 -> [w2031]
                tunnel: [w2030] -> w2027 mode=indexing
                tunnel: w2025 -> [w2028] mode=indexing
                n954 = Not A Number/Path/Refnum?(number/path/refnum=w2028) -> (NaN/Path/Refnum?=w2029:bool)
                n955 = case shown="True" w2029 {
                  tunnel: w2031 -> [w2034 _]
                  tunnel: [w2033 ""] -> w2030
                  tunnel: w2028 -> [w2032 _]
                  frame False {
                    n956 = call "Number_2_string.vi"("precision"=w2034, "number"=w2032) -> ("String"=w2033:string)
                  }
                  frame True {
                  }
                }
              }
              n957 = Build Array (concatenate)(w2024, w2027) -> (w2026:string[])
            }
          }
          frame #4 {
            n958 = Index Array(array=w2040, index=0 ("Index")) -> (element=w2038:i32)
            n959 = global read "Results_plotter_Global.vi" "Summarise"() -> (w2037:string[])
            n960 = for {
              shift-right: [w2050] -> w2036
              shift-left: i32[] [] -> [w2051]
              tunnel: w2043 -> [w2056]
              tunnel: w2038 -> [w2055]
              tunnel: w2041 -> [w2048] mode=indexing
              tunnel: w2037 -> [w2046] mode=indexing
              i -> [w2049]
              n961 = Equal?(x=w2055, y=w2049) -> (x = y?=w2054:bool)
              n962 = Not A Number/Path/Refnum?(number/path/refnum=w2048) -> (NaN/Path/Refnum?=w2047:bool)
              n963 = Equal?(x=w2056, y=w2049) -> (x = y?=w2053:bool)
              n964 = Equal?(x="FALSE", y=w2046) -> (x = y?=w2044:bool)
              n965 = Compound Arithmetic op=OR(w2053, w2054, w2047, w2044) -> (w2052:bool)
              n966 = case shown="False" w2052 {
                tunnel: w2051 -> [w2059 w2060]
                tunnel: [w2058 w2060] -> w2050
                tunnel: w2049 -> [w2057 _]
                frame False {
                  n967 = Build Array (concatenate)(w2059, w2057) -> (w2058:i32[])
                }
                frame True {
                }
              }
            }
          }
          frame #5 {
            n968 = local read "Plotted Series"() -> (w2064:bool[][])
            n969 = for {
              tunnel: w2066 -> [w2080]
              tunnel: [w2079] -> w2069 mode=indexing
              tunnel: w2062 -> [w2078]
              tunnel: w2065 -> [w2077]
              tunnel: w2064 -> [w2076] mode=indexing
              tunnel: i32[] [] -> [w2074]
              tunnel: w2061 -> [w2073]
              n970 = for {
                shift-right: [w2082] -> w2075
                shift-left: w2074 -> [w2083]
                tunnel: w2076 -> [w2081] mode=indexing
                i -> [w2084]
                n971 = case shown="True" w2081 {
                  tunnel: w2084 -> [_ w2088]
                  tunnel: w2083 -> [w2085 w2087]
                  tunnel: [w2085 w2086] -> w2082
                  frame False {
                  }
                  frame True {
                    n972 = Build Array (concatenate)(w2087, w2088) -> (w2086:i32[])
                  }
                }
              }
              n973 = for {
                tunnel: w2080 -> [w2096]
                tunnel: [w2097] -> w2079 mode=indexing
                tunnel: w2078 -> [w2091] mode=indexing
                tunnel: w2077 -> [w2094]
                tunnel: w2075 -> [w2093]
                tunnel: w2073 -> [w2090]
                n974 = for {
                  tunnel: w2093 -> [w2102] mode=indexing
                  tunnel: [w2101] -> w2098 mode=indexing
                  tunnel: w2091 -> [w2100]
                  tunnel: w2094 -> [w2099]
                  n975 = Index Array(array=w2099, index (row)=w2102, index (col)=w2100) -> (element=w2101:string)
                }
                n976 = Index Array(array=w2090, index=w2091) -> (element=w2092:string)
                n977 = Index Array(array=w2096, index=w2091) -> (element=w2095:dbl)
                n978 = call "Value_Occurence_Analysis.vi"("Average Numeric Values?"=FALSE, "Tolerance"=w2095, "Precision (3)"=w2092, "String Array"=w2098) -> ("Output String"=w2097:string)  [unwired: 2 out]
              }
            }
            n979 = for {
              tunnel: w2062 -> [w2072] mode=indexing
              tunnel: w2068 -> [w2071]
              tunnel: [w2070] -> w2067 mode=indexing
              n980 = Index Array(array=w2071, index=w2072) -> (element=w2070:string)
            }
          }
          frame #6 {
            n981 = for {
              shift-right: [w2120] -> w2103
              shift-left: string[][] [] -> [w2121]
              shift-right: [w2116] -> _
              shift-left: _ -> [w2117]
              tunnel: w2107 -> [w2118] mode=indexing
              tunnel: w2106 -> [w2110] mode=indexing
              tunnel: w2105 -> [w2109] mode=indexing
              i -> [w2115]
              n982 = Greater Than 0?(x=w2115) -> (x > 0?=w2114:bool)
              n983 = Match Pattern(string=w2118, regular expression="; ") -> (before substring=w2116:string)  [unwired: 4 out]
              n984 = Equal?(x=w2117, y=w2116) -> (x = y?=w2113:bool)
              n985 = Build Array (concatenate)(w2110, "", w2109) -> (w2108:string[])
              n986 = Compound Arithmetic op=AND(w2114, invert w2113) -> (w2112:bool)
              n987 = case shown="True" w2112 {
                tunnel: w2121 -> [w2125 w2128]
                tunnel: [w2124 w2127] -> w2120
                tunnel: w2108 -> [w2123 w2126]
                frame True {
                  n988 = Build Array (concatenate)(w2125, string[] [] ("array"), w2123) -> (w2124:string[][])
                }
                frame False {
                  n989 = Build Array (concatenate)(w2128, w2126) -> (w2127:string[][])
                }
              }
            }
          }
          frame #7 {
            w2133 = TRUE  # Simple Save?
            n990 = Build Array (concatenate)(w2137, w2136) -> (w2135:string[])
            n991 = local read "Header"() -> (w2130:string)
            n992 = call "Write_output_file.vi"("Output filename"="Output Filename", "Header"=w2130, "Channel Names"=w2135, "Data"=w2134, "Simple Save?"=w2133, "Summarise mode"=T9."No data summary") -> ("Output filename Out"=w2131:path)  [unwired: 6 in, 3 out]
            n993 = local write "Output Filename"(w2131) -> ()
          }
          frame #8 {
            n994 = local write "Save Plot data"(FALSE ("Save Plot data")) -> ()
            n995 = local write "Header"("") -> ()
            n996 = Select(t="Save Surface Fit data", s=w2142, f="Create Selectors") -> (s? t:f=w2140:string)
          }
        }
      }
      frame "What type of row averaging?" {
        n997 = Two Button Dialog(message="Do you want to Combine rows with identical positions together?", 1:"Just average series" ("F button name (\"Cancel\")"), 2:"Combine rows" ("T button name (\"OK\")")) -> (T button?=w2148:bool)
        n998 = Select(t="Combine rows" ("T button name (\"OK\")"), s=w2148, f="Average Rows together") -> (s? t:f=w2145:string)
      }
      frame "Combine rows" {
        w2158 = TRUE  # Show panel ?
        n999 = local read "Output Filename"() -> (w2157:path)
        n1000 = call "Combined_file_Panel.vi"("Show panel ?"=w2158, "Output filename"=w2157) -> ("Only Plotted data?"=w2159:bool, "Include Empty Rows? Out"=w2160:bool, "Give Audit Channels Out"=w2161:bool, "Output filename Out"=w2156:path)  [unwired: 5 out]
        n1001 = case shown="False" w2159 {
          tunnel: w2163 -> [w2172 w2175]
          tunnel: [w2172 w2173] -> w2162
          frame False {
          }
          frame True {
            n1002 = global read "Results_plotter_Global.vi" "Plot Index values"() -> (w2177:dbl[][])
            n1003 = Index Array(array=w2177, index (row)=2) -> (element=w2174:dbl[])  [unwired: 1 in]
            n1004 = for {
              tunnel: w2175 -> [w2180]
              tunnel: w2174 -> [w2179] mode=indexing
              tunnel: [w2178] -> w2173 mode=indexing
              n1005 = Index Array(array=w2180, index (row)=w2179) -> (element=w2178:string[])  [unwired: 1 in]
            }
          }
        }
        n1006 = local write "Save Averaged rows"(FALSE ("Save Plot data")) -> ()
        n1007 = local read "X Ch Name"() -> (w2167:u16)
        n1008 = local read "Y Ch Name"() -> (w2168:u16)
        n1009 = local read "Z Ch Name"() -> (w2169:u16)
        n1010 = call "Find_Rows_to_Combine.vi"("Include Empty Rows?"=w2160, "file path (dialog if empty)"=w2156, "Give Audit Channels"=w2161, "Full Channel Names"=w2166, "Data"=w2162, "Z Column Index"=w2169, "Y Column Index"=w2168, "X Column Index"=w2167) -> ()  [unwired: 4 out]
        n1011 = local write "Output Filename"(w2156) -> ()
      }
      frame "Average Rows together" {
        n1012 = global read "Results_plotter_Global.vi" "XY Graph Cluster"() -> (w2182:cluster{dbl[], dbl[]}[])
        n1013 = local read "Tolerances"() -> (w2188:dbl[])
        n1014 = local read "Absisca"() -> (w2187:u16)
        n1015 = local read "Transpose"() -> (w2186:bool)
        n1016 = global read "Results_plotter_Global.vi" "Precision"() -> (w2184:string[])
        n1017 = global read "Results_plotter_Global.vi" "Summarise"() -> (w2183:string[])
        n1018 = stacked-sequence {
          seq-local: [w2200 _ _ _ _] -> [_ w2217 _ _ _]
          seq-local: [_ w2220 _ _ _] -> [_ _ _ w2302 _]
          seq-local: [w2196 _ _ _ _] -> [_ w2218 _ _ _]
          seq-local: [_ _ w2280 _ _] -> [_ _ _ w2296 _]
          tunnel: [_ _ _ _ TRUE] -> w2194
          tunnel: [_ _ _ _ "Create Selectors"] -> w2193
          tunnel: w2191 -> [_ w2223 _ _ w2305]
          tunnel: w2192 -> [_ _ w2281 _ w2304]
          tunnel: [_ _ _ _ w2304] -> w2190
          tunnel: [_ _ _ _ w2305] -> w2189
          tunnel: w2188 -> [w2202 w2221 _ _ _]
          tunnel: w2182 -> [w2201 _ _ _ _]
          tunnel: w2187 -> [w2199 _ _ _ _]
          tunnel: w2186 -> [w2198 _ _ _ _]
          tunnel: w2185 -> [w2195 _ _ _ _]
          tunnel: w2184 -> [_ w2222 _ _ _]
          tunnel: w2183 -> [_ w2219 w2282 _ _]
          tunnel: [w2195 _ _ _ _] -> w2181
          frame #0 {
            n1019 = Not(x=w2198) -> (.not. x?=w2205:bool)
            n1020 = for {
              tunnel: w2201 -> [w2212] mode=indexing
              tunnel: w2205 -> [w2209]
              shift-right: [w2207] -> w2203
              shift-left: dbl[] [] -> [w2208]
              n1021 = Unbundle(w2212) -> (w2211:dbl[], w2210:dbl[])
              n1022 = Select(t=w2211, s=w2209, f=w2210) -> (s? t:f=w2206:dbl[])
              n1023 = Build Array (concatenate)(w2208, w2206) -> (w2207:dbl[])
            }
            n1024 = Index Array(array=w2202, index=w2199) -> (element=w2197:dbl)
            n1025 = call "Numeric_bins.vi"("Values"=w2203, "Tolerance"=w2197) -> ("Bin Centres"=w2200:dbl[], "Bin Index"=w2196:i32[])  [unwired: 1 out]
          }
          frame #1 {
            n1026 = Array Size(array=w2217) -> (size(s)=w2216:i32)
            n1027 = global read "Results_plotter_Global.vi" "Plot Index values"() -> (w2214:dbl[][])
            n1028 = Index Array(array=w2214, index (row)=2) -> (element=w2213:dbl[])  [unwired: 1 in]
            n1029 = for {
              N: w2216 -> [_]
              tunnel: w2223 -> [w2233]
              tunnel: w2222 -> [w2232]
              tunnel: w2221 -> [w2231]
              tunnel: [w2224] -> w2220 mode=indexing
              tunnel: w2219 -> [w2230]
              tunnel: w2218 -> [w2228]
              tunnel: w2213 -> [w2227]
              i -> [w2229]
              n1030 = stacked-sequence {
                seq-local: [w2237 _] -> [_ w2256]
                tunnel: w2233 -> [_ w2257]
                tunnel: w2232 -> [_ w2255]
                tunnel: w2231 -> [_ w2254]
                tunnel: w2230 -> [_ w2253]
                tunnel: w2229 -> [w2236 _]
                tunnel: w2228 -> [w2235 _]
                tunnel: w2227 -> [w2234 _]
                tunnel: [_ w2251] -> w2226
                tunnel: [_ w2250] -> w2225
                frame #0 {
                  n1031 = for {
                    shift-right: [w2243] -> w2237
                    shift-left: i32[] [] -> [w2244]
                    tunnel: w2236 -> [w2242]
                    tunnel: w2235 -> [w2241] mode=indexing
                    tunnel: w2234 -> [w2239] mode=indexing
                    n1032 = Equal?(x=w2241, y=w2242) -> (x = y?=w2240:bool)
                    n1033 = case shown="False" w2240 {
                      tunnel: w2244 -> [w2245 w2248]
                      tunnel: [w2245 w2249] -> w2243
                      tunnel: w2239 -> [_ w2246]
                      frame False {
                      }
                      frame True {
                        n1034 = To Long Integer(number=w2246) -> (32bit integer=w2247:i32)
                        n1035 = Build Array (concatenate)(w2248, w2247) -> (w2249:i32[])
                      }
                    }
                  }
                }
                frame #1 {
                  n1036 = for {
                    tunnel: w2257 -> [w2271]
                    tunnel: w2256 -> [w2270]
                    tunnel: w2255 -> [w2268] mode=indexing
                    tunnel: w2254 -> [w2267] mode=indexing
                    tunnel: [w2266] -> w2251 mode=indexing
                    tunnel: w2253 -> [w2263] mode=indexing
                    shift-right: [w2258] -> w2250
                    shift-left: string[] [] -> [w2259]
                    i -> [w2265]
                    n1037 = for {
                      tunnel: w2271 -> [w2279]
                      tunnel: w2270 -> [w2278] mode=indexing
                      tunnel: [w2277] -> w2269 mode=indexing
                      tunnel: w2265 -> [w2276]
                      n1038 = Index Array(array=w2279, index (row)=w2278, index (col)=w2276) -> (element=w2277:string)
                    }
                    n1039 = Equal?(x="TRUE", y=w2263) -> (x = y?=w2262:bool)
                    n1040 = Not(x=w2262) -> (.not. x?=w2261:bool)
                    n1041 = call "Value_Occurence_Analysis.vi"("Average Numeric Values?"=w2261, "Tolerance"=w2267, "Precision (3)"=w2268, "String Array"=w2269) -> ("St Dev"=w2260:string, "Output String"=w2266:string)  [unwired: 1 out]
                    n1042 = case shown="False" w2261 {
                      tunnel: w2260 -> [_ w2275]
                      tunnel: w2259 -> [w2272 w2274]
                      tunnel: [w2272 w2273] -> w2258
                      frame False {
                      }
                      frame True {
                        n1043 = Build Array (concatenate)(w2274, w2275) -> (w2273:string[])
                      }
                    }
                  }
                }
              }
              n1044 = Build Array (concatenate)(w2226, w2225) -> (w2224:string[])
            }
          }
          frame #2 {
            n1045 = for {
              tunnel: w2282 -> [w2287] mode=indexing
              shift-right: [w2283] -> w2280
              shift-left: w2281 -> [w2284]
              tunnel: w2281 -> [w2285] mode=indexing
              n1046 = Equal?(x="TRUE", y=w2287) -> (x = y?=w2286:bool)
              n1047 = case shown="False" w2286 {
                tunnel: w2285 -> [w2293 _]
                tunnel: w2284 -> [w2290 w2294]
                tunnel: [w2289 w2294] -> w2283
                frame False {
                  n1048 = Concatenate Strings(w2293, "St Dev") -> (w2291:string)
                  n1049 = Build Array (concatenate)(w2290, w2291) -> (w2289:string[])
                }
                frame True {
                }
              }
            }
          }
          frame #3 {
            w2299 = FALSE  # Save Plotted rows only?
            w2301 = TRUE  # Simple Save?
            n1050 = local read "Output Filename"() -> (w2297:path)
            n1051 = local read "Header"() -> (w2298:string)
            n1052 = local read "Template"() -> (w2300:path)
            n1053 = call "Write_output_file.vi"("Output filename"=w2297, "Header"=w2298, "Template Filename"=w2300, "Channel Names"=w2296, "Data"=w2302, "Simple Save?"=w2301, "Save Plotted rows only?"=w2299, "Summarise mode"=T9."No data summary") -> ("Output filename Out"=w2303:path)  [unwired: 4 in, 3 out]
            n1054 = local write "Output Filename"(w2303) -> ()
          }
          frame #4 {
            n1055 = local write "Save Averaged rows"(FALSE ("Save Plot data")) -> ()
          }
        }
      }
      frame "Save Surface Fit data" {
        n1056 = local read "Transpose"() -> (w2309:bool)
        n1057 = local read "Tolerances"() -> (w2316:dbl[])
        n1058 = local read "Absisca"() -> (w2315:u16)
        n1059 = global read "Results_plotter_Global.vi" "Precision"() -> (w2312:string[])
        n1060 = stacked-sequence {
          seq-local: [w2323 _ _ _ _ _] -> [_ w2342 _ _ _ _]
          seq-local: [_ w2339 _ _ _ _] -> [_ _ _ _ w2426 _]
          seq-local: [_ _ w2365 _ _ _] -> [_ _ _ _ w2445 _]
          seq-local: [w2324 _ _ _ _ _] -> [_ _ w2366 _ _ _]
          seq-local: [_ _ w2361 _ _ _] -> [_ _ _ _ w2429 _]
          seq-local: [_ _ w2360 _ _ _] -> [_ _ _ w2396 _ _]
          seq-local: [_ _ _ w2391 _ _] -> [_ _ _ _ w2427 _]
          tunnel: [_ _ _ _ _ TRUE] -> w2320
          tunnel: [_ _ _ _ _ "Create Selectors"] -> w2319
          tunnel: w2317 -> [_ _ _ _ _ w2451]
          tunnel: w2318 -> [_ w2327 _ _ _ w2452]
          tunnel: w2316 -> [_ w2353 _ _ _ _]
          tunnel: w2315 -> [_ w2354 _ _ _ _]
          tunnel: [_ _ w2371 _ _ _] -> w2314
          tunnel: w2313 -> [_ w2330 w2371 _ _ _]
          tunnel: w2312 -> [_ _ w2367 _ _ _]
          tunnel: [_ _ _ _ _ w2452] -> w2311
          tunnel: [_ _ _ _ _ w2451] -> w2310
          tunnel: w2309 -> [_ _ _ w2390 _ _]
          frame #0 {
            n1061 = global read "Results_plotter_Global.vi" "Raw Interpolation"() -> (w2321:dbl[][])
            n1062 = global read "Results_plotter_Global.vi" "X Values"() -> (w2323:dbl[])
            n1063 = global read "Results_plotter_Global.vi" "Y Values"() -> (w2322:dbl[])
            n1064 = Insert Into Array(array=w2321, index (col)=0 ("disabled index (col)"), new element=w2322) -> (w2324:dbl[][])  [unwired: 1 in]
          }
          frame #1 {
            n1065 = global read "Results_plotter_Global.vi" "Y Axis Name"() -> (w2329:string)
            n1066 = Search 1D Array(1D array=w2330, element=w2329) -> (index of element=w2328:i32)  [unwired: 1 out]
            n1067 = Index Array(array=w2327, index=w2328) -> (element=w2326:string)
            n1068 = Match Pattern(string=w2326, regular expression=":") -> (before substring=w2356:string, after substring=w2355:string)  [unwired: 3 out]
            n1069 = Index Array(array=w2353, index=w2354) -> (element=w2344:dbl)
            n1070 = Concatenate Strings(w2356, " ", w2355, " =:" ("regular expression")) -> (w2338:string)
            n1071 = Greater?(x=w2344, y=0.9) -> (0:w2351:bool)
            n1072 = Greater?(x=w2344, y=0.09) -> (0:w2346:bool)
            n1073 = call <vilib>:"Trim Whitespace.vi"("string"=w2338) -> ("trimmed string"=w2337:string)  [unwired: 1 in]
            n1074 = Select(t=i16 0 ("precision (6)"), s=w2351, f=i16 2 ("precision (6)")) -> (s? t:f=w2347:i16)
            n1075 = Select(t=w2347, s=w2346, f=i16 3) -> (s? t:f=w2343:i16)
            n1076 = Number To Fractional String(number=w2342, precision (6)=w2343) -> (F-format string=w2341:string[])  [unwired: 2 out]
            n1077 = for {
              tunnel: w2337 -> [w2359]
              tunnel: w2341 -> [w2357] mode=indexing
              tunnel: [w2358] -> w2332 mode=indexing
              n1078 = Concatenate Strings(w2359, w2357) -> (w2358:string)
            }
            n1079 = Build Array (concatenate)("Channel:Values:Plotted" ("Input Element"), "Axis:Name:" ("Input Element"), "Axis:Values:" ("Input Element"), w2332) -> (w2339:string[])
          }
          frame #2 {
            n1080 = global read "Results_plotter_Global.vi" "X Axis Name"() -> (w2364:string)
            n1081 = Concatenate Strings(w2364, " =" ("string")) -> (w2362:string)
            n1082 = local read "Multi Ordinate"() -> (w2370:i32[])
            n1083 = Index Array(array=w2370, index=0 ("Index")) -> (element=w2368:i32)
            n1084 = Index Array(array=w2367, index=w2368) -> (element=w2360:string)
            n1085 = Index Array(array=w2371, index=w2368) -> (element=w2361:string)
            n1086 = for {
              tunnel: w2361 -> [w2373]
              tunnel: [w2376] -> w2365 mode=indexing
              tunnel: w2360 -> [w2375]
              tunnel: w2366 -> [w2374] mode=indexing
              tunnel: w2362 -> [w2372]
              n1087 = for {
                tunnel: w2374 -> [w2379] mode=indexing
                tunnel: [w2378] -> w2377 mode=indexing
                tunnel: w2375 -> [w2381]
                n1088 = Not A Number/Path/Refnum?(number/path/refnum=w2379) -> (NaN/Path/Refnum?=w2380:bool)
                n1089 = case shown="False" w2380 {
                  tunnel: w2381 -> [w2384 _]
                  tunnel: w2379 -> [w2383 _]
                  tunnel: [w2382 ""] -> w2378
                  frame False {
                    n1090 = call "Number_2_string.vi"("precision"=w2384, "number"=w2383) -> ("String"=w2382:string)
                  }
                  frame True {
                  }
                }
              }
              n1091 = Build Array (concatenate)(w2373, w2372, w2377) -> (w2376:string[])
            }
          }
          frame #3 {
            w2395 = "\t"
            n1092 = global read "Results_plotter_Global.vi" "Intensity Plot data in rows"() -> (w2397:dbl[][])
            n1093 = global read "Results_plotter_Global.vi" "Value plotted Name"() -> (w2394:string)
            n1094 = global read "Results_plotter_Global.vi" "X Axis Name"() -> (w2388:string)
            n1095 = global read "Results_plotter_Global.vi" "Y Axis Name"() -> (w2387:string)
            n1096 = case shown="False" w2390 {
              tunnel: [w2398 w2401] -> w2389
              tunnel: w2388 -> [w2399 w2401]
              tunnel: w2387 -> [w2398 w2400]
              tunnel: [w2399 w2400] -> w2386
              frame False {
              }
              frame True {
              }
            }
            n1097 = Concatenate Strings(w2389, w2395, w2386, w2395, w2394, "\r") -> (w2392:string)
            n1098 = for {
              tunnel: w2397 -> [w2407] mode=indexing
              tunnel: w2396 -> [w2412]
              shift-right: [w2406] -> w2391
              shift-left: w2392 -> [w2411]
              n1099 = Index Array(array=w2407, index=0) -> (element=w2403:dbl)
              n1100 = Index Array(array=w2407, index=1) -> (element=w2402:dbl)
              n1101 = Index Array(array=w2407, index=2) -> (element=w2405:dbl)
              n1102 = Not A Number/Path/Refnum?(number/path/refnum=w2405) -> (NaN/Path/Refnum?=w2404:bool)
              n1103 = case shown="False" w2404 {
                tunnel: w2412 -> [w2423 _]
                tunnel: w2411 -> [w2422 w2424]
                tunnel: w2405 -> [w2421 _]
                tunnel: [w2420 w2424] -> w2406
                tunnel: w2403 -> [w2419 _]
                tunnel: w2402 -> [w2418 _]
                frame False {
                  w2414 = "\t"
                  n1104 = call "Number_2_string.vi"("number"=w2419) -> ("String"=w2417:string)  [unwired: 1 in]
                  n1105 = call "Number_2_string.vi"("number"=w2418) -> ("String"=w2416:string)  [unwired: 1 in]
                  n1106 = call "Number_2_string.vi"("precision"=w2423, "number"=w2421) -> ("String"=w2415:string)
                  n1107 = Concatenate Strings(w2422, w2417, w2414, w2416, w2414, w2415, "\r") -> (w2420:string)
                }
                frame True {
                }
              }
            }
          }
          frame #4 {
            w2441 = TRUE  # append to file? (new file:F)
            n1108 = global read "Results_plotter_Global.vi" "Surface Integral"() -> (w2440:dbl)
            n1109 = global read "Results_plotter_Global.vi" "Surface Area"() -> (w2439:dbl)
            n1110 = Initialize Array("", 10 ("Dimension Size")) -> (w2450:string[])
            n1111 = Divide(x=w2440, y=w2439) -> (x/y=w2438:dbl)
            n1112 = call "Asterisk_header.vi"("Channel names"=w2450) -> ("Header string"=w2428:string)
            n1113 = call "Value_to_string.vi"("Value"=w2440, "Label for value"="Surface Integral") -> ("Output string"=w2435:string)  [unwired: 1 in]
            n1114 = call "Value_to_string.vi"("Value"=w2439, "Label for value"="Surface Area") -> ("Output string"=w2436:string)  [unwired: 1 in]
            n1115 = call "Value_to_string.vi"("Value"=w2438, "Label for value"="Surface Average") -> ("Output string"=w2434:string)  [unwired: 1 in]
            n1116 = Concatenate Strings(w2436, w2435, w2434) -> (w2431:string)
            n1117 = call "Ch_names_to_rows.vi"("Channel Names"=w2426) -> ("3 Row names"=w2425:string[][])
            n1118 = local read "Output Filename"() -> (w2442:path)
            n1119 = Build Array (concatenate)(w2425, w2445) -> (w2443:string[][])
            n1120 = Array To Spreadsheet String(array=w2443, 3:"%s" ("format string")) -> (spreadsheet string=w2430:string)  [unwired: 1 out]
            n1121 = Format Into String(format string="\n%s\n\n%s\n%s\n\n\nInterpolated Surface of %s\n%s\n%s\n%s\n\n\n%s", w2428, w2427, w2428, w2429, w2428, w2430, w2428, w2431) -> (resulting string=w2433:string)  [unwired: 2 in, 1 out]
            n1122 = call "Write_Characters_To_File.vi"("file path (dialog if empty)"=w2442, "character string"=w2433, "append to file? (new file:F)"=w2441) -> ()  [unwired: 2 in, 4 out]
          }
          frame #5 {
            n1123 = local write "Save Surface Fit"(FALSE ("Save Plot data")) -> ()
          }
        }
      }
      frame "Save Data in Rows" {
        w2467 = TRUE  # Show panel ?
        n1124 = local read "Output Filename"() -> (w2464:path)
        n1125 = local write "Save Data in Rows"(FALSE ("Save All data")) -> ()
        n1126 = call "Output_file_Panel.vi"("Show panel ?"=w2467, "Channel Names"=w2462, "Header"="Header", "Output filename"=w2464) -> ("Save Full Res Data?"=w2459:bool, "Desired Columns"=w2468:i32[], "Header Out"=w2466:string, "Output filename Out"=w2470:path, "Channels to Tabulate in header Out"=w2456:i32[], "Save Plotted rows only?"=w2457:bool, "Summarise mode"=w2465:T9, "Grouping info"=w2458:T14[])
        "Plotted rows only?" <- w2457
        n1127 = case shown="False" w2459 {
          tunnel: w2470 -> [w2486 w2488]
          tunnel: w2468 -> [w2485 _]
          tunnel: w2466 -> [w2484 _]
          tunnel: w2457 -> [w2483 _]
          tunnel: w2465 -> [w2482 _]
          tunnel: w2463 -> [w2481 _]
          tunnel: w2462 -> [w2480 _]
          tunnel: [w2479 w2488] -> w2461
          tunnel: ["Create Selectors" "Is Filename Empty?"] -> w2460
          tunnel: w2458 -> [w2475 _]
          tunnel: w2456 -> [w2474 _]
          frame False {
            w2477 = FALSE  # Simple Save?
            n1128 = local read "Template"() -> (w2478:path)
            n1129 = call "Write_output_file.vi"("Output filename"=w2486, "Header"=w2484, "Template Filename"=w2478, "Channel Names"=w2480, "Data"=w2481, "Desired Columns"=w2485, "Simple Save?"=w2477, "Save Plotted rows only?"=w2483, "Summarise mode"=w2482, "Grouping info"=w2475, "Channels to Tabulate in header"=w2474) -> ("Output filename Out"=w2479:path)  [unwired: 1 in, 3 out]
          }
          frame True {
            "Mode" <- Plotter_Mode."Save file" ("Mode")
          }
        }
        n1130 = local write "Output Filename"(w2461) -> ()
      }
      frame "Is Filename Empty?" {
        n1131 = call "File Dialog"("start path"="Full_Res_Results_Folder", "prompt"="Please select a new or existing folder to save the results files in") -> ("selected path"=w2492:path, "cancelled"=w2490:bool)  [unwired: 5 in, 7 out]
        n1132 = local write "Full_Res_Results_Folder"(w2492) -> ()
        n1133 = case shown="False" w2490 {
          tunnel: ["Full Res file manipulator" ("f") "Create Selectors" ("t")] -> w2494
          frame False {
          }
          frame True {
          }
        }
      }
      frame "Check for overwrite or append" {
        n1134 = local read "Output Filename"() -> (w2508:path)
        n1135 = Format Into String(format string="Do you want to append to the result file\n\"%s\"" ("message"), w2508) -> (resulting string=w2503:string)  [unwired: 2 in, 1 out]
        n1136 = call <vilib>:"Three Button Dialog.vi"("Window Title (\"\")"="Output File Dialog" ("Window Title (\"\")"), "Right Button Text (\"Cancel\")"="Cancel" ("Button 3 Name"), "Center Button Text (\"No\")"="Overwrite" ("F button name (\"Cancel\")"), "Left Button Text (\"Yes\")"="Append" ("T button name (\"OK\")"), "message"=w2503) -> ("Which Button?"=w2502:T11)  [unwired: 6 out]
        n1137 = case shown="\"Center Button\"" w2502 {
          tunnel: w2508 -> [_ w2515 _]
          tunnel: ["Full Res file manipulator" "Full Res file manipulator" "Create Selectors" ("t")] -> w2501
          frame "Left Button" {
          }
          frame "Center Button" {
            n1138 = call "Delete_with_Check.vi"("FilePath"=w2515) -> ()  [unwired: 1 out]
          }
          frame "Right Button", Default {
          }
        }
      }
      frame "Create Plot summary" {
        w2530 = TRUE  # Summarise All
        n1139 = global read "Results_plotter_Global.vi" "Plot Index values"() -> (w2533:dbl[][])
        n1140 = local read "Intensity Plot?"() -> (w2529:bool)
        n1141 = global read "Results_plotter_Global.vi" "Row Reference"() -> (w2525:i32[][])
        n1142 = Index Array(array=w2525, index (col)=0 ("disabled index (col)")) -> (element=w2524:i32[])  [unwired: 1 in]
        n1143 = Index Array(array=w2533, index (row)=2) -> (element=w2535:dbl[])  [unwired: 1 in]
        n1144 = Select(t="Save Intensity plot as jpg", s=w2529, f="Create summary per series") -> (s? t:f=w2520:string)
        n1145 = To Long Integer(number=w2535) -> (32bit integer=w2532:i32[])
        n1146 = for {
          tunnel: w2540 -> [w2553]
          tunnel: [w2552] -> w2531 mode=indexing
          tunnel: w2532 -> [w2550] mode=indexing
          tunnel: w2524 -> [w2551]
          shift-right: [w2547] -> w2522
          shift-left: i32[] [] -> [w2548]
          n1147 = Index Array(array=w2551, index=w2550) -> (element=w2546:i32)
          n1148 = Search 1D Array(1D array=w2548, element=w2546) -> (index of element=w2549:i32)  [unwired: 1 out]
          n1149 = Index Array(array=w2553, index (row)=w2550) -> (element=w2552:string[])  [unwired: 1 in]
          n1150 = case shown="0, Default" w2549 {
            tunnel: w2546 -> [_ w2557]
            tunnel: w2548 -> [w2554 w2556]
            tunnel: [w2554 w2555] -> w2547
            frame 0, Default {
            }
            frame -1 {
              n1151 = Build Array (concatenate)(w2556, w2557) -> (w2555:i32[])
            }
          }
        }
        n1152 = local read "Result files to read"() -> (w2521:path[])
        n1153 = for {
          tunnel: w2522 -> [w2545] mode=indexing
          tunnel: w2521 -> [w2544]
          tunnel: [w2541] -> w2519 mode=indexing
          n1154 = Index Array(array=w2544, index=w2545) -> (element=w2543:path)
          n1155 = Strip Path(path=w2543) -> (name=w2542:string)  [unwired: 1 out]
          n1156 = call "Add_filename_suffix.vi"("Filename"=w2542) -> ("Base name"=w2541:string)  [unwired: 1 in, 3 out]
        }
        n1157 = call "Value_Occurence_Analysis.vi"("String Array"=w2519) -> ("Output String"=w2518:string)  [unwired: 3 in, 2 out]
        n1158 = global write "Results_plotter_Global.vi" "Current Data Filenames"(w2518) -> ()
        n1159 = call "Summarise.vi"("Channel Names"=w2536, "Data"=w2531, "Summarise All"=w2530) -> ("Summary"=w2538:string[][])  [unwired: 2 in]
        n1160 = global write "Results_plotter_Global.vi" "Plot Summary"(w2538) -> ()
      }
      frame "Create summary per series" {
        n1161 = global read "Results_plotter_Global.vi" "Plot Summary"() -> (w2559:string[][])
        n1162 = local read "Plotted Series"() -> (w2561:bool[][])
        n1163 = for {
          tunnel: w2561 -> [w2578] mode=indexing
          tunnel: i32[] [] -> [w2577]
          tunnel: w2566 -> [w2575]
          tunnel: w2563 -> [w2573]
          shift-right: [w2567] -> w2558
          shift-left: w2559 -> [w2569]
          w2572 = TRUE  # Summarise All
          n1164 = for {
            shift-right: [w2586] -> w2576
            shift-left: w2577 -> [w2587]
            tunnel: w2578 -> [w2585] mode=indexing
            i -> [w2588]
            n1165 = case shown="True" w2585 {
              tunnel: w2588 -> [_ w2592]
              tunnel: w2587 -> [w2589 w2591]
              tunnel: [w2589 w2590] -> w2586
              frame False {
              }
              frame True {
                n1166 = Build Array (concatenate)(w2591, w2592) -> (w2590:i32[])
              }
            }
          }
          n1167 = for {
            tunnel: w2576 -> [w2584] mode=indexing
            tunnel: w2575 -> [w2583]
            tunnel: [w2582] -> w2574 mode=indexing
            n1168 = Index Array(array=w2583, index (row)=w2584) -> (element=w2582:string[])  [unwired: 1 in]
          }
          n1169 = call "Summarise.vi"("Channel Names"=w2573, "Data"=w2574, "Summarise All"=w2572) -> ("Summary"=w2570:string[][])  [unwired: 2 in]
          n1170 = Index Array(array=w2570, index (col)=2 ("disabled index (col)")) -> (element=w2568:string[])  [unwired: 1 in]
          n1171 = for {
            tunnel: w2569 -> [w2581] mode=indexing
            tunnel: w2568 -> [w2580] mode=indexing
            tunnel: [w2579] -> w2567 mode=indexing
            n1172 = Build Array (concatenate)(w2581, w2580) -> (w2579:string[])
          }
        }
        n1173 = global write "Results_plotter_Global.vi" "Plot Summary"(w2558) -> ()
      }
      frame "Save Intensity plot as jpg" {
        n1174 = local read "Job Directory"() -> (w2599:path)
        n1175 = global read "Constants_global.vi" "EnFlo SW Folder"() -> (w2601:path)
        n1176 = Build Path(base path=w2601, name or relative path=path "Anemometry/Anemometry Sub Vis/Data_plotting_vis/Intensity Plot Vis") -> (appended path=w2595:path)
        n1177 = call "Remote_call_prep.vi"("Vi Name in"="Create picture Vi Name", "Job Directory In"=w2599, "VI Directory"=w2595) -> ("Vi Name out"=w2597:string, "Job Directory out"=w2594:path, "cancelled"=w2593:bool)
        n1178 = local write "Create picture Vi Name"(w2597) -> ()
        n1179 = local write "Job Directory"(w2594) -> ()
        n1180 = Build Path(base path=w2595, name or relative path=w2597) -> (appended path=w2596:path)
        n1181 = case shown="False" w2593 {
          tunnel: w2596 -> [w2610 _]
          tunnel: w2594 -> [w2609 _]
          frame False {
            n1182 = Open VI Reference(type specifier VI Refnum (for type only)="type specifier VI Refnum (for type only)", vi path=w2610) -> (vi reference=w2615:refnum<vi>, error out=w2614:errorcluster)  [unwired: 2 in, 2 out]
            n1183 = property class="VI Interface Type 1"(reference=w2615, error in=w2614, "Front Panel Window:Open"=TRUE) -> (reference out=w2611:refnum<vi>, error out=w2612:errorcluster)
            n1184 = local read "Intensity Graph"() -> (w2618:dbl[][])
            n1185 = local read "No of Contours"() -> (w2608:i32)
            n1186 = call-by-ref "?"(reference=w2611, error in=w2612, "No of Contours"=w2608, "Job Directory"=w2609, "Intensity Graph"=w2618) -> (reference out=w2617:refnum<vi>, error out=w2616:errorcluster)  [unwired: 3 in]
            n1187 = Close Reference(reference=w2617, error in (no error)=w2616) -> ()  [unwired: 1 out]
          }
          frame True {
          }
        }
        n1188 = local write "Save Plot as jpg"(FALSE ("Save All data")) -> ()
      }
      frame "Run Calculation Routine" {
        n1189 = stacked-sequence {
          seq-local: [w2627 _ _] -> [_ w2637 _]
          seq-local: [w2626 _ _] -> [_ w2638 _]
          tunnel: [_ w2636 _] -> w2621
          tunnel: w2620 -> [_ _ _]
          frame #0 {
            n1190 = global read "Constants_global.vi" "EnFlo SW Folder"() -> (w2633:path)
            n1191 = Build Path(base path=w2633, name or relative path=path "Anemometry/Anemometry Sub Vis/Data_plotting_vis/Calculation Vis") -> (appended path=w2630:path)
            n1192 = local read "Job Directory"() -> (w2629:path)
            n1193 = call "Remote_call_prep.vi"("Vi Name in"="Calculate Routine", "Job Directory In"=w2629, "VI Directory"=w2630) -> ("Vi Name out"=w2631:string, "Job Directory out"=w2628:path, "cancelled"=w2627:bool)
            n1194 = local write "Calculate Routine"(w2631) -> ()
            n1195 = local write "Job Directory"(w2628) -> ()
            n1196 = Build Path(base path=w2630, name or relative path=w2631) -> (appended path=w2626:path)
          }
          frame #1 {
            n1197 = case shown="False" w2637 {
              tunnel: w2638 -> [w2646 _]
              tunnel: [w2642 w2659] -> w2636
              tunnel: "What to do next?" -> [w2641 w2659]
              frame False {
                n1198 = Open VI Reference(type specifier VI Refnum (for type only)="VI Refnum Calculation", vi path=w2646) -> (vi reference=w2652:refnum<vi>, error out=w2651:errorcluster)  [unwired: 1 in, 3 out]
                n1199 = property class="VI Interface Type 2"(reference=w2652, error in=w2651, "Front Panel Window:Open"=TRUE) -> (reference out=w2648:refnum<vi>, error out=w2649:errorcluster)
                n1200 = call-by-ref "?"(reference=w2648, error in=w2649) -> (reference out=w2654:refnum<vi>, error out=w2653:errorcluster, "New Values In"=w2639:string[][], "New Chs In"=w2647:string[])  [unwired: 2 in]
                n1201 = for {
                  tunnel: w2647 -> [w2657] mode=indexing
                  tunnel: [w2656] -> w2640 mode=indexing
                  n1202 = call "Check_Ch_Name_colons.vi"("No of Colons"=2, "Ch Name in"=w2657) -> ("Ch Name out"=w2656:string)
                }
                n1203 = Empty String/Path?(string/path=w2640) -> (empty?=w2644:bool[])
                n1204 = Or Array Elements(Boolean array=w2644) -> (logical OR=w2643:bool)
                n1205 = Close Reference(reference=w2654, error in (no error)=w2653) -> ()  [unwired: 1 out]
                n1206 = Select(t=w2641, s=w2643, f="Input calculated values") -> (s? t:f=w2642:string)
                n1207 = global write "Results_plotter_Global.vi" "New Values In"(w2639) -> ()
                n1208 = global write "Results_plotter_Global.vi" "New Chs In"(w2640) -> ()
              }
              frame True {
              }
            }
          }
          frame #2 {
            w2662 = FALSE ("Raw DF in Orig Pos?")
            n1209 = local write "Edit Raw Data Header Info"(w2662) -> ()
            n1210 = local write "Calculate new metadata"(FALSE ("Save All data")) -> ()
            n1211 = local write "Plotted rows only?"(TRUE ("Plotted rows only?")) -> ()
            n1212 = local write "Raw DF in Orig Pos?"(w2662) -> ()
            n1213 = local write "Edit Raw DF?"(w2662) -> ()
            n1214 = local write "Mode"(Plotter_Mode."Edit values per row" ("Mode")) -> ()
          }
        }
      }
      frame "Input calculated values" {
        n1215 = local read "Result files to read"() -> (w2668:path[])
        n1216 = local read "Raw DF in Orig Pos?"() -> (w2665:bool)
        n1217 = stacked-sequence {
          seq-local: [w2672 _ _ _] -> [_ w2685 w2697 _]
          seq-local: [_ w2682 _ _] -> [_ _ w2698 _]
          tunnel: [_ _ _ w2750] -> w2670
          tunnel: w2668 -> [_ _ w2699 _]
          tunnel: w2667 -> [_ _ w2696 _]
          tunnel: w2666 -> [_ _ w2695 _]
          tunnel: w2665 -> [_ _ w2694 _]
          tunnel: w2664 -> [_ _ _ w2747]
          frame #0 {
            n1218 = global read "Results_plotter_Global.vi" "Plot Index values"() -> (w2675:dbl[][])
            n1219 = global read "Results_plotter_Global.vi" "Row Reference"() -> (w2676:i32[][])
            n1220 = Index Array(array=w2675, index (row)=2) -> (element=w2673:dbl[])  [unwired: 1 in]
            n1221 = for {
              tunnel: w2676 -> [w2680]
              tunnel: w2673 -> [w2679] mode=indexing
              tunnel: [w2678] -> w2672 mode=indexing
              n1222 = Index Array(array=w2680, index (row)=w2679) -> (element=w2678:i32[])  [unwired: 1 in]
            }
            n1223 = local write "Delete Plotted data from file"(FALSE ("Save All data")) -> ()
          }
          frame #1 {
            n1224 = Index Array(array=w2685, index (col)=0 ("disabled index (col)")) -> (element=w2681:i32[])  [unwired: 1 in]
            n1225 = for {
              shift-right: [w2687] -> w2682
              shift-left: i32[] [] -> [w2688]
              tunnel: w2681 -> [w2686] mode=indexing
              n1226 = Search 1D Array(1D array=w2688, element=w2686) -> (index of element=w2689:i32)  [unwired: 1 out]
              n1227 = case shown="-1" w2689 {
                tunnel: w2688 -> [w2690 w2693]
                tunnel: [w2690 w2692] -> w2687
                tunnel: w2686 -> [_ w2691]
                frame 0, Default {
                }
                frame -1 {
                  n1228 = Build Array (concatenate)(w2693, w2691) -> (w2692:i32[])
                }
              }
            }
          }
          frame #2 {
            n1229 = for {
              tunnel: w2699 -> [w2706]
              tunnel: w2698 -> [w2703] mode=indexing
              tunnel: w2697 -> [w2704]
              tunnel: w2696 -> [w2702]
              tunnel: w2695 -> [w2701]
              tunnel: w2694 -> [w2700]
              # "New Values"
              # "Row in file"
              n1230 = Index Array(array=w2706, index=w2703) -> (element=w2705:path)
              n1231 = stacked-sequence {
                seq-local: [w2711 _] -> [_ w2745]
                seq-local: [w2709 _] -> [_ w2740]
                tunnel: w2705 -> [_ w2746]
                tunnel: w2704 -> [w2713 _]
                tunnel: w2703 -> [w2712 _]
                tunnel: w2702 -> [_ _]
                tunnel: w2701 -> [_ _]
                tunnel: w2700 -> [_ w2744]
                frame #0 {
                  n1232 = global read "Results_plotter_Global.vi" "New Values In"() -> (w2707:string[][])
                  n1233 = for {
                    tunnel: w2712 -> [w2724]
                    tunnel: w2713 -> [w2720] mode=indexing
                    shift-right: [w2718] -> w2711
                    shift-left: i32[] [] -> [w2719]
                    shift-right: [w2717] -> w2709
                    shift-left: string[][] [] -> [w2716]
                    tunnel: w2707 -> [w2715]
                    i -> [w2714]
                    n1234 = Index Array(array=w2720, index=0) -> (element=w2722:i32)
                    n1235 = Equal?(x=w2722, y=w2724) -> (x = y?=w2721:bool)
                    n1236 = case shown="True" w2721 {
                      tunnel: w2720 -> [_ w2730]
                      tunnel: w2719 -> [w2726 w2735]
                      tunnel: [w2726 w2733] -> w2718
                      tunnel: w2716 -> [w2725 w2731]
                      tunnel: [w2725 w2732] -> w2717
                      tunnel: w2715 -> [_ w2728]
                      tunnel: w2714 -> [_ w2727]
                      frame False {
                      }
                      frame True {
                        n1237 = Index Array(array=w2728, index (row)=w2727) -> (element=w2729:string[])  [unwired: 1 in]
                        n1238 = Index Array(array=w2730, index=1) -> (element=w2734:i32)
                        n1239 = Build Array (concatenate)(w2735, w2734) -> (w2733:i32[])
                        n1240 = Build Array (concatenate)(w2731, w2729) -> (w2732:string[][])
                      }
                    }
                  }
                }
                frame #1 {
                  w2739 = FALSE  # Edit all Rows?
                  w2741 = FALSE  # Edit Raw DF?
                  w2742 = FALSE  # Edit Raw Data Header Info
                  w2743 = FALSE  # Value  Constant?
                  n1241 = global read "Results_plotter_Global.vi" "New Chs In"() -> (w2737:string[])
                  n1242 = local read "Job Directory"() -> (w2738:path)
                  n1243 = call "Add_Update_Values.vi"("Filename"=w2746, "Value  Constant?"=w2743, "Edit Raw data files?"=w2741, "New Chs In"=w2737, "Edit Raw Data Header Info"=w2742, "New Values In"=w2740, "Selected Rows"=w2745, "Edit all Rows?"=w2739, "Raw DF in Orig Pos?"=w2744, "Job Directory"=w2738) -> ()  [unwired: 1 in, 5 out]
                }
              }
            }
          }
          frame #3 {
            n1244 = local read "No Of Rows"() -> (w2749:i32)
            n1245 = Less?(x=w2749, y=w2747) -> (x < y?=w2748:bool)
            n1246 = Current VI's Path() -> (path=w2751:path)
            n1247 = case shown="True" w2748 {
              tunnel: ["Create Selectors" "Initialise" ("t")] -> w2750
              frame False {
              }
              frame True {
              }
            }
            n1248 = call "Bring_to_front.vi"("path"=w2751) -> ()
          }
        }
      }
      frame "Save XY plot as jpg" {
        n1249 = local read "Create picture Vi Name"() -> (w2758:string)
        n1250 = local read "Job Directory"() -> (w2761:path)
        n1251 = global read "Constants_global.vi" "EnFlo SW Folder"() -> (w2763:path)
        n1252 = Build Path(base path=w2763, name or relative path=path "Anemometry/Anemometry Sub Vis/Data_plotting_vis/XY Plot Vis") -> (appended path=w2759:path)
        n1253 = call "Remote_call_prep.vi"("Vi Name in"=w2758, "Job Directory In"=w2761, "VI Directory"=w2759) -> ("Vi Name out"=w2760:string, "Job Directory out"=w2756:path, "cancelled"=w2755:bool)
        n1254 = local write "Create picture Vi Name"(w2760) -> ()
        n1255 = local write "Job Directory"(w2756) -> ()
        n1256 = Build Path(base path=w2759, name or relative path=w2760) -> (appended path=w2757:path)
        n1257 = case shown="False" w2755 {
          tunnel: [w2776 FALSE ("Saved Automatically?")] -> w2766
          tunnel: [w2775 path "" ("Plot data file")] -> w2765
          tunnel: [w2774 "" ("Tex Info String")] -> w2764
          tunnel: w2757 -> [w2773 _]
          tunnel: w2756 -> [w2772 _]
          frame False {
            n1258 = Open VI Reference(type specifier VI Refnum (for type only)="type specifier VI Refnum (for type only) 2", vi path=w2773) -> (vi reference=w2783:refnum<vi>, error out=w2782:errorcluster)  [unwired: 1 in, 3 out]
            n1259 = property class="VI Interface Type 3"(reference=w2783, error in=w2782, "Front Panel Window:Open"=TRUE) -> (reference out=w2779:refnum<vi>, error out=w2780:errorcluster)
            n1260 = global read "Results_plotter_Global.vi" "XY Graph Cluster"() -> (w2777:cluster{dbl[], dbl[]}[])
            n1261 = call-by-ref "?"(reference=w2779, error in=w2780, "Plot Array"=w2777, "Template"=w2772) -> (reference out=w2785:refnum<vi>, error out=w2784:errorcluster, "Saved Automatically?"=w2776:bool, "Tex Info String"=w2774:string, "Plot data file"=w2775:path)
            n1262 = Close Reference(reference=w2785, error in (no error)=w2784) -> ()  [unwired: 1 out]
          }
          frame True {
          }
        }
        n1263 = local write "Save Plot as jpg"(FALSE ("Save All data")) -> ()
        n1264 = case shown="False" w2766 {
          tunnel: w2765 -> [_ w2797]
          tunnel: [w2789 "Save Plot Data"] -> w2754
          tunnel: w2764 -> [_ w2795]
          frame False {
            n1265 = global read "Results_plotter_Global.vi" "New Chs In"() -> (w2794:string[])
            n1266 = Array Size(array=w2794) -> (size(s)=w2793:i32)
            n1267 = Greater Than 0?(x=w2793) -> (x > 0?=w2792:bool)
            n1268 = Select(t="Input calculated values", s=w2792, f="Create Selectors") -> (s? t:f=w2789:string)
          }
          frame True {
            n1269 = local write "Output Filename"(w2797) -> ()
            n1270 = local write "Header"(w2795) -> ()
          }
        }
      }
      frame "Full Res file manipulator" {
        n1271 = local read "Result files to read"() -> (w2807:path[])
        n1272 = local read "Output Filename"() -> (w2805:path)
        n1273 = local read "Mode"() -> (w2806:T1)
        n1274 = local read "Raw DF in Orig Pos?"() -> (w2801:bool)
        n1275 = local read "Plotted rows only?"() -> (w2804:bool)
        n1276 = global read "Results_plotter_Global.vi" "New Values In"() -> (w2798:string[][])
        n1277 = global read "Results_plotter_Global.vi" "New Chs In"() -> (w2799:string[])
        n1278 = stacked-sequence {
          seq-local: [w2812 _ _ _ _] -> [_ w2839 w2874 _ _]
          seq-local: [_ w2836 _ _ _] -> [_ _ w2875 _ _]
          seq-local: [_ w2833 _ _ _] -> [_ _ w2866 _ _]
          seq-local: [_ _ w2864 _ _] -> [_ _ _ w3087 _]
          seq-local: [_ _ w2863 _ _] -> [_ _ _ w3086 _]
          seq-local: [_ _ w2858 _ _] -> [_ _ _ w3083 _]
          tunnel: [_ _ _ w3090 _] -> w2809
          tunnel: w2807 -> [_ _ w2876 _ _]
          tunnel: w2806 -> [_ w2832 w2873 w3088 _]
          tunnel: w2805 -> [_ _ w2872 _ _]
          tunnel: w2804 -> [w2811 _ w2871 _ _]
          tunnel: w2799 -> [_ _ w2870 _ _]
          tunnel: w2803 -> [_ _ w2869 w3084 _]
          tunnel: w2802 -> [_ _ w2868 w3085 _]
          tunnel: w2801 -> [_ _ w2867 _ _]
          tunnel: w2800 -> [_ _ _ w3089 _]
          tunnel: w2798 -> [_ _ w2860 _ _]
          frame #0 {
            n1279 = global read "Results_plotter_Global.vi" "Row Reference"() -> (w2813:i32[][])
            n1280 = case shown="True" w2811 {
              tunnel: w2813 -> [w2815 w2816]
              tunnel: [w2815 w2817] -> w2812
              frame False {
              }
              frame True {
                n1281 = local read "Plotted Series"() -> (w2819:bool[][])
                n1282 = for {
                  tunnel: w2819 -> [w2826]
                  shift-right: [w2820] -> w2817
                  shift-left: i32[][] [] -> [w2822]
                  tunnel: w2816 -> [w2821] mode=indexing
                  i -> [w2825]
                  n1283 = Index Array(array=w2826, index (col)=w2825) -> (element=w2824:bool[])  [unwired: 1 in]
                  n1284 = Or Array Elements(Boolean array=w2824) -> (logical OR=w2823:bool)
                  n1285 = case shown="True" w2823 {
                    tunnel: w2822 -> [w2827 w2830]
                    tunnel: w2821 -> [_ w2829]
                    tunnel: [w2827 w2828] -> w2820
                    frame False {
                    }
                    frame True {
                      n1286 = Build Array (concatenate)(w2830, w2829) -> (w2828:i32[][])
                    }
                  }
                }
              }
            }
            n1287 = local write "Delete Plotted data from file"(FALSE ("Save All data")) -> ()
          }
          frame #1 {
            n1288 = local read "Job Directory"() -> (w2831:path)
            n1289 = case shown="\"Post Process Plotted Rows\"" w2832 {
              tunnel: [FALSE w2844] -> w2834
              tunnel: [w2840 w2843] -> w2833
              tunnel: w2831 -> [w2840 w2842]
              frame "Post Process Plotted Rows" {
              }
              frame "Delete unwanted rows", Default {
                n1290 = call "Remote_call_prep.vi"("Job Directory In"=w2842) -> ("Job Directory out"=w2843:path)  [unwired: 2 in, 2 out]
                n1291 = local write "Job Directory"(w2843) -> ()
                n1292 = Not Equal?(x=w2842, y=w2843) -> (x != y?=w2844:bool)
              }
            }
            n1293 = Index Array(array=w2839, index (col)=0 ("disabled index (col)")) -> (element=w2835:i32[])  [unwired: 1 in]
            n1294 = for {
              shift-right: [w2851] -> w2836
              shift-left: i32[] [] -> [w2852]
              tunnel: w2835 -> [w2850] mode=indexing
              n1295 = Search 1D Array(1D array=w2852, element=w2850) -> (index of element=w2853:i32)  [unwired: 1 out]
              n1296 = case shown="-1" w2853 {
                tunnel: w2852 -> [w2854 w2857]
                tunnel: [w2854 w2856] -> w2851
                tunnel: w2850 -> [_ w2855]
                frame 0, Default {
                }
                frame -1 {
                  n1297 = Build Array (concatenate)(w2857, w2855) -> (w2856:i32[])
                }
              }
            }
            n1298 = case shown="True" w2834 {
              tunnel: w2833 -> [_ w2846]
              frame False {
              }
              frame True {
                n1299 = local read "Template"() -> (w2845:path)
                n1300 = Path To String(path=w2846) -> (string=w2849:string)
                n1301 = call "Read_Write_Template.vi"("Template File"=w2845, "Mode"=Global_mode."Write Global to File", "Single Value In"=w2849, "Data type"="Log Folder Name" ("Variable name")) -> ()  [unwired: 4 in, 8 out]
              }
            }
          }
          frame #2 {
            w2862 = path[] []
            n1302 = local read "Full_Res_Results_Folder"() -> (w2861:path)
            n1303 = for {
              tunnel: w2876 -> [w2898]
              tunnel: w2875 -> [w2895] mode=indexing
              tunnel: w2874 -> [w2896]
              tunnel: w2873 -> [w2894]
              tunnel: w2872 -> [w2893]
              tunnel: w2871 -> [w2892]
              tunnel: w2870 -> [w2891]
              tunnel: w2869 -> [w2890]
              tunnel: w2868 -> [w2889]
              tunnel: w2867 -> [w2888]
              tunnel: w2866 -> [w2887]
              shift-right: [w2886] -> _
              shift-left: FALSE -> [w2885]
              shift-right: [w2883] -> w2864
              shift-left: w2862 -> [w2884]
              shift-right: [w2881] -> w2863
              shift-left: w2862 -> [w2882]
              tunnel: w2861 -> [w2880]
              tunnel: w2860 -> [w2879]
              shift-right: [w2877] -> w2858
              shift-left: i32[] [] -> [w2878]
              # "Row No in file"
              # "Row No in plotter"
              n1304 = Index Array(array=w2898, index=w2895) -> (element=w2897:path)
              n1305 = stacked-sequence {
                seq-local: [w2901 _ _ _] -> [_ w2929 w2978 _]
                seq-local: [_ w2927 _ _] -> [_ _ w2977 _]
                seq-local: [w2899 _ _ _] -> [_ _ w2970 w3081]
                tunnel: w2897 -> [_ w2928 w2979 _]
                tunnel: w2896 -> [w2903 _ _ _]
                tunnel: w2895 -> [w2902 _ _ _]
                tunnel: w2894 -> [_ w2926 w2976 _]
                tunnel: w2893 -> [_ _ w2975 _]
                tunnel: w2892 -> [_ _ w2974 _]
                tunnel: w2891 -> [_ _ w2973 _]
                tunnel: w2890 -> [_ _ w2972 _]
                tunnel: w2889 -> [_ _ w2971 _]
                tunnel: w2888 -> [_ _ w2969 _]
                tunnel: w2887 -> [_ _ w2968 _]
                tunnel: [_ w2925 _ _] -> w2886
                tunnel: w2885 -> [_ w2924 _ _]
                tunnel: w2884 -> [_ _ w2967 _]
                tunnel: [_ _ w2966 _] -> w2883
                tunnel: w2882 -> [_ _ w2965 _]
                tunnel: [_ _ w2964 _] -> w2881
                tunnel: w2880 -> [_ _ w2963 _]
                tunnel: w2879 -> [_ _ w2962 _]
                tunnel: w2878 -> [_ _ _ w3082]
                tunnel: [_ _ _ w3080] -> w2877
                frame #0 {
                  w2900 = i32[] []
                  n1306 = for {
                    tunnel: w2902 -> [w2912]
                    tunnel: w2903 -> [w2908] mode=indexing
                    shift-right: [w2906] -> w2901
                    shift-left: w2900 -> [w2907]
                    shift-right: [w2905] -> w2899
                    shift-left: w2900 -> [w2904]
                    n1307 = Index Array(array=w2908, index=0) -> (element=w2910:i32)
                    n1308 = Equal?(x=w2910, y=w2912) -> (x = y?=w2909:bool)
                    n1309 = case shown="True" w2909 {
                      tunnel: w2908 -> [_ w2916]
                      tunnel: w2907 -> [w2914 w2922]
                      tunnel: [w2914 w2920] -> w2906
                      tunnel: w2904 -> [w2913 w2918]
                      tunnel: [w2913 w2919] -> w2905
                      frame False {
                      }
                      frame True {
                        n1310 = Index Array(array=w2916, index=2) -> (element=w2915:i32)
                        n1311 = Build Array (concatenate)(w2918, w2915) -> (w2919:i32[])
                        n1312 = Index Array(array=w2916, index=1) -> (element=w2921:i32)
                        n1313 = Build Array (concatenate)(w2922, w2921) -> (w2920:i32[])
                      }
                    }
                  }
                }
                frame #1 {
                  n1314 = case shown="\"Post Process Plotted Rows\"" w2926 {
                    tunnel: w2929 -> [_ _ _ _ _ w2945]
                    tunnel: w2928 -> [_ _ _ _ _ w2943]
                    tunnel: [TRUE ("T button?") TRUE ("T button?") TRUE ("T button?") TRUE ("T button?") TRUE ("T button?") w2942] -> w2927
                    tunnel: [w2930 w2932 w2934 w2936 w2938 w2941] -> w2925
                    tunnel: w2924 -> [w2930 w2932 w2934 w2936 w2938 w2940]
                    frame "Save file" {
                    }
                    frame "Edit values per row" {
                    }
                    frame "Edit Values with constants" {
                    }
                    frame "Edit Raw Data file header" {
                    }
                    frame "Post Process Plotted Rows" {
                    }
                    frame "Delete unwanted rows" {
                      n1315 = Array Size(array=w2945) -> (size(s)=w2944:i32)
                      n1316 = case shown="True" w2940 {
                        tunnel: w2944 -> [w2954 _]
                        tunnel: w2943 -> [w2953 _]
                        tunnel: [w2948 w2961] -> w2942
                        tunnel: [w2947 w2961] -> w2941
                        frame False {
                          n1317 = Format Into String(format string="Remove %d rows from \"%s\"", w2954, w2953) -> (resulting string=w2951:string)  [unwired: 2 in, 1 out]
                          n1318 = call <vilib>:"Three Button Dialog.vi"("Allow user to close window? (TRUE)"=TRUE, "Right Button Text (\"Cancel\")"="Yes To All Files" ("Right Button Text (\"Cancel\")"), "message"=w2951) -> ("Which Button?"=w2949:T11)  [unwired: 3 in, 5 out]
                          n1319 = case shown="\"Left Button\"" w2949 {
                            tunnel: [TRUE TRUE w2959 w2960] -> w2948
                            tunnel: [FALSE TRUE w2959 w2960] -> w2947
                            frame "Left Button" {
                            }
                            frame "Right Button" {
                            }
                            frame "Center Button" {
                              w2959 = FALSE
                            }
                            frame "Window Close" {
                              w2960 = FALSE
                            }
                          }
                        }
                        frame True {
                          w2961 = TRUE
                        }
                      }
                    }
                  }
                }
                frame #2 {
                  n1320 = case shown="True" w2977 {
                    tunnel: w2979 -> [_ w2998]
                    tunnel: w2978 -> [_ w2997]
                    tunnel: w2976 -> [_ w2996]
                    tunnel: w2975 -> [_ w2995]
                    tunnel: w2974 -> [_ w2994]
                    tunnel: w2973 -> [_ w2993]
                    tunnel: w2972 -> [_ w2992]
                    tunnel: w2971 -> [_ w2991]
                    tunnel: w2970 -> [_ w2990]
                    tunnel: w2969 -> [_ w2989]
                    tunnel: w2968 -> [_ w2988]
                    tunnel: w2967 -> [w2981 w2987]
                    tunnel: [w2981 w2986] -> w2966
                    tunnel: w2965 -> [w2980 w2985]
                    tunnel: [w2980 w2984] -> w2964
                    tunnel: w2963 -> [_ w2983]
                    tunnel: w2962 -> [_ w2982]
                    frame False {
                    }
                    frame True {
                      n1321 = case shown="\"Edit Raw Data file header\", Default" w2996 {
                        tunnel: w2998 -> [w3004 w3009 w3038 w3051 w3068]
                        tunnel: w2997 -> [w3007 w3020 w3037 w3050 w3067]
                        tunnel: w2995 -> [_ _ _ _ _]
                        tunnel: w2994 -> [_ _ _ w3048 w3065]
                        tunnel: w2993 -> [_ _ _ w3046 w3063]
                        tunnel: w2992 -> [_ _ _ _ w3062]
                        tunnel: w2991 -> [_ _ _ _ w3060]
                        tunnel: w2990 -> [_ _ _ _ w3059]
                        tunnel: w2989 -> [_ _ _ w3045 w3057]
                        tunnel: w2988 -> [_ _ _ w3043 w3055]
                        tunnel: w2987 -> [w3006 w3013 w3036 w3041 w3053]
                        tunnel: [w3006 w3014 w3036 w3041 w3053] -> w2986
                        tunnel: w2985 -> [w3005 w3012 w3035 w3040 w3052]
                        tunnel: [w3005 w3010 w3035 w3040 w3052] -> w2984
                        tunnel: w2983 -> [w3003 _ _ _ _]
                        tunnel: w2982 -> [_ _ _ w3039 _]
                        frame "Save file" {
                          n1322 = Strip Path(path=w3004) -> (name=w3001:string)  [unwired: 1 out]
                          n1323 = call "Add_filename_suffix.vi"("Filename"=w3001, "Suffix to add"=".xls") -> ("Filename out"=w2999:string)  [unwired: 3 out]
                          n1324 = Build Path(base path=w3003, name or relative path=w2999) -> (appended path=w3002:path)
                          n1325 = call "Save_full_Res_rows.vi"("Selected Rows"=w3007, "Filename to write"=w3002, "Filename Orig"=w3004) -> ()  [unwired: 2 out]
                        }
                        frame "Edit Raw Data file header", Default {
                          w3025 = FALSE  # Add Extra Channels?
                          w3024 = FALSE  # Read Channel Names only
                          n1326 = global read "Constants_global.vi" "Run VI Folder"() -> (w3019:path)
                          n1327 = Strip Path(path=w3019) -> (stripped path=w3018:path)  [unwired: 1 out]
                          n1328 = Build Path(base path=w3018, name or relative path="Data_plotting_vis") -> (appended path=w3017:path)
                          n1329 = Build Path(base path=w3017, name or relative path="RD_Files.tpt") -> (appended path=w3023:path)
                          n1330 = call "Read_Data_file.vi"("Results file"=w3009, "Read Channel Names only"=w3024, "Add Extra Channels?"=w3025, "Template File"=w3023) -> ("Row numbers"=w3008:i32[], "Channel Values Out"=w3026:string[][])  [unwired: 1 in, 13 out]
                          n1331 = Index Array(array=w3026, index (col)=0 ("index (row)")) -> (element=w3021:string[])  [unwired: 1 in]
                          n1332 = for {
                            tunnel: w3021 -> [w3034]
                            tunnel: w3020 -> [w3028] mode=indexing
                            tunnel: [w3032] -> w3015 mode=indexing
                            tunnel: [w3031] -> w3011 mode=indexing
                            tunnel: w3009 -> [w3031]
                            tunnel: w3008 -> [w3030]
                            n1333 = Search 1D Array(1D array=w3030, element=w3028) -> (index of element=w3029:i32)  [unwired: 1 in]
                            n1334 = Index Array(array=w3034, index=w3029) -> (element=w3033:string)
                            n1335 = call "String_to_Pathname.vi"("Input String"=w3033) -> ("path"=w3032:path)
                          }
                          n1336 = Build Array (concatenate)(w3012, w3011) -> (w3010:path[])
                          n1337 = Build Array (concatenate)(w3013, w3015) -> (w3014:path[])
                        }
                        frame "Delete unwanted rows" {
                          n1338 = call "Delete_unwanted_rows.vi"("Selected Rows"=w3037, "Filename"=w3038) -> ()  [unwired: 1 out]
                        }
                        frame "Edit Values with constants" {
                          w3049 = TRUE  # Value  Constant?
                          n1339 = local read "Edit Raw Data Header Info"() -> (w3042:bool)
                          n1340 = local read "Edit Raw DF?"() -> (w3044:bool)
                          n1341 = Not(x=w3048) -> (.not. x?=w3047:bool)
                          n1342 = call "Add_Update_Values.vi"("Filename"=w3051, "Value  Constant?"=w3049, "Edit Raw data files?"=w3044, "New Chs In"=w3046, "Edit Raw Data Header Info"=w3042, "New Values In"=w3039, "Selected Rows"=w3050, "Edit all Rows?"=w3047, "Raw DF in Orig Pos?"=w3045, "Job Directory"=w3043) -> ()  [unwired: 1 in, 5 out]
                        }
                        frame "Edit values per row" {
                          w3054 = FALSE  # Edit Raw Data Header Info
                          w3066 = FALSE  # Value  Constant?
                          n1343 = for {
                            tunnel: w3063 -> [w3079] mode=indexing
                            tunnel: w3062 -> [w3078]
                            tunnel: [w3077] -> w3061 mode=indexing
                            n1344 = Search 1D Array(1D array=w3078, element=w3079) -> (index of element=w3077:i32)  [unwired: 1 out]
                          }
                          n1345 = for {
                            tunnel: w3061 -> [w3073]
                            tunnel: w3060 -> [w3072]
                            tunnel: w3059 -> [w3070] mode=indexing
                            tunnel: [w3069] -> w3058 mode=indexing
                            n1346 = Index Array(array=w3072, index (row)=w3070) -> (element=w3071:string[])  [unwired: 1 in]
                            n1347 = for {
                              tunnel: w3073 -> [w3076] mode=indexing
                              tunnel: w3071 -> [w3075]
                              tunnel: [w3074] -> w3069 mode=indexing
                              n1348 = Index Array(array=w3075, index=w3076) -> (element=w3074:string)
                            }
                          }
                          n1349 = Not(x=w3065) -> (.not. x?=w3064:bool)
                          n1350 = local read "Edit Raw DF?"() -> (w3056:bool)
                          n1351 = call "Add_Update_Values.vi"("Filename"=w3068, "Value  Constant?"=w3066, "Edit Raw data files?"=w3056, "New Chs In"=w3063, "Edit Raw Data Header Info"=w3054, "New Values In"=w3058, "Selected Rows"=w3067, "Edit all Rows?"=w3064, "Raw DF in Orig Pos?"=w3057, "Job Directory"=w3055) -> ()  [unwired: 1 in, 5 out]
                        }
                      }
                    }
                  }
                }
                frame #3 {
                  n1352 = Build Array (concatenate)(w3082, w3081) -> (w3080:i32[])
                }
              }
            }
          }
          frame #3 {
            n1353 = case shown="\"Post Process Plotted Rows\"" w3088 {
              tunnel: ["Create Selectors" w3098 "Initialise" ("t") w3157] -> w3090
              tunnel: w3089 -> [_ _ _ w3154]
              tunnel: w3087 -> [w3091 w3097 _ _]
              tunnel: w3086 -> [_ w3096 _ _]
              tunnel: w3085 -> [_ w3095 _ _]
              tunnel: w3084 -> [_ w3094 _ _]
              tunnel: w3083 -> [_ w3093 _ _]
              frame "Edit Raw Data file header" {
                n1354 = call "Edit_Raw_DF_Header.vi"("Selected files"=w3091) -> ()  [unwired: 15 out]
              }
              frame "Post Process Plotted Rows" {
                n1355 = stacked-sequence {
                  seq-local: [w3100 _ _] -> [_ w3124 _]
                  seq-local: [w3099 _ _] -> [_ _ w3149]
                  seq-local: [_ w3121 _] -> [_ _ w3148]
                  tunnel: [_ _ "Create Selectors"] -> w3098
                  tunnel: w3097 -> [_ _ w3151]
                  tunnel: w3096 -> [_ _ w3150]
                  tunnel: w3095 -> [_ w3123 _]
                  tunnel: w3094 -> [w3101 _ _]
                  tunnel: w3093 -> [_ w3120 _]
                  frame #0 {
                    n1356 = global read "Results_plotter_Global.vi" "Dispose"() -> (w3103:string[])
                    n1357 = for {
                      tunnel: w3103 -> [w3112] mode=indexing
                      shift-right: [w3108] -> w3100
                      shift-left: i32[] [] -> [w3110]
                      i -> [w3109]
                      n1358 = String Subset(string=w3112, length (rest)=1 ("length (rest)")) -> (substring=w3114:string)  [unwired: 1 out]
                      n1359 = Equal?(x="T", y=w3114) -> (x = y?=w3111:bool)
                      n1360 = case shown="False" w3111 {
                        tunnel: w3110 -> [w3118 w3119]
                        tunnel: [w3117 w3119] -> w3108
                        tunnel: w3109 -> [w3116 _]
                        frame False {
                          n1361 = Build Array (concatenate)(w3118, w3116) -> (w3117:i32[])
                        }
                        frame True {
                        }
                      }
                    }
                    n1362 = for {
                      tunnel: w3101 -> [w3107]
                      tunnel: w3100 -> [w3106] mode=indexing
                      tunnel: [w3105] -> w3099 mode=indexing
                      n1363 = Index Array(array=w3107, index=w3106) -> (element=w3105:string)
                    }
                    n1364 = local write "Post Process Plotted Data"(FALSE ("Post Process Plotted Data")) -> ()
                  }
                  frame #1 {
                    n1365 = global read "Results_plotter_Global.vi" "Precision"() -> (w3122:string[])
                    n1366 = for {
                      tunnel: w3124 -> [w3130]
                      tunnel: w3123 -> [w3126]
                      tunnel: w3122 -> [w3129]
                      tunnel: [w3128] -> w3121 mode=indexing
                      tunnel: w3120 -> [w3127] mode=indexing
                      n1367 = Index Array(array=w3126, index (row)=w3127) -> (element=w3125:string[])  [unwired: 1 in]
                      n1368 = for {
                        tunnel: w3130 -> [w3140] mode=indexing
                        tunnel: w3125 -> [w3142]
                        tunnel: w3129 -> [w3141]
                        tunnel: [w3134] -> w3128 mode=indexing
                        n1369 = Index Array(array=w3142, index=w3140) -> (element=w3133:string)
                        n1370 = Index Array(array=w3141, index=w3140) -> (element=w3132:string)
                        n1371 = Fract/Exp String To Number(string=w3133) -> (offset past number=w3138:i32, number=w3135:dbl)  [unwired: 3 out]
                        n1372 = String Length(string=w3133) -> (length=w3139:i32)
                        n1373 = Equal?(x=w3139, y=w3138) -> (x = y?=w3136:bool)
                        n1374 = Empty String/Path?(string/path=w3133) -> (empty?=w3137:bool)
                        n1375 = Compound Arithmetic op=AND(invert w3137, w3136) -> (w3131:bool)
                        n1376 = case shown="True" w3131 {
                          tunnel: w3132 -> [_ w3145]
                          tunnel: w3135 -> [_ w3146]
                          tunnel: [w3143 w3144] -> w3134
                          tunnel: w3133 -> [w3143 _]
                          frame False {
                          }
                          frame True {
                            n1377 = call "Number_2_string.vi"("precision"=w3145, "number"=w3146) -> ("String"=w3144:string)
                          }
                        }
                      }
                    }
                  }
                  frame #2 {
                    n1378 = Build Array (concatenate)(w3149, w3148) -> (w3147:string[][])
                    n1379 = call "Post_Process_Profile_Remote.vi"("Results Plotter Rows"=w3147, "Raw Data files to PP"=w3151, "Current Results filenames"=w3150) -> ()  [unwired: 1 out]
                  }
                }
              }
              frame "Delete unwanted rows" {
              }
              frame "Edit Values with constants", Default {
                n1380 = local read "No Of Rows"() -> (w3156:i32)
                n1381 = Less?(x=w3156, y=w3154) -> (x < y?=w3155:bool)
                n1382 = case shown="False" w3155 {
                  tunnel: ["Create Selectors" "Initialise" ("t")] -> w3157
                  frame False {
                  }
                  frame True {
                  }
                }
              }
            }
          }
          frame #4 {
            n1383 = Current VI's Path() -> (path=w3160:path)
            n1384 = call "Bring_to_front.vi"("path"=w3160) -> ()
          }
        }
      }
      frame "End" {
        n1385 = local read "Template"() -> (w3162:path)
        n1386 = local read "Empty"() -> (w3163:bool)
        n1387 = call "Valid_Path.vi"("Filename"=w3162) -> ("Valid Path?"=w3161:bool)
        n1388 = case shown="True" w3163 {
          frame False {
          }
          frame True {
            n1389 = property on="Result files to read" class="Arr (strict)"("Index Values"=u32[] [0] ("Write Attribute")) -> ()  [unwired: 2 in, 2 out]
            n1390 = local write "Result files to read"(path[] [] ("Result files to read")) -> ()
            n1391 = local write "Empty"(FALSE ("Empty")) -> ()
          }
        }
        n1392 = case shown="False" w3161 {
          tunnel: w3164 -> [w3173 _]
          frame False {
            n1393 = local write "Template"(w3173) -> ()
          }
          frame True {
          }
        }
      }
      frame "Empty Results file array" {
        n1394 = local read "Template"() -> (w3175:path)
        n1395 = call "Valid_Path.vi"("Filename"=w3175) -> ("Valid Path?"=w3174:bool)
        n1396 = case shown="True" w3174 {
          tunnel: w3176 -> [w3185 _]
          frame False {
            n1397 = local write "Template"(w3185) -> ()
          }
          frame True {
          }
        }
        n1398 = property on="Result files to read" class="Arr (strict)"("Index Values"=u32[] [0] ("Write Attribute")) -> ()  [unwired: 2 in, 2 out]
        n1399 = local write "Result files to read"(path[] [] ("Result files to read")) -> ()
        n1400 = local write "Empty"(FALSE ("Empty")) -> ()
      }
      frame "Save Setup" {
        w3190 = "Current_Setup.xls" ("Setup filename")
        n1401 = local read "Create picture Vi Name"() -> (w3205:string)
        n1402 = local read "Additional X Values"() -> (w3211:dbl[])
        n1403 = local read "Additional Y Values"() -> (w3210:dbl[])
        n1404 = local read "Result files to read"() -> (w3213:path[])
        n1405 = local read "Output Filename"() -> (w3206:path)
        n1406 = local read "Intensity Plot?"() -> (w3204:bool)
        n1407 = local read "Multi Ordinate?"() -> (w3203:bool)
        n1408 = local read "Multi Ordinate"() -> (w3199:i32[])
        n1409 = local read "Filter Array"() -> (w3207:u16[])
        n1410 = local read "Transpose"() -> (w3212:bool)
        n1411 = local read "Template"() -> (w3191:path)
        n1412 = local read "Filter Bins 2"() -> (w3200:i32[])
        n1413 = local read "Ordinate"() -> (w3209:u16)
        n1414 = local read "Filter Bins 1"() -> (w3201:i32[])
        n1415 = local read "Absisca"() -> (w3208:u16)
        n1416 = call "Read_Write_Plot_Setup.vi"("Mode"=enum16{"Load", "Save"}."Load", "Setup filename"=w3190) -> ("Cluster 2"=w3214:T10)  [unwired: 1 in, 1 out]
        n1417 = Bundle By Name(cluster=w3214, "Result files to read"=w3213, "Template"=w3191, "Transpose"=w3212, "Additional X Values"=w3211, "Additional Y Values"=w3210, "Ordinate"=w3209, "Absisca"=w3208, "Filter Array"=w3207, "color and symbol"=TRUE, "Output Filename"=w3206, "Jpg Vi Name"=w3205, "Intensity Plot?"=w3204, "Multi Ordinate?"=w3203, "Filter Bins 1"=w3201, "Filter Bins 2"=w3200, "Multi Ordinate"=w3199) -> (w3202:T10)
        n1418 = local read "Save Setup"() -> (w3189:bool)
        n1419 = local read "stop"() -> (w3197:bool)
        n1420 = Not(x=w3197) -> (.not. x?=w3196:bool)
        n1421 = Path To String(path="Job Directory") -> (string=w3195:string)
        n1422 = call "Read_Write_Plot_Setup.vi"("Mode"=enum16{"Load", "Save"}."Save", "Setup filename"=w3190, "Cluster"=w3202) -> ()  [unwired: 2 out]
        n1423 = call "Read_Write_Template.vi"("Template File"=w3191, "Mode"=Global_mode."Write Global to File", "Single Value In"=w3195, "Data type"="Log Folder Name" ("Variable name")) -> ()  [unwired: 4 in, 8 out]
        n1424 = Select(t="Save to named setup file", s=w3189, f="Check modification dates?") -> (s? t:f=w3187:string)
      }
      frame "Save to named setup file" {
        w3221 = TRUE  # Save New File?
        n1425 = call "Save_current_setup.vi"("Save New File?"=w3221, "Setup File Type"=Setup_Filetype."Results File Plotter Setups") -> ()  [unwired: 4 out]
        n1426 = local write "Save Setup"(FALSE ("Save Setup")) -> ()
      }
    }
    "Current" <- w11
  }
